vi "Tracker_2.2+.vi"(8 "error in (no error)":errorcluster, 11 "Settings file path":path=path "D:/Users/Dmitriy/CData/CloudStation/Tracker_repository/SubVi's/Tracker_settings.tcf") -> (0 "error out":errorcluster)   [LabVIEW 2018]
uses:
  <vilib>/Utility/miscctls.llb/LVPointTypeDef.ctl
  <vilib>/Utility/config.llb/NI_LVConfig.lvlib
  SubVi's/SW_Globals.vi
  <vilib>/Utility/file.llb/Write Delimited Spreadsheet (string).vi
  <vilib>/Utility/miscctls.llb/LVRangeTypeDef.ctl
  <extravilib>/ChannelInstances/Lossy Stream-a[.,.](str).lvlib
  <vilib>/Instr/_visa.llb/VISA Flush IO Buffer Mask.ctl
  <vilib>/Utility/miscctls.llb/LVBoundsTypeDef.ctl
  <vilib>/Utility/miscctls.llb/LVOffsetAndMultiplierTypeDef.ctl
  <vilib>/platform/TimedLoop/XDataNode/XDataNode.xnode
  <vilib>/Platform/TimedLoop/XDataNode/nitl_modes.ctl
  <vilib>/Platform/TimedLoop/XDataNode/XDNodeRunTimeDep.lvlib
  <vilib>/Platform/TimedLoop/XDataNode/wakeup.ctl
  <vilib>/Platform/TimedLoop/XDataNode/timing_clust.ctl
  <vilib>/Analysis/NI_AALBase.lvlib
  <vilib>/Instr/_visa.llb/VISA Open Access Mode.ctl
  <vilib>/Utility/sysdir.llb/System Directory Type.ctl
  <vilib>/ChannelSupport/Lossy Behavior.ctl
  <extravilib>/ChannelInstances/Stream-a[.](str).lvlib
  <vilib>/Utility/file.llb/Write Delimited Spreadsheet (I64).vi
  <vilib>/Platform/TimedLoop/scheduler/LVUserAPI/_suppVIs/Create_1kHz_TSource.vi
  <vilib>/Utility/file.llb/Read Delimited Spreadsheet (string).vi
  <vilib>/Utility/config.llb/Config Data RefNum.ctl
  <vilib>/Utility/miscctls.llb/LVPoint32TypeDef.ctl
  SubVi's/CTL_Data_flow_control_cluster.ctl
panel:
  out "Timed structure (Streaming) and VISA error(s)":errorcluster
  out "VISA streaming error out":errorcluster
  out "Latest frame":string[](array[string])
  out "Serial port opened":bool
  in  "Open serial port":bool
  out "FP size change error":errorcluster
  out "FPS status":i32=80
  out "Data flow controls":T1
  in  "Streaming":bool
  out "write status":bool
  out "Last send packet size, bytes":u32
  out "PP status":string
  out "DAQ status":string
  out "Stop TTL is fired":bool
  out "Start TTL is fired":bool
  out "IO paramaters loaded from file":bool
  out "IO parameters loaded cluster":T2
  out "Settings load path":path caption="selected path"
  in  "\"Stop at\" enabled":bool
  in  "Serial OUT name":refnum<visa-resource-name>="Serial_Output"
  out "Output to the external terminal":string="00:00:00.000\t0.000000\t0.000000\t0.000000\t0.000000\t00.000000\t0.000000\t0\t0.000\r\n"
  in  "Twisted neck":bool
  in  "Bridge horizontal offset":sgl min=-70 max=70 step=0.1 format="%#.1g"
  in  "Name Prefix":string="SavedTrack"
  in  "Stop record at":dbl=600.0 caption="Stop at" min=0.0 max=43200.0 step=60.0 format="%<%H:%M:%S>t"
  out "Adv. Stim. set":bool
  in  "Save files First Call":bool=TRUE
  in  "Record start First Call":bool=TRUE
  out "Time per sample mean":dbl format="%0.2f"
  out "Time per sample SD":dbl format="%0.2f"
  out "Save iteration duration":i64
  out "standard deviation":dbl format="%0.2f"
  out "mean":dbl format="%0.2f"
  in  "Type of histogram":u8
  out "TTL 4 counter":u32
  out "TTL 3 counter":u32
  out "TTL 2 counter":u32
  out "TTL 1 counter":u32
  out "Full track plotting":u32
  out "Full track preparation":u32
  out "Main queue":refnum<queue>
  in  "Map index (analysis)":i32
  in  "Full trace color":u32(colorbox)=16711680
  out "Current TTL status":u8
  out "TTL inputs":u8[](array[numeric])
  out "TTL outputs":u8[](array[numeric])
  out "Start/Stop in config":u32
  out "Start/Stop out pulses config":u32
  out "Changed IO":bool
  out "Sync capability":u8
  in  "IO parameters string":string
  out "Reset STIM":bool
  out "Reset REG":bool
  out "Init plot":bool=TRUE
  out "Zones preference array (loaded)":dbl[][](array[numeric])
  out "Current zone":dbl[](array[numeric])
  out "Absolute timestamp (rec)":dbl[](array[numeric])
  in  "Colors for Stim. setup":T3(array[cluster])=[{"Not Selected"=1143775, "Not Selected"=1143775}, {"Not Selected"=14517504, "Not Selected"=14517504}, {"Not Selected"=1976113, "Not Selected"=1976113}, {"Not Selected"=2575993, "Not Selected"=2575993}]
  out "Record":bool
  out "Stopped":bool
  out "Reset starting pulse":bool
  out "TTL is long enough":bool
  out "Started":bool
  out "Coords":T4={"Horizontal"=316, "Vertical"=127}
  out "Button":u16=1
  out "Settings file path":path
  out "Track path":path
  out "Index of the last recorded timepoint":i32
  out "ceil(x): smallest int >= x":dbl
  out "Application Directory":path
  out "Path to the settings file":path=path "D:/Users/Dmitriy/CData/CloudStation/Tracker_repository/Tracker_settings.tcf"
  out "Eff. save interval":sgl=7.981
  out "Relative timestamp (rec)":dbl[](array[numeric])
  out "alpha rot. angle":dbl[](array[numeric])
  out "Y coord":dbl[](array[numeric])
  out "X coord":dbl[](array[numeric])
  out "Zones allocation array":i32[](array[numeric])
  out "Zones presence array":bool[](array[boolean])
  in  "Stop Button":bool
  out "Path to the latest saved temp file":path
  out "Temp file ready":bool
  out "Pixels per mm":dbl=1.1663076923076923
  out "Settings file refnum out":T5
  out "Current User":string="Researcher"
  in  "Main tab control":enum32{"Settings", "Recording", "Analysis"}(tab)
  in  "Set advanced stimulus":bool
  in  "Load settings":bool
  out "IO status indicator":T6
  in  "Set IO config":bool
  in  "Jump to Analysis":bool
  in  "Reset stimuli":bool
  in  "Stimulus presets":T7(array[cluster]) {"TTL out" items=["1"=1, "2"=2, "1 + 2"=3]; "Stimulus, s" min=0 max=10000 step=0.1; "Time, s" min=0 max=10000 step=0.1; "Event type" items=["Time spent in zone", "Future options"]}
  in  "Zone-based stimulus setup":T8(radio)=enum."Zone 13"
  out "Ready":bool=TRUE
  in  "Re-check HW connection":bool
  in  "Reset regions":bool
  in  "Start Tracking button":bool
  in  "Starting angle BORDER":i16
  in  "N segments BORDER":u8=5 min=1 max=12
  in  "N segments MIDFIELD":u8=3 max=8
  in  "Starting angle MIDFIELD":i16=30
  in  "Radius, mm MIDFIELD":u16=110
  in  "Radius, mm CENTER":u16=50 min=5 step=1
  out "Board size":string="Large"
  in  "Cage diameter, mm":u16(ring)=333 items=["180 mm"=180, "240 mm"=240, "290 mm"=290, "325 mm"=325, "327 mm"=327, "333 mm"=333]
  out "Segments diagram":picture
  out "HW info":string
  out "Port":string="Large"
  in  "Expand/hide stream panel (Set)":bool
  out "Run times distrib. indicator":bool
  out "IO pulses count":string
  in  "Bridge swap":bool
  in  "Reset barplot":bool
  out "Mouse speed digi":dbl=0.28949046360238656 caption="Mouse speed" format="%05.1f"
  out "Histograms (normalized)":dbl[](graph)=[0.0, 0.0, 0.0, 0.0, 0.0, 0.0, 0.0, 1.0, 0.0, 0.0, 0.0, 0.0, 0.0, 0.0] caption="Zone preference (normalized)"
  in  "Multiplyer of chart RX":u8(slide)=1 min=1 max=10 step=1 scale=1.0..6.0
  in  "Zones presence indicator":T9={"01"=TRUE, "02"=TRUE, "03"=TRUE, "04"=TRUE, "05"=TRUE, "06"=TRUE, "07"=TRUE, "08"=TRUE, "09"=TRUE, "10"=TRUE, "11"=TRUE, "12"=TRUE, "13"=TRUE}
  in  "Zones":bool=TRUE
  in  "Record/Stop":bool
  out "Diagram at recording":picture caption="Mouse track"
  in  "Trace, s":u16(slide)=5 max=30 step=1 scale=0.0..30.0
  in  "Data filtering":u16(ring)=5 items=["None"=0, "Kalman 1/3"=2, "Kalman 1/8"=3, "SG 3/5"=4, "SG 3/11"=5, "SG 3/31"=6]
  out "Record timestamp":dbl format="%<%H:%M:%S%3u>t"
  out "Current Time":timestamp=timestamp(3610093053.229 s since 1904-01-01) format="%<%H:%M:%S %d.%m.%Y>T"
  in  "Exit (recording)":bool
  out "Mouse speed":waveform(dbl)(graph)={"t0"=timestamp(3610093053.229 s since 1904-01-01), "dt"=1.0, "Y"=[0.28949046360238656]}
  in  "Bridge offset":sgl min=-70 max=70 step=0.1 format="%#.1g"
  out "TTL IO 1 (recording)":bool caption="IO 1"
  out "TTL IO 2 (recording)":bool caption="IO 2"
  out "TTL IO 3 (recording)":bool caption="IO 3"
  out "TTL IO 4 (recording)":bool caption="IO 4"
  out "TTL REC":bool
  out "Mouse running, perc. of time":dbl=0.28949046360238656 caption="Run, %" format="%05.2f"
  out "Zones presense indicator":bool=TRUE
  out "Speed distrib. indicator":bool
  out "Run lengts distrib. indicator":bool
  in  "Additional record settings":bool caption="Add. recording settings"
  in  "Expand/hide stream panel (Rec)":bool
  in  "Back to Settings":bool
  out "Data loading progress":dbl(slide) scale=0.0..100.0
  in  "Speed":u16(ring)=3 items=["25"=75, "10"=30, "6"=18, "4"=12, "2"=6, "1"=3, "2/3"=2, "1/3"=1]
  in  "Timeline":dbl(slide) min=0.0 step=1.0 scale=0.0..2351.728 scale format="%<%H:%M:%S>t"
  in  "Multiplyer of chart RX 2":u8(slide)=1 min=1 max=10 step=1 scale=1.0..6.0
  out "Diagram at analysis":picture caption="Mouse track"
  in  "Play/Pause":bool
  out "Recorded at time":timestamp format="%<%H:%M:%S %d.%m.%Y>T"
  out "Recorded timestamp":dbl format="%<%H:%M:%S%3u>t"
  in  "Zones (analysis)":bool=TRUE caption="Zones"
  out "Mouse speed 2":waveform(dbl)(graph) caption="Mouse speed"
  out "Mouse speed digi 2":dbl format="%05.1f"
  out "Zones allocation (normalized) in analysis":dbl[](graph) caption="Zone preference (normalized)"
  out "Recorded by":string
  in  "Trace in analysis, s":u16(slide)=2 caption="Trace, s" max=30 step=1 scale=0.0..30.0
  in  "Open File":bool
  out "Bridge swap (analysis)":bool caption="Swapped"
  in  "Show heatmap (analysis)":bool caption="Heat map"
  in  "Show full track (analysis)":bool caption="Full track"
  out "Bridge Vertical offset (analysis)":sgl caption="Br. offset" min=-60 max=60 step=0.1 format="%#.1g"
  out "TTL IO 2 (analysis)":bool
  out "TTL IO 1 (analysis)":bool
  out "TTL IO 3 (analysis)":bool
  out "TTL IO 4 (analysis)":bool
  in  "Expand/hide stream panel (An)":bool
  # "v.2.1.9.9"
  # "Cage segmentation"
  # "BORDER"
  # "CENTER"
  # "MIDFIELD"
  # "v.2.1.9.9"
  # "v.2.1.9.9"
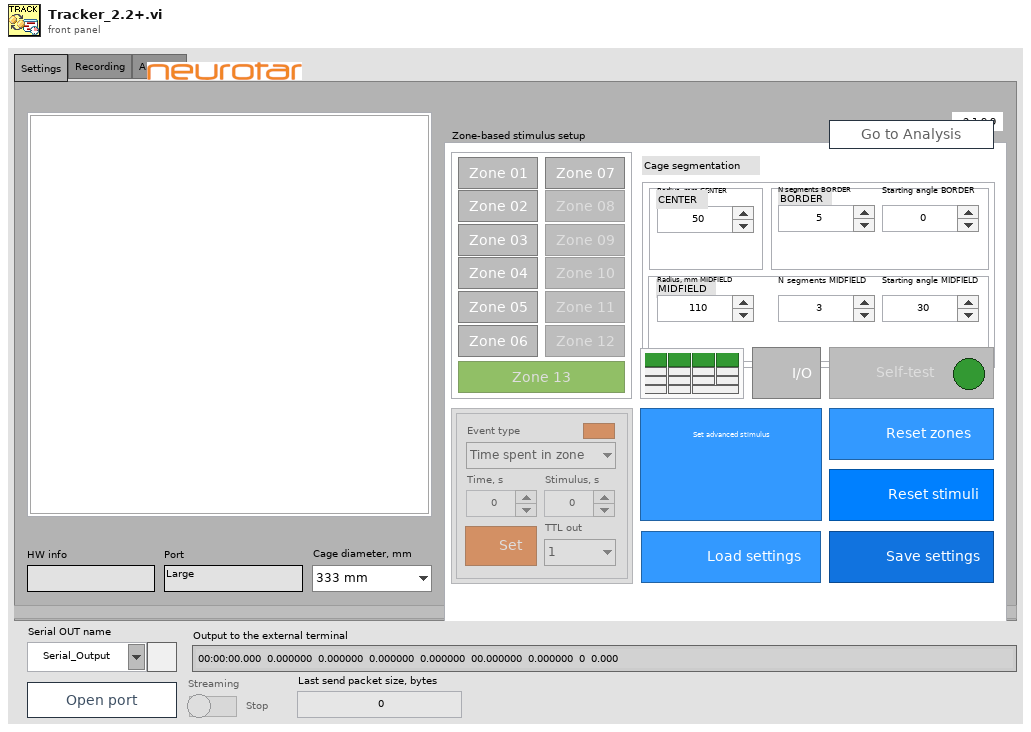
[diagram p1: front panel]
types:
  T1 = typedef "CTL_Data_flow_control_cluster.ctl" = cluster{"Data acquisition status":refnum<notifier>, "Play/Pause status":refnum<notifier>, "Complete stop":refnum<notifier>, "Temp file ready for processing":refnum<notifier>, "Has been recorded":refnum<notifier>, "Recording now":refnum<notifier>, "Path to the latest complete temp file":refnum<notifier>, "(Final) Data file is saved":refnum<notifier>, "Data loaded":refnum<notifier>}
  T2 = cluster{"SYNC configuration":u16, "IO 1 configuration":u16, "IO 2 configuration":u16, "IO 3 configuration":u16, "IO 4 configuration":u16, "Activate ext. RS-232":u16, "IO inversion config.":u16}
  T3 = cluster{"Not Selected":u32, "Not Selected":u32}[]
  T4 = typedef "LVPoint32TypeDef.ctl" = cluster{"Horizontal":i32, "Vertical":i32}
  T5 = typedef "NI_LVConfig.lvlib/Config Data RefNum.ctl" = refnum<k1>
  T6 = cluster{"IO1":bool, "IO2":bool, "IO3":bool, "IO4":bool, "Z1":bool, "Z2":bool, "Z3":bool, "Z4":bool, "St1":bool, "St2":bool, "St3":bool, "St4":bool, "Syn1":bool, "Syn2":bool, "RS-232 ext. activated":bool}
  T7 = cluster{"Event type":u16, "Time, s":sgl, "Stimulus, s":sgl, "Set/Clear":bool, "TTL out":u16, "Stim. has been set":bool}[]
  T8 = enum32{"No Selection", "Zone 01", "Zone 02", "Zone 03", "Zone 04", "Zone 05", "Zone 06", "Zone 07", "Zone 08", "Zone 09", "Zone 10", "Zone 11", "Zone 12", "Zone 13"}
  T9 = cluster{"01":bool, "02":bool, "03":bool, "04":bool, "05":bool, "06":bool, "07":bool, "08":bool, "09":bool, "10":bool, "11":bool, "12":bool, "13":bool}
  T10 = cluster{"SG coefficients 3/5":cluster{"0th order SG coefficients":dbl[], "1st order SG coefficients":dbl[]}, "SG coefficients 3/11":cluster{"0th order SG coefficients":dbl[], "1st order SG coefficients":dbl[]}, "SG coefficients 3/31":cluster{"0th order SG coefficients":dbl[], "1st order SG coefficients":dbl[]}, "SG coefficients 3/51":cluster{"0th order SG coefficients":dbl[], "1st order SG coefficients":dbl[]}}
  T11 = cluster{"Numeric Control":u32, "Numeric Control":u32}[]
  T12 = enum8{"Enabled", "Disabled", "Disabled and Grayed Out"}
  T13 = typedef "XDNodeRunTimeDep.lvlib/timing_clust.ctl" = cluster{"Expected End [f-1]":u64, "Actual End [f-1]":u64, "Finished Late? [f-1]":bool, "Expected End [i-1]":u64, "Actual End [i-1]":u64, "Finished Late? [i-1]":bool, "Expected Start [i]":u64, "Actual Start [i]":u64, "Expected Start [f]":u64, "Actual Start [f]":u64, "Source Name":string, "Structure Name":string, "Period":i64, "Deadline":i64, "Offset":i64, "Start":i64, "Priority":i32, "Timeout":i32, "Mode":T14, "Wakeup Reason":T15, "Error":errorcluster, "Source Type":string, "Secondary Source Type":string, "Global End Time":u64, "Global Start Time":u64, "Frame Duration":u64, "Iteration Duration":u64, "Assigned CPU":i32, "I/O Scan Engine Mode":u32}
  T14 = typedef "XDNodeRunTimeDep.lvlib/nitl_modes.ctl" = enum32{"No Change", "Process missed periods, maintain original phase", "Discard missed periods, maintain original phase", "Process missed periods, ignore original phase", "Discard missed periods, ignore original phase"}
  T15 = typedef "XDNodeRunTimeDep.lvlib/wakeup.ctl" = enum32{"Normal", "Aborted", "Asynchronous wakeup", "Timing source error", "Timed loop error", "Timeout"}
  T16 = cluster{"Read buffer":string, "Timestamp":timestamp}
  T17 = cluster{"Data acquisition status":refnum<notifier>, "Play/Pause status":refnum<notifier>, "Complete stop":refnum<notifier>, "Temp file ready for processing":refnum<notifier>, "Has been recorded":refnum<notifier>, "Recording now":refnum<notifier>, "Path to the latest complete temp file":refnum<notifier>, "Final CSV saved":refnum<notifier>, "Data loaded":refnum<notifier>}
  T18 = typedef "VISA Flush IO Buffer Mask.ctl" = u16
  T19 = typedef "LVBoundsTypeDef.ctl" = cluster{"Width":u32, "Height":u32}
  T20 = cluster{"Amount of border segments":u8, "Border segments starting angle":i16, "Amount of midfield segments":u8, "Midfield segments starting angle":i16, "Midfield segments outer radius, mm":u16, "Amount of central segments":u8, "Center segment outer radius, mm":u16, "Diameter of the cage, mm":u16, "R-gap between segments, mm":u8}
  T21 = typedef "LVRangeTypeDef.ctl" = cluster{"Minimum":dbl, "Maximum":dbl, "Increment":dbl, "Minor Increment":dbl, "Start":dbl}
  T22 = cluster{"Temporary file output path":path, "Density map array output path":path, "Recording settings output path":path, "Density map picture output path":path, "Layout picture output path":path, "Path to the settings file":path, "Path to TDMS file":path, "TDMS file reference":refnum<k34>}
  T23 = cluster{"Zones preference array (loaded)":dbl[][], "TTL inputs":u8[], "TTL outputs":u8[], "Stimulus presets array (loaded)":cluster{"Event type":u16, "Time, s":sgl, "Stimulus, s":sgl, "Set/Clear":bool, "TTL out":u16, "Stim. has been set":bool}[], "Absolute timestamp":dbl[], "Relative timestamp":dbl[], "X coord":dbl[], "Y coord":dbl[], "alpha rot. angle":dbl[], "Current zone":dbl[], "Acquisition settings cluster out":cluster{"Researcher name":string, "N segments MIDFIELD":u8, "N segments BORDER":u8, "Radius, mm CENTER":u16, "Radius, mm MIDFIELD":u16, "Starting angle MIDFIELD":i16, "Starting angle BORDER":i16, "Cage diameter, mm":u16, "Bridge swap":bool, "Bridge V. offset":sgl, "Twisted neck":bool, "Offset H.":sgl, "Name prefix":string, "Stop at":dbl, "\"Stop at\" enabled":bool, "Settings loaded OK":bool}, "Data column names":string[]}
  T24 = cluster{"Absolute timestamp (DBL)":dbl[], "Relative timestamp (DBL)":dbl[], "Zones normalized allocation array":dbl[][], "Coordinates and speed":dbl[][], "Current zone and TTLs":u8[][], "Acquisition settings cluster out":cluster{"Researcher name":string, "N segments MIDFIELD":u8, "N segments BORDER":u8, "Radius, mm CENTER":u16, "Radius, mm MIDFIELD":u16, "Starting angle MIDFIELD":i16, "Starting angle BORDER":i16, "Cage diameter, mm":u16, "Bridge swap":bool, "Bridge V. offset":sgl, "Twisted neck":bool, "Offset H.":sgl, "Name prefix":string, "Stop at":dbl, "\"Stop at\" enabled":bool, "Settings loaded OK":bool}, "Stimulus presets array":cluster{"Event type":u16, "Time, s":sgl, "Stimulus, s":sgl, "Set/Clear":bool, "TTL out":u16, "Stim. has been set":bool}[]}
  T25 = cluster{"Researcher name":string, "N segments MIDFIELD":u8, "N segments BORDER":u8, "Radius, mm CENTER":u16, "Radius, mm MIDFIELD":u16, "Starting angle MIDFIELD":i16, "Starting angle BORDER":i16, "Cage diameter, mm":u16, "Bridge swap":bool, "Bridge V. offset":sgl, "Twisted neck":bool, "Offset H.":sgl, "Name prefix":string, "Stop at":dbl, "\"Stop at\" enabled":bool, "Settings loaded OK":bool}
  T26 = typedef "imagedata.ctl" = cluster{"image type":i32, "image depth":i32, "image":u8[], "mask":u8[], "colors":u32[], "Rectangle":cluster{"left":i16, "top":i16, "right":i16, "bottom":i16}}
  T27 = cluster{"Fonts scale factor":dbl, "Pixels per mm":dbl, "Radius of displayed outer segments, pix":dbl, "Radius of displayed midfield segments, pix":dbl, "Radius of displayed central segment, pix":dbl}
  T28 = cluster{"Width":u16, "Style":enum32{"Solid", "Dash", "Dot", "DashDot", "DashDotDot"}}
  T29 = cluster{"N segments BORDER":u8, "Starting angle BORDER":i16, "N segments MIDFIELD":u8, "Starting angle MIDFIELD":i16, "Radius, mm MIDFIELD":u16, "Amount of central segments":u8, "Radius, mm CENTER":u16}
  T30 = typedef "LVOffsetAndMultiplierTypeDef.ctl" = cluster{"Offset":dbl, "Multiplier":dbl}
  T31 = enum32{"No Selection", "Zone 01", "Zone 02", "Zone 03", "Zone 04", "Zone 05", "Zone 06", "Zone 07", "Zone 08", "Zone 09", "Zone 10", "Zone 11", "Zone 12", "Zone 13", "Zone 14"}
  T32 = enum32{"Page Enabled", "Page Disabled", "Page Disabled & Grayed"}
  T33 = typedef "LVPointTypeDef.ctl" = cluster{"Horizontal":i16, "Vertical":i16}
  T34 = enum32{"invalid app kind", "Development System", "Run Time System", "Student Edition", "Embedded LabVIEW", "Evaluation", "Custom"}
  T35 = cluster{"Researcher name":string, "N segments MIDFIELD":u8, "N segments BORDER":u8, "Radius, mm CENTER":u16, "Radius, mm MIDFIELD":u16, "Starting angle MIDFIELD":i16, "Starting angle BORDER":i16, "Cage diameter, mm":u16, "Bridge swap":bool, "Bridge V. offset":sgl, "Twisted neck":bool, "Offset H.":sgl, "Name prefix":string, "Stop at":dbl, "\"Stop at\" enabled":bool, "Data filtering":u16, "Settings loaded OK":bool}
  T36 = cluster{"Event type":u16, "Dur., s":sgl, "Stim., s":sgl, "Set/Clear":bool, "TTL out N":u16, "Stim. has been set":bool}[]
  T37 = cluster{"0th order SG coefficients":dbl[], "1st order SG coefficients":dbl[]}
  T38 = typedef "Lossy Behavior.ctl" = enum16{"drop oldest element", "skip this write"}
  T39 = cluster{"Offset V.":sgl, "Offset H.":sgl, "Bridge swap":bool, "Turn magnets 90 deg.":bool, "Twisted neck":bool}
  T40 = typedef "Stream-a[.](str).lvlib/)Channel.ctl" = refnum<queue>
  T41 = typedef "Lossy Stream-a[.,.](str).lvlib/)Channel.ctl" = refnum<queue>
  T42 = cluster{"Read buffer":string, "Timestamp":timestamp}[]
  T43 = typedef "LVRectTypeDef.ctl" = cluster{"Left":i16, "Top":i16, "Right":i16, "Bottom":i16}
  T44 = typedef "VISA Open Access Mode.ctl" = u32
  T45 = cluster{"Event type":u16, "Cond., s":sgl, "Stim., s":sgl, "Set/Clear":bool, "TTL out N":u16, "Stim. has been set":bool}
  T46 = cluster{"Offset V.":sgl, "Offset H.":sgl, "Bridge swap":bool, "Twisted neck":bool, "Name prefix":string, "Stop at":dbl, "\"Stop at\" enabled":bool}
  T47 = cluster{"N segments BORDER":u8, "Starting angle BORDER":i16, "N segments MIDFIELD":u8, "Starting angle MIDFIELD":i16, "Radius, mm MIDFIELD":u16, "Amount of central segments":u8, "Radius, mm CENTER":u16, "Bridge swap":bool, "Bridge V. offset":sgl, "Twisted neck":bool, "Offset H.":sgl, "Zones configuration":string[], "IO parameters string":string, "Cage diameter, mm":u16, "Name prefix":string, "Stop at":dbl, "\"Stop at\" enabled":bool, "Data filtering":u16}
  T48 = cluster{"SYNC configuration":bool, "IO 1 configuration":bool, "IO 2 configuration":bool, "IO 3 configuration":bool, "IO 4 configuration":bool, "Activate ext. RS-232":bool, "IO inversion config.":bool}
  T49 = cluster{"Event type":u16, "Cond., s":sgl, "Stim., s":sgl, "Set/Clear":bool, "TTL out N":u16, "Stim. has been set":bool}[]
  T50 = cluster{"Event type":u16, "Time, s":sgl, "Stimulus, s":sgl, "Set/Clear":bool, "TTL out":u16, "Stim. has been set":bool}
  T51 = typedef "System Directory Type.ctl" = i32
  T52 = cluster{"N segments BORDER":u8, "Starting angle BORDER":i16, "N segments MIDFIELD":u8, "Starting angle MIDFIELD":i16, "Radius, mm MIDFIELD":u16, u8, "Radius, mm CENTER":u16, "Cage diameter, mm":u16, i32}
  T53 = cluster{"N segments BORDER":u8, "Starting angle BORDER":i16, "N segments MIDFIELD":u8, "Starting angle MIDFIELD":i16, "Radius, mm MIDFIELD":u16, "N segments CENTER":u8, "Radius, mm CENTER":u16, "Cage diameter, mm":u16, "R-gap":i32}
  T54 = cluster{"Zone[1]":bool, "Zone[2]":bool, "Zone[3]":bool, "Zone[4]":bool, "Zone[5]":bool, "Zone[6]":bool, "Zone[7]":bool, "Zone[8]":bool, "Zone[9]":bool, "Zone[10]":bool, "Zone[11]":bool, "Zone[12]":bool, "Zone[13]":bool}
  T55 = typedef "LVStringsAndValuesArrayTypeDef_U16.ctl" = cluster{"String":string, "Value":u16}[]
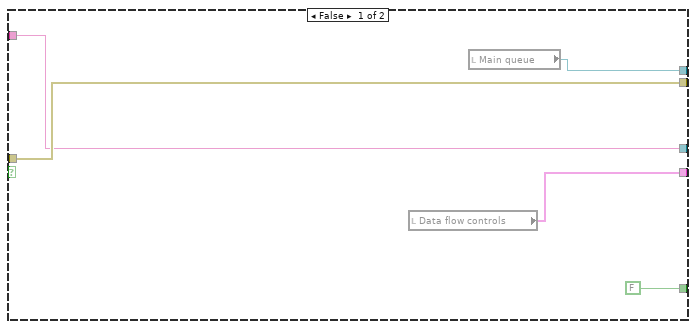
[diagram p2: hidden frame]
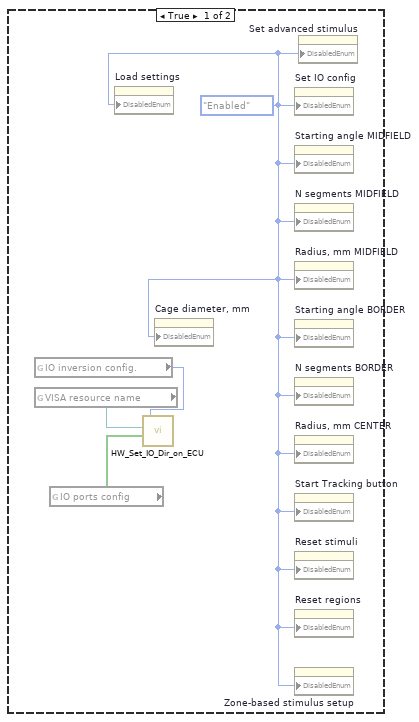
[diagram p3: hidden frame]
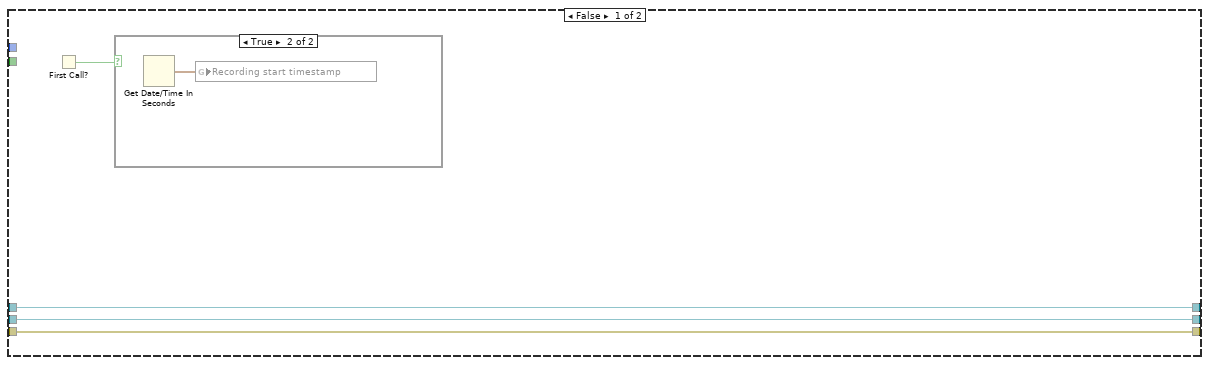
[diagram p10: hidden frame]
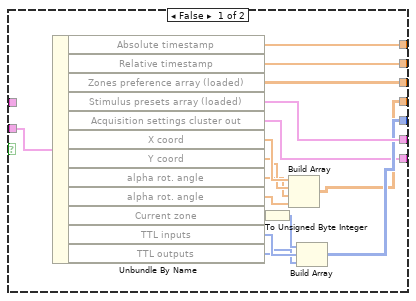
[diagram p20: hidden frame]
diagram:
  w6 = u16 3 items=["3/5", "3/11", "3/31", "3/51"] ("Select filter length")
  w8 = u16 2 items=["3/5", "3/11", "3/31", "3/51"] ("Select filter length")
  w12 = u16 1 items=["3/5", "3/11", "3/31", "3/51"] ("Select filter length")
  w16 = u16 0 items=["3/5", "3/11", "3/31", "3/51"] ("Select filter length")
  n1 = disable-structure shown="Disabled" {
    disable-tunnel: w26 -> [w43 _]
    disable-tunnel: [w42 _] -> w23
    disable-tunnel: [w31 _] -> w20
    disable-tunnel: [w30 _] -> w18
    disable-tunnel: w3 -> [w28 _]
    disable-tunnel: [w27 _] -> w2
    frame Disabled {
      n2 = disable-structure shown="Default" {
        disable-tunnel: [w109] -> w32
        frame Enabled {
          w108 = T12."Disabled and Grayed Out" ("Disabled")
          n3 = property on="Cage diameter, mm" class="Ring (strict)"("DisabledEnum"=w108) -> ()  [unwired: 2 in, 2 out]
          n4 = property on="Load settings" class="Bool (strict)"("DisabledEnum"=w108) -> ()  [unwired: 2 in, 2 out]
          n5 = property on="Set IO config" class="Bool"("DisabledEnum"=w108) -> ()  [unwired: 2 in, 2 out]
          n6 = property on="Starting angle MIDFIELD" class="DigNum (strict)"("DisabledEnum"=w108) -> ()  [unwired: 2 in, 2 out]
          n7 = property on="N segments MIDFIELD" class="DigNum (strict)"("DisabledEnum"=w108) -> ()  [unwired: 2 in, 2 out]
          n8 = property on="Radius, mm MIDFIELD" class="DigNum (strict)"("DisabledEnum"=w108) -> ()  [unwired: 2 in, 2 out]
          n9 = property on="Starting angle BORDER" class="DigNum (strict)"("DisabledEnum"=w108) -> ()  [unwired: 2 in, 2 out]
          n10 = property on="N segments BORDER" class="DigNum (strict)"("DisabledEnum"=w108) -> ()  [unwired: 2 in, 2 out]
          n11 = property on="Radius, mm CENTER" class="DigNum (strict)"("DisabledEnum"=w108) -> ()  [unwired: 2 in, 2 out]
          n12 = property on="Start Tracking button" class="Bool"("DisabledEnum"=w108) -> ()  [unwired: 2 in, 2 out]
          n13 = property on="Reset stimuli" class="Bool (strict)"("DisabledEnum"=w108) -> ()  [unwired: 2 in, 2 out]
          n14 = property on="Reset regions" class="Bool (strict)"("DisabledEnum"=w108) -> (error out=w109:errorcluster)  [unwired: 2 in, 1 out]
          n15 = property on="Zone-based stimulus setup" class="RadioBtnsControl (strict)"("DisabledEnum"=w108) -> ()  [unwired: 2 in, 2 out]
          n16 = property on="Set advanced stimulus" class="Bool (strict)"("DisabledEnum"=w108) -> ()  [unwired: 2 in, 2 out]
        }
      }
      n17 = property on="Re-check HW connection" class="Bool"(error in=w32, "DisabledEnum"=T12."Disabled and Grayed Out" ("Disabled")) -> (error out=w40:errorcluster)  [unwired: 1 in, 1 out]
      n18 = property on="Ready" class="Bool (strict)"(error in=w40, "Value"=FALSE ("Ready"), "Colors [4]"=T11 [{"Numeric Control"=16749459, "Numeric Control"=16749459}, {"Numeric Control"=1988894, "Numeric Control"=3381555}, {"Numeric Control"=4934475, "Numeric Control"=7895160}, {"Numeric Control"=994319, "Numeric Control"=1657881}]) -> (error out=w29:errorcluster)  [unwired: 1 in, 1 out]
      n19 = node-c288(w28, i64 1201 ("Period"), 50 ("Priority")) -> (w45:T13)
      n20 = timed-loop {
        tunnel: w43 -> [w65]
        tunnel: [w48] -> w33
        tunnel: [w64] -> w31
        tunnel: [w49] -> w42
        tunnel: [w63] -> w27
        tunnel: w29 -> [w59]
        tunnel: [w52] -> w36
        timing: w45 -> [_]
        timing-out: [_] -> w44
        stop <- w47 stop-if-true
        n21 = node-c288() -> ()  [unwired: 1 in, 1 out]
        n22 = property on="Re-check HW connection" class="Bool"(error in=w59, "DisabledEnum"=T12."Enabled" ("Disabled")) -> (error out=w58:errorcluster)  [unwired: 1 in, 1 out]
        n23 = First Call?() -> (First Call?: T/F=w50:bool)
        n24 = property on="Ready" class="Bool (strict)"(error in=w58) -> (error out=w62:errorcluster, "Value"=w61:bool)  [unwired: 1 in, 1 out]
        n25 = Or(x=w50, y="Re-check HW connection") -> (x .or. y?=w51:bool)
        n26 = Not(x=w61) -> (.not. x?=w57:bool)
        n27 = And(x=w57, y=w51) -> (x .and. y?=w56:bool)
        n28 = case shown="True" w56 {
          tunnel: w65 -> [w71 w101]
          tunnel: [w69 w100] -> w64
          tunnel: [w71 w99] -> w49
          tunnel: [w68 w98] -> w63
          tunnel: [w72 w73] -> w53
          tunnel: [FALSE ("Instrument OK?") w88] -> w48
          tunnel: w62 -> [w72 w76]
          frame False {
            n29 = local read "Data flow controls"() -> (w68:T1)
            n30 = local read "Main queue"() -> (w69:refnum<queue>)
          }
          frame True {
            w97 = T16 {"Read buffer"="", "Timestamp"=timestamp(3605695211.9516535 s since 1904-01-01)}  # Data frame example
            n31 = call <vilib>:"Set Busy.vi"("error in (no error)"=w76) -> ("error out"=w75:errorcluster)  [unwired: 9 in, 1 out]
            n32 = property on="Ready" class="Bool (strict)"(error in=w75, "Colors [4]"=T11 [{"Numeric Control"=16749459, "Numeric Control"=16176658}, {"Numeric Control"=1988894, "Numeric Control"=3381555}, {"Numeric Control"=4934475, "Numeric Control"=7895160}, {"Numeric Control"=994319, "Numeric Control"=1657881}]) -> (error out=w86:errorcluster)  [unwired: 1 in, 1 out]
            n33 = Obtain Queue(name (unnamed)="Data flow", element data type=w97, error in (no error)=w86) -> (queue out=w100:refnum<queue>, error out=w95:errorcluster)  [unwired: 2 in, 1 out]
            "Main queue" <- w100
            n34 = call "HW_Setup.vi"("error in"=w95, "Traget FPS"=80, "VISA resource name in"=w101) -> ("FPS status"=→"FPS status":i32, "Instrument OK?"=w88:bool, "Data flow controls"=w98:T1, "VISA resource name out"=w99:refnum<visa-resource-name>, "Version information"=w85:string, "Sensor board size"=w78:string, "error out"=w74:errorcluster)  [unwired: 1 in, 1 out]
            "Ready" <- w88
            "Board size" <- w78
            "Data flow controls" <- w98
            n35 = String Length(string=w85) -> (length=w92:i32)
            n36 = Equal?(x=w85, y="1.1.4") -> (x = y?=w82:bool)
            n37 = Greater Than 0?(x=w92) -> (x > 0?=w91:bool)
            n38 = Concatenate Strings(w78, ", FW: " ("string"), w85) -> (w90:string)
            n39 = Select(t=u8 0, s=w82, f=u8 1) -> (s? t:f=→"Sync capability":u8)
            n40 = Select(t=w90, s=w91, f="Not connected") -> (s? t:f=→"HW info":string)
            n41 = call <vilib>:"Unset Busy.vi"("error in (no error)"=w74) -> ("error out"=w73:errorcluster)  [unwired: 10 in]
          }
        }
        n42 = property on="Jump to Analysis" class="Bool (strict)"() -> ("Value"=w46:bool)  [unwired: 2 in, 2 out]
        n43 = Or(x=w48, y=w46) -> (x .or. y?=w47:bool)
        n44 = global write "SW_Globals.vi" "VISA resource name"(w49) -> ()
        n45 = property on="Ready" class="Bool (strict)"(error in=w53, "Colors [4]"=T11 [{"Numeric Control"=16749459, "Numeric Control"=16749459}, {"Numeric Control"=1988894, "Numeric Control"=3381555}, {"Numeric Control"=4934475, "Numeric Control"=7895160}, {"Numeric Control"=994319, "Numeric Control"=1657881}]) -> (error out=w52:errorcluster)  [unwired: 1 in, 1 out]
        n46 = node-c288() -> ()  [unwired: 1 in, 1 out]
      }
      n47 = node-c288(w44) -> ()  [unwired: 1 out]
      n48 = property on="Re-check HW connection" class="Bool"(error in=w36, "DisabledEnum"=T12."Disabled and Grayed Out" ("Disabled")) -> (error out=w30:errorcluster)  [unwired: 1 in, 1 out]
      n49 = case shown="False" w33 {
        frame True {
          w110 = T12."Enabled" ("Disabled")
          n50 = global read "SW_Globals.vi" "IO inversion config."() -> (w111:u16)
          n51 = global read "SW_Globals.vi" "VISA resource name"() -> (w113:refnum<visa-resource-name>)
          n52 = global read "SW_Globals.vi" "IO ports config"() -> (w112:bool[])
          n53 = property on="Load settings" class="Bool (strict)"("DisabledEnum"=w110) -> ()  [unwired: 2 in, 2 out]
          n54 = call "HW_Set_IO_Dir_on_ECU.vi"("IO ports config"=w112, "VISA resource name"=w113, "IO inversion config."=w111) -> ()  [unwired: 1 in, 2 out]
          n55 = property on="Cage diameter, mm" class="Ring (strict)"("DisabledEnum"=w110) -> ()  [unwired: 2 in, 2 out]
          n56 = property on="Set IO config" class="Bool"("DisabledEnum"=w110) -> ()  [unwired: 2 in, 2 out]
          n57 = property on="Starting angle MIDFIELD" class="DigNum (strict)"("DisabledEnum"=w110) -> ()  [unwired: 2 in, 2 out]
          n58 = property on="N segments MIDFIELD" class="DigNum (strict)"("DisabledEnum"=w110) -> ()  [unwired: 2 in, 2 out]
          n59 = property on="Radius, mm MIDFIELD" class="DigNum (strict)"("DisabledEnum"=w110) -> ()  [unwired: 2 in, 2 out]
          n60 = property on="Starting angle BORDER" class="DigNum (strict)"("DisabledEnum"=w110) -> ()  [unwired: 2 in, 2 out]
          n61 = property on="N segments BORDER" class="DigNum (strict)"("DisabledEnum"=w110) -> ()  [unwired: 2 in, 2 out]
          n62 = property on="Radius, mm CENTER" class="DigNum (strict)"("DisabledEnum"=w110) -> ()  [unwired: 2 in, 2 out]
          n63 = property on="Start Tracking button" class="Bool"("DisabledEnum"=w110) -> ()  [unwired: 2 in, 2 out]
          n64 = property on="Reset stimuli" class="Bool (strict)"("DisabledEnum"=w110) -> ()  [unwired: 2 in, 2 out]
          n65 = property on="Reset regions" class="Bool (strict)"("DisabledEnum"=w110) -> ()  [unwired: 2 in, 2 out]
          n66 = property on="Zone-based stimulus setup" class="RadioBtnsControl (strict)"("DisabledEnum"=w110) -> ()  [unwired: 2 in, 2 out]
          n67 = property on="Set advanced stimulus" class="Bool (strict)"("DisabledEnum"=w110) -> ()  [unwired: 2 in, 2 out]
        }
        frame False {
          w114 = T12."Disabled and Grayed Out" ("Disabled")
          n68 = disable-structure shown="Disabled" {
            disable-tunnel: w114 -> [w115 _]
            frame Disabled {
              n69 = property on="Load settings" class="Bool (strict)"("DisabledEnum"=w115) -> ()  [unwired: 2 in, 2 out]
            }
            frame Enabled {
            }
          }
          n70 = property on="Set advanced stimulus" class="Bool (strict)"("DisabledEnum"=w114) -> ()  [unwired: 2 in, 2 out]
          n71 = property on="Cage diameter, mm" class="Ring (strict)"("DisabledEnum"=w114) -> ()  [unwired: 2 in, 2 out]
          n72 = property on="Set IO config" class="Bool"("DisabledEnum"=w114) -> ()  [unwired: 2 in, 2 out]
          n73 = property on="Starting angle MIDFIELD" class="DigNum (strict)"("DisabledEnum"=w114) -> ()  [unwired: 2 in, 2 out]
          n74 = property on="N segments MIDFIELD" class="DigNum (strict)"("DisabledEnum"=w114) -> ()  [unwired: 2 in, 2 out]
          n75 = property on="Radius, mm MIDFIELD" class="DigNum (strict)"("DisabledEnum"=w114) -> ()  [unwired: 2 in, 2 out]
          n76 = property on="Starting angle BORDER" class="DigNum (strict)"("DisabledEnum"=w114) -> ()  [unwired: 2 in, 2 out]
          n77 = property on="N segments BORDER" class="DigNum (strict)"("DisabledEnum"=w114) -> ()  [unwired: 2 in, 2 out]
          n78 = property on="Radius, mm CENTER" class="DigNum (strict)"("DisabledEnum"=w114) -> ()  [unwired: 2 in, 2 out]
          n79 = property on="Start Tracking button" class="Bool"("DisabledEnum"=w114) -> ()  [unwired: 2 in, 2 out]
          n80 = property on="Reset stimuli" class="Bool (strict)"("DisabledEnum"=w114) -> ()  [unwired: 2 in, 2 out]
          n81 = property on="Reset regions" class="Bool (strict)"("DisabledEnum"=w114) -> ()  [unwired: 2 in, 2 out]
          n82 = property on="Zone-based stimulus setup" class="RadioBtnsControl (strict)"("DisabledEnum"=w114) -> ()  [unwired: 2 in, 2 out]
          n83 = property on="Set advanced stimulus" class="Bool (strict)"("DisabledEnum"=w114) -> ()  [unwired: 2 in, 2 out]
        }
      }
    }
    frame Enabled {
    }
  }
  n84 = disable-structure shown="Disabled" {
    disable-tunnel: w23 -> [w122 _]
    disable-tunnel: w20 -> [w119 _]
    disable-tunnel: w18 -> [w118 _]
    disable-tunnel: w3 -> [w117 _]
    disable-tunnel: w2 -> [w116 _]
    frame Disabled {
      n85 = node-c288(w117, i64 1 ("Period"), 65000 ("Priority")) -> (w124:T13)
      n86 = timed-loop "In this loop raw data from the device is obtained and TTLs are fired" {
        tunnel: w122 -> [w147]
        tunnel: w118 -> [w146]
        tunnel: w116 -> [w126]
        tunnel: w119 -> [w151]
        timing: w124 -> [_]
        timing-out: [_] -> w123
        stop <- w128 stop-if-true
        # "In this loop raw data from the device is obtained and TTLs are fired"
        n87 = node-c288() -> (w145:i64)  [unwired: 1 in]
        n88 = Unbundle By Name(w126) -> ("Complete stop"=w135:refnum<notifier>, "Recording now"=w134:refnum<notifier>, "Has been recorded"=w133:refnum<notifier>)
        n89 = disable-structure shown="Disabled" {
          disable-tunnel: w145 -> [w183 _]
          frame Disabled {
            n90 = Build Array(w183) -> (w181:i64[])
            n91 = call "FL_Last_N_Samples_1D.vi"("BufferLengthSamples"=u32 500, "Input Array"=w181) -> ("Output Array"=w182:dbl[])
            n92 = call <vilib>:"Std Deviation and Variance.vi"("X"=w182) -> ("mean"=→"mean":dbl, "standard deviation"=→"standard deviation":dbl)  [unwired: 1 in, 1 out]
          }
          frame Enabled {
          }
        }
        n93 = property on="Start/Stop out pulses config" class="DigNum (strict)"() -> ("Value"=w148:u32)  [unwired: 2 in, 2 out]
        n94 = Get Notifier Status(notifier=w133) -> (current notification=w132:bool)  [unwired: 1 in, 4 out]
        n95 = Get Notifier Status(notifier=w135) -> (current notification=w128:bool)  [unwired: 1 in, 4 out]
        n96 = Get Notifier Status(notifier=w134) -> (current notification=w130:bool)  [unwired: 1 in, 4 out]
        n97 = Not(x=w130) -> (.not. x?=w129:bool)
        n98 = Greater Than 0?(x=w148) -> (x > 0?=w149:bool)
        n99 = And(x=w129, y=w132) -> (x .and. y?=w131:bool)
        n100 = case "Inside this case structure TTL can be fired at the start of the recording" shown="True" w130 {
          tunnel: w149 -> [_ w197]
          tunnel: w146 -> [w186 w196]
          tunnel: [w186 w195] -> w152
          tunnel: w147 -> [w187 w194]
          tunnel: [w187 w193] -> w154
          tunnel: [w185 w192] -> w153
          tunnel: w151 -> [w185 w191]
          tunnel: w148 -> [_ w190]
          frame False {
            n101 = First Call?() -> (First Call?: T/F=w184:bool)
            n102 = case shown="True" w184 {
              frame False {
              }
              frame True {
                n103 = Get Date/Time In Seconds() -> (seconds since 1Jan1904=w188:timestamp)
                n104 = global write "SW_Globals.vi" "Recording start timestamp"(w188) -> ()
              }
            }
          }
          frame True {
            n105 = property on="Start TTL is fired" class="Bool (strict)"() -> ("Value"=w189:bool)  [unwired: 2 in, 2 out]
            n106 = case shown="False" w189 {
              tunnel: w197 -> [w214 _]
              tunnel: w196 -> [w213 w256]
              tunnel: [w198 w256] -> w195
              tunnel: w194 -> [w212 w255]
              tunnel: [w211 w255] -> w193
              tunnel: [w209 w254] -> w192
              tunnel: w191 -> [w210 w254]
              tunnel: w190 -> [w201 _]
              tunnel: w190 -> [w200 _]
              frame False {
                n107 = flat-sequence {
                  tunnel: w210 -> [w227]
                  tunnel: w212 -> [w228]
                  tunnel: w213 -> [w225]
                  tunnel: w214 -> [w226]
                  tunnel: [w226] -> w208
                  tunnel: [w225] -> w207
                  tunnel: [w228] -> w206
                  tunnel: [w227] -> w205
                  tunnel: w200 -> [w215]
                  tunnel: [w233] -> w204
                  tunnel: [w238] -> w203
                  tunnel: [w237] -> w202
                  tunnel: w208 -> [w230]
                  tunnel: w207 -> [w236]
                  tunnel: w206 -> [w235]
                  tunnel: w205 -> [w239]
                  tunnel: w201 -> [w229]
                  tunnel: [w250] -> w198
                  tunnel: [w252] -> w209
                  tunnel: [w253] -> w211
                  tunnel: w202 -> [w250]
                  tunnel: w203 -> [w252]
                  tunnel: w204 -> [w253]
                  frame #0 {
                    n108 = Number To Boolean Array(number=w215) -> (Boolean array=w219:bool[])
                    n109 = Index Array(array=w219, index=3) -> (element=w221:bool)
                    n110 = Index Array(array=w219, index=2) -> (element=w222:bool)
                    n111 = Index Array(array=w219, index=1) -> (element=w223:bool)
                    n112 = Index Array(array=w219, index=0) -> (element=w224:bool)
                    n113 = property on="TTL IO 4 (recording)" class="Bool (strict)"("Value"=w221) -> ()  [unwired: 2 in, 2 out]
                    n114 = property on="TTL IO 3 (recording)" class="Bool (strict)"("Value"=w222) -> ()  [unwired: 2 in, 2 out]
                    n115 = property on="TTL IO 2 (recording)" class="Bool (strict)"("Value"=w223) -> ()  [unwired: 2 in, 2 out]
                    n116 = property on="TTL IO 1 (recording)" class="Bool (strict)"("Value"=w224) -> ()  [unwired: 2 in, 2 out]
                  }
                  frame #1 {
                    n117 = call "SW_Fire_TTL_at_start_universal.vi"("TTL port(s) config to fire"=w229, "TTL pulse length, ms"=100.0, "error in (no error)"=w236, "Serial Port In"=w235, "Close VISA (T)"=FALSE, "Start/stop signaling (F)"=w230) -> ("error out"=w234:errorcluster, "Serial Port Out"=w233:refnum<visa-resource-name>)  [unwired: 3 in, 1 out]
                    n118 = Flush Queue(queue=w239, error in (no error)=w234) -> (queue out=w238:refnum<queue>, error out=w237:errorcluster)  [unwired: 1 out]
                  }
                  frame #2 {
                    n119 = Get Date/Time In Seconds() -> (seconds since 1Jan1904=w251:timestamp)
                    n120 = Number To Boolean Array(number=u32 0) -> (Boolean array=w246:bool[])
                    n121 = global write "SW_Globals.vi" "Recording start timestamp"(w251) -> ()
                    n122 = Index Array(array=w246, index=2) -> (element=w243:bool)
                    n123 = Index Array(array=w246, index=1) -> (element=w242:bool)
                    n124 = Index Array(array=w246, index=0) -> (element=w241:bool)
                    n125 = Index Array(array=w246, index=3) -> (element=w244:bool)
                    n126 = property on="TTL IO 3 (recording)" class="Bool (strict)"("Value"=w243) -> ()  [unwired: 2 in, 2 out]
                    n127 = property on="TTL IO 2 (recording)" class="Bool (strict)"("Value"=w242) -> ()  [unwired: 2 in, 2 out]
                    n128 = property on="TTL IO 1 (recording)" class="Bool (strict)"("Value"=w241) -> ()  [unwired: 2 in, 2 out]
                    n129 = property on="TTL IO 4 (recording)" class="Bool (strict)"("Value"=w244) -> ()  [unwired: 2 in, 2 out]
                  }
                }
                n130 = property on="Start TTL is fired" class="Bool (strict)"(error in=w198, "Value"=TRUE ("Start TTL is fired")) -> ()  [unwired: 1 in, 2 out]
              }
              frame True {
              }
            }
          }
        }
        n131 = Or(x=w131, y=w128) -> (x .or. y?=w155:bool)
        n132 = disable-structure shown="Disabled" {
          disable-tunnel: w137 -> [w177 _]
          disable-tunnel: w136 -> [w176 _]
          frame Disabled {
            n133 = Subtract(x=w177, y=w176) -> (x-y=w171:dbl)
            n134 = Multiply(x=1000.0, y=w171) -> (x*y=w169:dbl)
            n135 = Build Array(w169) -> (w170:dbl[])
            n136 = call "FL_Last_N_Samples_1D.vi"("BufferLengthSamples"=u32 1000, "Input Array"=w170) -> ("Output Array"=w172:dbl[])
            n137 = call <vilib>:"Std Deviation and Variance.vi"("X"=w172) -> ("mean"=→"Time per sample mean":dbl, "standard deviation"=→"Time per sample SD":dbl)  [unwired: 1 in, 1 out]
          }
          frame Enabled {
          }
        }
        n138 = disable-structure shown="Disabled" {
          disable-tunnel: w126 -> [w164 _]
          frame Disabled {
            n139 = Unbundle By Name(w164) -> ("Data acquisition status"=w163:refnum<notifier>, "Play/Pause status"=w161:refnum<notifier>)
            n140 = Get Notifier Status(notifier=w163) -> (current notification=→"DAQ status":string)  [unwired: 1 in, 4 out]
            n141 = Get Notifier Status(notifier=w161) -> (current notification=→"PP status":string)  [unwired: 1 in, 4 out]
          }
          frame Enabled {
          }
        }
        n142 = flat-sequence {
          tunnel: w152 -> [w258]
          tunnel: w153 -> [w259]
          tunnel: w154 -> [w260]
          tunnel: w126 -> [w261]
          tunnel: [w261] -> w144
          tunnel: [w260] -> w143
          tunnel: [w259] -> w142
          tunnel: [w258] -> w141
          tunnel: [w257] -> w136
          tunnel: w144 -> [w267]
          tunnel: w143 -> [w264]
          tunnel: w142 -> [w263]
          tunnel: w141 -> [w262]
          tunnel: [w268] -> w140
          tunnel: [w266] -> w139
          tunnel: [w265] -> w138
          tunnel: [w270] -> w158
          tunnel: [w271] -> w159
          tunnel: [w272] -> _
          tunnel: w140 -> [w272]
          tunnel: w139 -> [w271]
          tunnel: w138 -> [w270]
          tunnel: [w269] -> w137
          frame #0 {
            n143 = call <vilib>:"High Resolution Relative Seconds.vi"() -> ("relative seconds"=w257:dbl)
          }
          frame #1 {
            n144 = call "HW_Stream_raw_data_enq.vi"("error in"=w262, "Queue in"=w263, "Data flow controls in"=w267, "VISA resource name in"=w264) -> ("error out"=w265:errorcluster, "Data flow controls out"=w268:T17, "VISA resource name out"=w266:refnum<visa-resource-name>)  [unwired: 4 in, 1 out]
          }
          frame #2 {
            n145 = call <vilib>:"High Resolution Relative Seconds.vi"() -> ("relative seconds"=w269:dbl)
          }
        }
        n146 = case "Inside this case structure TTL can be fired at the end of the recording" shown="True" w155 {
          selector: w155 -> [w297 w303]
          tunnel: w159 -> [w298 w306]
          tunnel: [w299 w308] -> w157
          tunnel: w158 -> [w299 w307]
          tunnel: [w298 w305] -> w156
          tunnel: w149 -> [_ w304]
          tunnel: [w297 w303] -> w150
          tunnel: w148 -> [_ w302]
          tunnel: w148 -> [_ w301]
          frame False {
          }
          frame True {
            n147 = property on="Stop TTL is fired" class="Bool (strict)"() -> ("Value"=w300:bool)  [unwired: 2 in, 2 out]
            n148 = case shown="False" w300 {
              tunnel: [w310 w356] -> w308
              tunnel: w307 -> [w321 w356]
              tunnel: w306 -> [w320 w355]
              tunnel: [w319 w355] -> w305
              tunnel: w304 -> [w318 _]
              tunnel: w302 -> [w311 _]
              tunnel: w301 -> [w312 _]
              frame False {
                n149 = flat-sequence {
                  tunnel: w318 -> [w333]
                  tunnel: w320 -> [w334]
                  tunnel: w321 -> [w332]
                  tunnel: [w332] -> w315
                  tunnel: [w334] -> w314
                  tunnel: [w333] -> w313
                  tunnel: w312 -> [w322]
                  tunnel: [w342] -> w317
                  tunnel: [w341] -> w316
                  tunnel: w315 -> [w339]
                  tunnel: w314 -> [w336]
                  tunnel: w313 -> [w337]
                  tunnel: w311 -> [w335]
                  tunnel: [w354] -> w319
                  tunnel: [w353] -> w310
                  tunnel: w317 -> [w353]
                  tunnel: w316 -> [w354]
                  frame #0 {
                    n150 = Number To Boolean Array(number=w322) -> (Boolean array=w328:bool[])
                    n151 = Index Array(array=w328, index=3) -> (element=w326:bool)
                    n152 = Index Array(array=w328, index=2) -> (element=w325:bool)
                    n153 = Index Array(array=w328, index=1) -> (element=w324:bool)
                    n154 = Index Array(array=w328, index=0) -> (element=w323:bool)
                    n155 = property on="TTL IO 4 (recording)" class="Bool (strict)"("Value"=w326) -> ()  [unwired: 2 in, 2 out]
                    n156 = property on="TTL IO 3 (recording)" class="Bool (strict)"("Value"=w325) -> ()  [unwired: 2 in, 2 out]
                    n157 = property on="TTL IO 2 (recording)" class="Bool (strict)"("Value"=w324) -> ()  [unwired: 2 in, 2 out]
                    n158 = property on="TTL IO 1 (recording)" class="Bool (strict)"("Value"=w323) -> ()  [unwired: 2 in, 2 out]
                  }
                  frame #1 {
                    n159 = call "SW_Fire_TTL_at_stop_universal.vi"("TTL port(s) config to fire"=w335, "TTL pulse length, ms"=200.0, "error in (no error)"=w339, "Serial Port In"=w336, "Close VISA (T)"=FALSE, "Start/stop signaling (F)"=w337) -> ("error out"=w342:errorcluster, "Serial Port Out"=w341:refnum<visa-resource-name>)  [unwired: 3 in, 1 out]
                  }
                  frame #2 {
                    n160 = Number To Boolean Array(number=u32 0) -> (Boolean array=w346:bool[])
                    n161 = Index Array(array=w346, index=2) -> (element=w349:bool)
                    n162 = Index Array(array=w346, index=1) -> (element=w350:bool)
                    n163 = Index Array(array=w346, index=0) -> (element=w351:bool)
                    n164 = Index Array(array=w346, index=3) -> (element=w348:bool)
                    n165 = property on="TTL IO 3 (recording)" class="Bool (strict)"("Value"=w349) -> ()  [unwired: 2 in, 2 out]
                    n166 = property on="TTL IO 2 (recording)" class="Bool (strict)"("Value"=w350) -> ()  [unwired: 2 in, 2 out]
                    n167 = property on="TTL IO 1 (recording)" class="Bool (strict)"("Value"=w351) -> ()  [unwired: 2 in, 2 out]
                    n168 = property on="TTL IO 4 (recording)" class="Bool (strict)"("Value"=w348) -> ()  [unwired: 2 in, 2 out]
                  }
                }
                n169 = property on="Stop TTL is fired" class="Bool (strict)"(error in=w310, "Value"=TRUE ("Start/Stop TTL is fired")) -> ()  [unwired: 1 in, 2 out]
              }
              frame True {
              }
            }
          }
        }
        n170 = case shown="True" w150 {
          tunnel: w156 -> [w279 w282]
          tunnel: w157 -> [w278 w283]
          tunnel: [w279 w280] -> w127
          tunnel: [w278 w281] -> w125
          frame False {
          }
          frame True {
            n171 = First Call?() -> (First Call?: T/F=w284:bool)
            n172 = case shown="True" w284 {
              tunnel: w283 -> [w285 w293]
              tunnel: w282 -> [w286 w292]
              tunnel: [w286 w288] -> w280
              tunnel: [w285 w290] -> w281
              frame False {
              }
              frame True {
                w287 = T18 16 items=["Flush Receive Buffer"=16, "Write Transmit Buffer to Device"=32, "Flush Receive Buffer (No I/O)"=64, "Flush Transmit Buffer"=128] ("Mask")
                n173 = Concatenate Strings("SYNC=0" ("string"), "\r") -> (w296:string)
                n174 = VISA Write(VISA resource name=w292, write buffer=w296, error in (no error)=w293) -> (VISA resource name out=w289:refnum<visa-resource-name>, error out=w291:errorcluster)  [unwired: 1 out]
                n175 = VISA Flush I/O Buffer(VISA resource name=w289, mask (16)=w287, error in (no error)=w291) -> (VISA resource name out=w288:refnum<visa-resource-name>, error out=w290:errorcluster)
              }
            }
          }
        }
        n176 = case shown="True" w128 {
          tunnel: w126 -> [_ w167]
          tunnel: w125 -> [_ w166]
          tunnel: w127 -> [_ w165]
          frame False {
          }
          frame True {
            n177 = call "HW_Stop_acq_and_close_VISA.vi"("error in"=w166, "Data flow controls in"=w167, "VISA resource name in"=w165) -> ()  [unwired: 2 out]
          }
        }
        n178 = node-c288(w125) -> ()  [unwired: 1 out]
      }
      n179 = node-c288(w123) -> ()  [unwired: 1 out]
    }
    frame Enabled {
    }
  }
  n180 = disable-structure shown="Disabled" {
    disable-tunnel: w3 -> [w364 _]
    disable-tunnel: w2 -> [w363 _]
    frame Disabled {
      n181 = node-c288(w364, i64 139 ("Period"), 100 ("Priority")) -> (w368:T13)  [unwired: 1 in]
      n182 = timed-loop "This loop is used only for data loading purposes (that is why it is made relatively slow)" {
        tunnel: w363 -> [w373]
        timing: w368 -> [_]
        timing-out: [_] -> w367
        stop <- w370 stop-if-true
        n183 = node-c288() -> ()  [unwired: 1 in, 1 out]
        n184 = Unbundle By Name(w373) -> ("Has been recorded"=w372:refnum<notifier>, "(Final) Data file is saved"=w379:refnum<notifier>, "Data loaded"=w378:refnum<notifier>, "Complete stop"=w371:refnum<notifier>)
        n185 = Get Notifier Status(notifier=w372) -> (current notification=w375:bool)  [unwired: 1 in, 4 out]
        n186 = Get Notifier Status(notifier=w379) -> (current notification=w377:bool)  [unwired: 1 in, 4 out]
        n187 = Get Notifier Status(notifier=w378) -> (current notification=w374:bool)  [unwired: 1 in, 4 out]
        n188 = Get Notifier Status(notifier=w371) -> (current notification=w370:bool)  [unwired: 1 in, 4 out]
        n189 = Not(x=w374) -> (.not. x?=w376:bool)
        n190 = Compound Arithmetic op=AND(w375, w377, w376) -> (w369:bool)
        n191 = case shown="True" w369 {
          tunnel: w373 -> [_ w507]
          frame False {
          }
          frame True {
            w422 = FALSE
            w428 = T12."Disabled and Grayed Out" ("Disabled")
            w451 = 7
            # "Y coord"
            # "X coord"
            # "Background color"
            # "Histogram"
            # "Diagram with zones"
            # "Diagram no zones"
            n192 = call <vilib>:"Set Busy.vi"() -> ("error out"=w382:errorcluster)  [unwired: 10 in, 1 out]
            n193 = property on="Show heatmap (analysis)" class="Bool (strict)"(error in=w382, "DisabledEnum"=w428, "Val(Sgnl)"=w422) -> (error out=w427:errorcluster)  [unwired: 1 in, 1 out]
            n194 = property on="Show full track (analysis)" class="Bool (strict)"("DisabledEnum"=w428, "Val(Sgnl)"=w422) -> (error out=w426:errorcluster)  [unwired: 2 in, 1 out]
            n195 = property on="Zones (analysis)" class="Bool (strict)"("DisabledEnum"=w428, "Val(Sgnl)"=w422) -> (error out=w425:errorcluster)  [unwired: 2 in, 1 out]
            n196 = property on="Play/Pause" class="Bool (strict)"("DisabledEnum"=w428) -> (error out=w424:errorcluster)  [unwired: 2 in, 1 out]
            n197 = Merge Errors(w427, w426, w425, w424) -> (w423:errorcluster)
            n198 = global read "SW_Globals.vi" "Cluster of paths"() -> (w387:T22)
            n199 = property on="Data loading progress" class="Slide (strict)"(error in=w423, "DisabledEnum"=T12."Disabled" ("Disabled"), "Value"=0.0 ("Data loading progress")) -> (error out=w505:errorcluster)  [unwired: 1 in, 1 out]
            n200 = Unbundle By Name(w387) -> ("Path to TDMS file"=w402:path)
            n201 = control-ref of="Data loading progress"() -> (w508:refnum<vi>)
            n202 = property on="Play/Pause" class="Bool (strict)"(error in=w505, "DisabledEnum"=T12."Disabled and Grayed Out" ("Disabled")) -> (error out=w503:errorcluster)  [unwired: 1 in, 1 out]
            n203 = call <vilib>:"Get File Extension.vi"("file"=w402) -> ("lowercase file extension"=w401:string)  [unwired: 6 in, 4 out]
            n204 = Equal?(x=w401, y="tdms") -> (x = y?=w398:bool)
            n205 = case shown="True" w398 {
              tunnel: w508 -> [w543 w551]
              tunnel: w507 -> [w545 w550]
              tunnel: w503 -> [w542 w549]
              tunnel: [w541 w548] -> w465
              tunnel: [_ w547] -> w420
              tunnel: w387 -> [w544 w546]
              tunnel: [w540 _] -> w397
              frame False {
                # "Load CSV"
                n206 = call "SW_Load_data_for_Analysis.vi"("Data flow controls"=w545, "Cluster of paths input"=w544, "Progress bar reference"=w543, "error in (no error)"=w542) -> ("Loaded data"=w540:T23, "error out"=w541:errorcluster)  [unwired: 3 in, 11 out]
              }
              frame True {
                # "Load TDMS"
                n207 = call "SW_Load_data_for_Analysis_from_TDMS.vi"("error in (no error)"=w549, "Progress bar reference"=w551, "Cluster of paths input"=w546, "Data flow controls"=w550) -> ("error out"=w548:errorcluster, "Loaded data"=w547:T24)  [unwired: 3 in, 3 out]
              }
            }
            n208 = case shown="True" w398 {
              tunnel: w420 -> [_ w539]
              tunnel: [w516 w538] -> w396
              tunnel: [w531 w537] -> w419
              tunnel: [w530 w536] -> w418
              tunnel: [w529 w535] -> w417
              tunnel: [w518 w534] -> w413
              tunnel: [w528 w533] -> w410
              tunnel: [w517 w532] -> w404
              tunnel: w397 -> [w527 _]
              frame False {
                n209 = Unbundle By Name(w527) -> ("Absolute timestamp"=w530:dbl[], "Relative timestamp"=w529:dbl[], "Zones preference array (loaded)"=w528:dbl[][], "Stimulus presets array (loaded)"=w531:T7, "Acquisition settings cluster out"=w516:T25, "X coord"=w526:dbl[], "Y coord"=w525:dbl[], "alpha rot. angle"=w524:dbl[], "alpha rot. angle"=w523:dbl[], "Current zone"=w520:dbl[], "TTL inputs"=w522:u8[], "TTL outputs"=w521:u8[])
                n210 = To Unsigned Byte Integer(number=w520) -> (unsigned 8bit integer=w519:u8[])
                n211 = Build Array(w526, w525, w524, w523) -> (w517:dbl[][])
                n212 = Build Array(w519, w522, w521) -> (w518:u8[][])
              }
              frame True {
                n213 = Unbundle By Name(w539) -> ("Absolute timestamp (DBL)"=w536:dbl[], "Relative timestamp (DBL)"=w535:dbl[], "Zones normalized allocation array"=w533:dbl[][], "Coordinates and speed"=w532:dbl[][], "Current zone and TTLs"=w534:u8[][], "Stimulus presets array"=w537:T7, "Acquisition settings cluster out"=w538:T25)
              }
            }
            "Relative timestamp (rec)" <- w417
            "Absolute timestamp (rec)" <- w418
            "Zones preference array (loaded)" <- w410
            n214 = Index Array "TTL Inputs"(array=w413, index (row)=1) -> (element=→"TTL inputs":u8[])  [unwired: 1 in]
            n215 = Index Array "TTL Outputs"(array=w413, index (row)=2) -> (element=→"TTL outputs":u8[])  [unwired: 1 in]
            n216 = Index Array "X coord"(array=w404, index (row)=0) -> (element=w408:dbl[])  [unwired: 1 in]
            "X coord" <- w408
            n217 = Index Array "Current zone"(array=w413, index (row)=0) -> (element=→"Current zone":u8[])  [unwired: 1 in]
            n218 = Index Array "Y coord"(array=w404, index (row)=1) -> (element=w406:dbl[])  [unwired: 1 in]
            "Y coord" <- w406
            n219 = Unbundle By Name(w396) -> ("Twisted neck"=w395:bool, "Offset H."=w394:sgl, "Name prefix"=w393:string, "Stop at"=w392:dbl, "\"Stop at\" enabled"=w391:bool)
            n220 = property on="Data loading progress" class="Slide (strict)"(error in=w465, "DisabledEnum"=T12."Disabled and Grayed Out" ("Disabled")) -> (error out=w432:errorcluster)  [unwired: 1 in, 1 out]
            n221 = Index Array "alpha"(array=w404, index (row)=2) -> (element=→"alpha rot. angle":dbl[])  [unwired: 1 in]
            n222 = property on="Twisted neck" class="Bool (strict)"("Value"=w395) -> ()  [unwired: 2 in, 2 out]
            n223 = property on="\"Stop at\" enabled" class="Bool (strict)"("Value"=w391) -> ()  [unwired: 2 in, 2 out]
            n224 = property on="Bridge horizontal offset" class="DigNum (strict)"("Value"=w394) -> ()  [unwired: 2 in, 2 out]
            n225 = property on="Name Prefix" class="Str"("Value"=w393) -> ()  [unwired: 2 in, 2 out]
            n226 = property on="Stop record at" class="DigNum (strict)"("Value"=w392) -> ()  [unwired: 2 in, 2 out]
            n227 = for {
              tunnel: w419 -> [w637] mode=indexing
              tunnel: [w635] -> w389 mode=indexing if=w634
              i -> [w636]
              n228 = Unbundle By Name(w637) -> ("Stim. has been set"=w634:bool)
              n229 = To Unsigned Byte Integer(number=w636) -> (unsigned 8bit integer=w635:u8)
            }
            n230 = Unbundle By Name(w396) -> ("Bridge V. offset"=w421:sgl, "Bridge swap"=→"Bridge swap (analysis)":bool, "Cage diameter, mm"=w473:u16, "N segments BORDER"=w472:u8, "Starting angle BORDER"=w471:i16, "N segments MIDFIELD"=w470:u8, "Starting angle MIDFIELD"=w469:i16, "Radius, mm MIDFIELD"=w468:u16, "Radius, mm CENTER"=w467:u16, "Researcher name"=w493:string)
            "Bridge Vertical offset (analysis)" <- w421
            n231 = Array Max & Min(array=w417) -> (max value=w500:dbl, max index (indices)=→"Index of the last recorded timepoint":i32, min value=w499:dbl)  [unwired: 1 out]
            n232 = property on="Bridge offset" class="DigNum (strict)"("Value"=w421) -> ()  [unwired: 2 in, 2 out]
            n233 = Concatenate Strings("Recorded by " ("string"), w493) -> (→"Recorded by":string)
            n234 = Compound Arithmetic op=unknown(w472, w470, u32 1 ("value")) -> (w481:u32)
            n235 = Round To Nearest(number=w499) -> (nearest integer value=w497:dbl)
            n236 = Bundle By Name(cluster=T20 {"Amount of border segments"=8, "Border segments starting angle"=0, "Amount of midfield segments"=4, "Midfield segments starting angle"=0, "Midfield segments outer radius, mm"=60, "Amount of central segments"=1, "Center segment outer radius, mm"=30, "Diameter of the cage, mm"=180, "R-gap between segments, mm"=10} ("Input cluster of parameters"), "Diameter of the cage, mm"=w473, "Amount of border segments"=w472, "Border segments starting angle"=w471, "Amount of midfield segments"=w470, "Midfield segments starting angle"=w469, "Midfield segments outer radius, mm"=w468, "Center segment outer radius, mm"=w467) -> (w390:T20)
            n237 = global write "SW_Globals.vi" "Active segments amount"(w481) -> ()
            n238 = property on="Timeline" class="Slide (strict)"(error in=w432, "Scale.Maximum"=w500, "Scale.Minimum"=w497, "Value"=w497, "DisabledEnum"=T12."Disabled and Grayed Out" ("Disabled")) -> (error out=w494:errorcluster)  [unwired: 1 in, 1 out]
            n239 = Unbundle By Name(w387) -> ("Layout picture output path"=w386:path)
            n240 = Increment(x=w481) -> (x+1=w480:u32)
            n241 = property on="Diagram at analysis" class="Pict"(error in=w494) -> (error out=w388:errorcluster, "Bounds"=w475:T19)  [unwired: 1 in, 1 out]
            n242 = flat-sequence "Full track preparation (array of clusters)" {
              tunnel: [w594] -> w439
              tunnel: w429 -> [w604]
              tunnel: w430 -> [w603]
              tunnel: w406 -> [w602]
              tunnel: w408 -> [w600]
              tunnel: [w598] -> w445
              tunnel: [w601] -> w444
              tunnel: w439 -> [w601]
              tunnel: [w633] -> w446
              tunnel: w445 -> [w633]
              tunnel: w444 -> [w632]
              tunnel: [w632] -> w442
              tunnel: [w631] -> w443
              frame #0 {
                n243 = Tick Count (ms)() -> (millisecond timer value=w594:u32)
              }
              frame #1 {
                n244 = Array Size(array=w600) -> (size(s)=w599:i32)
                n245 = for {
                  N: w599 -> [w606]
                  tunnel: w600 -> [w622]
                  tunnel: w602 -> [w621]
                  tunnel: [w616] -> w596 mode=indexing
                  tunnel: w603 -> [w619]
                  tunnel: w604 -> [w615]
                  i -> [w607]
                  n246 = Increment(x=w607) -> (x+1=w608:i32)
                  n247 = Equal?(x=w607, y=w608) -> (x = y?=w609:bool)
                  n248 = Quotient & Remainder(x=w607, y=1200) -> (x-y*floor(x/y)=w611:i32)  [unwired: 1 out]
                  n249 = Equal To 0?(x=w611) -> (x = 0?=w610:bool)
                  n250 = Or(x=w609, y=w610) -> (x .or. y?=w605:bool)
                  n251 = Index Array(array=w622, index=w607) -> (element=w613:dbl)
                  n252 = Index Array(array=w621, index=w607) -> (element=w614:dbl)
                  n253 = case shown="True" w605 {
                    tunnel: w607 -> [_ w627]
                    tunnel: w606 -> [_ w626]
                    frame False {
                    }
                    frame True {
                      n254 = Increment(x=w627) -> (x+1=w628:i32)
                      n255 = Divide(x=w628, y=w626) -> (x/y=w630:dbl)
                      n256 = Multiply(x=w630, y=20.0) -> (x*y=w625:dbl)
                      n257 = Add(x=40.0, y=w625) -> (x+y=w623:dbl)
                      n258 = local write "Data loading progress"(w623) -> ()
                    }
                  }
                  n259 = Multiply(x=w619, y=w613) -> (x*y=w618:dbl)
                  n260 = Multiply(x=w619, y=w614) -> (x*y=w617:dbl)
                  n261 = Bundle(w618, w617) -> (w620:cluster{dbl, dbl})  [unwired: 1 in]
                  n262 = Add(x=w620, y=w615) -> (x+y=w616:cluster{dbl, dbl})
                }
                n263 = Delete From Array(array=w596, length=1, index=0) -> (array with subset deleted=w598:cluster{dbl, dbl}[])  [unwired: 1 out]
              }
              frame #2 {
                n264 = Tick Count (ms)() -> (millisecond timer value=w631:u32)
              }
            }
            n265 = call <vilib>:"Check if File or Folder Exists.vi"("path"=w386) -> ("file or folder exists?"=w385:bool)  [unwired: 8 in, 2 out]
            n266 = global write "SW_Globals.vi" "Regions to track"(w389) -> ()
            n267 = Bundle By Name(cluster=T21 {"Minimum"=0.0, "Maximum"=14.0, "Increment"=1.0, "Minor Increment"=1.0, "Start"=0.0} ("X Scale.Range"), "Maximum"=w480) -> (w479:T21)
            n268 = property on="Diagram at analysis" class="Pict"() -> ("Bounds"=w460:T19)  [unwired: 2 in, 2 out]
            n269 = case shown="False" w385 {
              tunnel: w390 -> [w515 _]
              tunnel: w389 -> [w513 _]
              tunnel: w388 -> [w512 _]
              tunnel: w386 -> [w509 _]
              frame False {
                n270 = call "SW_Generate_Segmented_Plot_v3.vi"("Draw Area Size"=cluster{"Width":dbl, "Height":dbl} {"Width"=1200.0, "Height"=1200.0}, "Regions to mark set"=w513, "Input cluster of parameters"=w515, "Error In"=w512) -> ("Zones layout output"=w511:picture)  [unwired: 6 in, 5 out]
                n271 = call <vilib>:"Picture to Pixmap.vi"("picture"=w511) -> ("image data"=w510:T26)  [unwired: 9 in, 1 out]
                n272 = call <vilib>:"Write PNG File.vi"("image data"=w510, "path to PNG file"=w509) -> ()  [unwired: 8 in, 2 out]
              }
              frame True {
              }
            }
            n273 = control-ref of="Zones allocation array"() -> (w487:refnum<vi>)
            n274 = property on="Zones allocation (normalized) in analysis" class="WFGraph (strict)"("XScale.Range"=w479) -> ()  [unwired: 2 in, 2 out]
            n275 = call "SW_Generate_Segmented_Plot_v3.vi"("Draw Area Size"=w475, "Regions to mark set"=w389, "Input cluster of parameters"=w390, "Error In"=w388) -> ("Zones layout output"=w450:picture, "No zones image"=w448:picture, "Array of the pixel to color correspondences"=w477:u32[][], "Array of the segment to color correspondences"=w478:u32[][], "Cluster of image geometrical and scaling parameters"=w476:T27, "Error Out"=w466:errorcluster)  [unwired: 6 in]
            n276 = control-ref of="Diagram at analysis"() -> (w431:refnum<vi>)
            n277 = global write "SW_Globals.vi" "Diagram"(w450) -> ()
            n278 = global write "SW_Globals.vi" "Diagram no zones"(w448) -> ()
            n279 = Unbundle By Name(w476) -> ("Pixels per mm"=w430:dbl)
            n280 = global write "SW_Globals.vi" "Array of the pixel to color correspondences"(w477) -> ()
            n281 = global write "SW_Globals.vi" "Array of the segment to color correspondences"(w478) -> ()
            n282 = property class="Arr (strict)"(reference=w487, error in=w466) -> (reference out=w485:refnum<vi>, error out=w484:errorcluster, "Value"=w488:i32[])
            n283 = Quotient & Remainder(x=w460, y=T19 {"Width"=2, "Height"=2}) -> (floor(x/y)=w429:T19)  [unwired: 1 out]
            n284 = call <vilib>:"Picture to Pixmap.vi"("picture"=w448) -> ("image data"=w449:T26)  [unwired: 9 in, 1 out]
            n285 = call <vilib>:"Picture to Pixmap.vi"("picture"=w450) -> ("image data"=w464:T26)  [unwired: 9 in, 1 out]
            n286 = local write "Pixels per mm"(w430) -> ()
            n287 = call <vilib>:"Unflatten Pixmap.vi"("image data"=w449) -> ("24-bit pixmap"=w447:u32[][])  [unwired: 4 in, 6 out]
            n288 = call <vilib>:"Unflatten Pixmap.vi"("image data"=w464) -> ("24-bit pixmap"=w463:u32[][])  [unwired: 4 in, 6 out]
            n289 = Array Size(array=w488) -> (size(s)=w490:i32)
            n290 = call "SW_Gen_2D_Histogram.vi"("Picture reference in"=w431, "Pixels per mm"=w430, "Y coord array"=w406, "X coord array"=w408, "Bounds"=w429) -> ("8-bit density map"=w383:u8[][], "24-bit pixmap"=w384:u32[][])  [unwired: 4 in, 1 out]
            n291 = Array Size(array=w384) -> (size(s)=w459:i32[])
            n292 = Initialize Array(0 ("element"), w490) -> (w486:i32[])
            n293 = property class="Arr (strict)"(reference=w485, error in=w484, "Value"=w486) -> ()  [unwired: 2 out]
            n294 = Index Array(array=w459, index=0) -> (element=w455:i32)
            n295 = Index Array(array=w459, index=1) -> (element=w453:i32)
            n296 = Subtract(x=w455, y=w451) -> (x-y=w454:i32)
            n297 = Subtract(x=w453, y=w451) -> (x-y=w452:i32)
            n298 = Index Array(array=w384, index (row)=w454, index (col)=w452) -> (element=w456:u32)
            n299 = Subtract(x=w443, y=w442) -> (x-y=→"Full track preparation":u32)
            n300 = flat-sequence {
              tunnel: w446 -> [w553]
              tunnel: w448 -> [w554]
              tunnel: w450 -> [w555]
              tunnel: [w555] -> w438
              tunnel: [w554] -> w437
              tunnel: [w553] -> w436
              tunnel: [w552] -> w434
              tunnel: w462 -> [w584]
              tunnel: w440 -> [w569]
              tunnel: w438 -> [w579]
              tunnel: w437 -> [w578]
              tunnel: w436 -> [w566]
              tunnel: w383 -> [w558]
              tunnel: [w593] -> w435
              frame #0 {
                n301 = Tick Count (ms)() -> (millisecond timer value=w552:u32)
              }
              frame #1 {
                w567 = T28 {"Width"=2, "Style"=enum."Solid"} ("pen")
                n302 = global read "SW_Globals.vi" "Cluster of paths"() -> (w563:T22)
                n303 = call <vilib>:"Flatten Pixmap.vi"("24-bit pixmap"=w569) -> ("image data"=w557:T26)  [unwired: 10 in]
                n304 = call <vilib>:"Flatten Pixmap.vi"("24-bit pixmap"=w584) -> ("image data"=w556:T26)  [unwired: 10 in]
                n305 = call <vilib>:"Draw Flattened Pixmap.vi"("image data"=w557) -> ("new picture"=w564:picture)  [unwired: 8 in]
                n306 = call <vilib>:"Draw Flattened Pixmap.vi"("image data"=w556) -> ("new picture"=w571:picture)  [unwired: 8 in]
                n307 = Unbundle By Name(w563) -> ("Density map array output path"=w559:path, "Density map picture output path"=w561:path)
                n308 = call <vilib>:"Check if File or Folder Exists.vi"("path"=w561) -> ("file or folder exists?"=w562:bool)  [unwired: 8 in, 2 out]
                n309 = call <vilib>:"Check if File or Folder Exists.vi"("path"=w559) -> ("file or folder exists?"=w560:bool)  [unwired: 8 in, 2 out]
                n310 = call "SW_Make_Track_overlay.vi"("Pen properties"=w567, "Full track array"=w566, "Full trace color"="Full trace color", "Picture in"=w579) -> ("Picture out"=w581:picture)  [unwired: 3 in]
                n311 = call "SW_Make_Track_overlay.vi"("Pen properties"=w567, "Full track array"=w566, "Full trace color"="Full trace color", "Picture in"=w564) -> ("Picture out"=w565:picture)  [unwired: 3 in]
                n312 = call "SW_Make_Track_overlay.vi"("Pen properties"=w567, "Full track array"=w566, "Full trace color"="Full trace color", "Picture in"=w571) -> ("Picture out"=w570:picture)  [unwired: 3 in]
                n313 = call "SW_Make_Track_overlay.vi"("Pen properties"=w567, "Full track array"=w566, "Full trace color"="Full trace color", "Picture in"=w578) -> ("Picture out"=w582:picture)  [unwired: 3 in]
                n314 = global write "SW_Globals.vi" "Density map with zones"(w571) -> ()
                n315 = global write "SW_Globals.vi" "Density map no zones"(w564) -> ()
                n316 = call <vilib>:"Picture to Pixmap.vi"("picture"=w581) -> ("image data"=w580:T26)  [unwired: 9 in, 1 out]
                n317 = call <vilib>:"Picture to Pixmap.vi"("picture"=w565) -> ("image data"=w575:T26)  [unwired: 9 in, 1 out]
                n318 = call <vilib>:"Picture to Pixmap.vi"("picture"=w570) -> ("image data"=w574:T26)  [unwired: 9 in, 1 out]
                n319 = call <vilib>:"Picture to Pixmap.vi"("picture"=w582) -> ("image data"=w583:T26)  [unwired: 9 in, 1 out]
                n320 = call <vilib>:"Draw Flattened Pixmap.vi"("image data"=w580) -> ("new picture"=w577:picture)  [unwired: 8 in]
                n321 = call <vilib>:"Draw Flattened Pixmap.vi"("image data"=w575) -> ("new picture"=w573:picture)  [unwired: 8 in]
                n322 = call <vilib>:"Draw Flattened Pixmap.vi"("image data"=w574) -> ("new picture"=w572:picture)  [unwired: 8 in]
                n323 = call <vilib>:"Draw Flattened Pixmap.vi"("image data"=w583) -> ("new picture"=w576:picture)  [unwired: 8 in]
                n324 = global write "SW_Globals.vi" "Full track with zones"(w577) -> ()
                n325 = global write "SW_Globals.vi" "Density map with no zones and with full track"(w573) -> ()
                n326 = global write "SW_Globals.vi" "Density map with zones and full track"(w572) -> ()
                n327 = global write "SW_Globals.vi" "Full track with no zones"(w576) -> ()
                n328 = case shown="False" w562 {
                  tunnel: w561 -> [w588 _]
                  tunnel: w556 -> [w587 _]
                  frame False {
                    n329 = call <vilib>:"Write PNG File.vi"("image data"=w587, "path to PNG file"=w588) -> ()  [unwired: 8 in, 2 out]
                  }
                  frame True {
                  }
                }
                n330 = case shown="False" w560 {
                  tunnel: w559 -> [w586 _]
                  tunnel: w558 -> [w585 _]
                  frame False {
                    n331 = call-poly <vilib>:"Write Delimited Spreadsheet.vi"("file path (dialog if empty)"=w586, "2D data"=w585) -> ()  [unwired: 12 in, 2 out]
                  }
                  frame True {
                  }
                }
              }
              frame #2 {
                w592 = T12."Enabled" ("Disabled")
                n332 = local write "Data loading progress"(100.0 ("Data loading progress")) -> ()
                n333 = property on="Zones (analysis)" class="Bool (strict)"("DisabledEnum"=w592) -> ()  [unwired: 2 in, 2 out]
                n334 = property on="Play/Pause" class="Bool (strict)"("DisabledEnum"=w592) -> ()  [unwired: 2 in, 2 out]
                n335 = property on="Show heatmap (analysis)" class="Bool (strict)"("DisabledEnum"=w592) -> ()  [unwired: 2 in, 2 out]
                n336 = property on="Show full track (analysis)" class="Bool (strict)"("DisabledEnum"=w592, "Val(Sgnl)"=TRUE ("Value (Signaling)")) -> (error out=w589:errorcluster)  [unwired: 2 in, 1 out]
                n337 = Tick Count (ms)() -> (millisecond timer value=w593:u32)
                n338 = call <vilib>:"Unset Busy.vi"("error in (no error)"=w589) -> ()  [unwired: 10 in, 1 out]
              }
            }
            n339 = call "SW_Create_density_overlay.vi"("Background color"=w456, "Density histogram"=w384, "Diagram with zones"=w463, "Diagram no zones"=w447) -> ("Density map with zones"=w462:u32[][], "Density map no zones"=w440:u32[][])
            n340 = Subtract(x=w435, y=w434) -> (x-y=→"Full track plotting":u32)
          }
        }
        n341 = node-c288() -> ()  [unwired: 1 in, 1 out]
      }
      n342 = node-c288(w367) -> ()  [unwired: 1 out]
    }
    frame Enabled {
    }
  }
  n343 = disable-structure shown="Disabled" {
    disable-tunnel: _ -> [w645 _]
    disable-tunnel: _ -> [w644 _]
    frame Disabled {
      n344 = node-c288(w644, i64 499 ("Period"), 800 ("Priority")) -> (w650:T13)
      n345 = timed-loop "Loop where temporary files are transferred to permanent location and data saved" {
        tunnel: w645 -> [w677]
        tunnel: [w662] -> w648
        timing: w650 -> [_]
        timing-out: [_] -> w649
        stop <- w663 stop-if-true
        n346 = node-c288() -> (→"Save iteration duration":i64)  [unwired: 1 in]
        n347 = flat-sequence {
          tunnel: w677 -> [w938]
          tunnel: [w938] -> w676
          tunnel: w676 -> [w939]
          tunnel: [w941] -> w674
          tunnel: [w940] -> w673
          tunnel: [w939] -> w675
          frame #0 {
            n348 = Wait (ms)(milliseconds to wait=u32 521) -> ()  [unwired: 1 out]
          }
          frame #1 {
            n349 = Unbundle By Name(w939) -> ("Path to the latest complete temp file"=w941, "Temp file ready for processing"=w940)
          }
        }
        n350 = Get Notifier Status(notifier=w673) -> (error out=w672:errorcluster)  [unwired: 1 in, 4 out]
        n351 = Get Notifier Status(notifier=w674, error in (no error)=w672) -> (current notification=w668:path)  [unwired: 4 out]
        n352 = feedback-in #1(w668) -> ()
        n353 = feedback #1(path "") -> (w670:path)
        n354 = local read "Starting angle MIDFIELD"() -> (w658:i16)
        n355 = local read "Starting angle BORDER"() -> (w660:i16)
        n356 = local read "N segments MIDFIELD"() -> (w659:u8)
        n357 = local read "Radius, mm MIDFIELD"() -> (w657:u16)
        n358 = local read "N segments BORDER"() -> (w661:u8)
        n359 = local read "Radius, mm CENTER"() -> (w655:u16)
        n360 = Not Equal?(x=w670, y=w668) -> (x != y?=w669:bool)
        n361 = Not Equal?(x=path "", y=w668) -> (x != y?=w667:bool)
        n362 = Bundle By Name(cluster=T29 {"N segments BORDER"=0, "Starting angle BORDER"=0, "N segments MIDFIELD"=0, "Starting angle MIDFIELD"=0, "Radius, mm MIDFIELD"=0, "Amount of central segments"=0, "Radius, mm CENTER"=0} ("output cluster 2"), "N segments BORDER"=w661, "Starting angle BORDER"=w660, "N segments MIDFIELD"=w659, "Starting angle MIDFIELD"=w658, "Radius, mm MIDFIELD"=w657, "Amount of central segments"=u8 1, "Radius, mm CENTER"=w655) -> (w654:T29)
        n363 = And(x=w667, y=w669) -> (x .and. y?=w664:bool)
        n364 = local read "Cage diameter, mm"() -> (w653:u16)
        n365 = global read "SW_Globals.vi" "Cluster of paths"() -> (w678:T22)
        n366 = case shown="True" w664 {
          tunnel: w678 -> [_ w702]
          tunnel: w675 -> [_ w701]
          tunnel: errorcluster {"status"=FALSE, "code"=0, "source"=""} ("error constant") -> [w683 w700]
          tunnel: w664 -> [_ w699]
          tunnel: w668 -> [_ w698]
          tunnel: [FALSE w689] -> w663
          tunnel: [w683 w690] -> w662
          tunnel: w654 -> [_ w693]
          tunnel: w653 -> [_ w692]
          frame False {
          }
          frame True {
            n367 = flat-sequence {
              tunnel: w698 -> [w772]
              tunnel: w699 -> [w771]
              tunnel: w702 -> [w757]
              tunnel: w700 -> [w770]
              tunnel: [w769] -> w706
              tunnel: w701 -> [w768]
              tunnel: [w768] -> w705
              tunnel: [w757] -> w696
              tunnel: w693 -> [w756]
              tunnel: w692 -> [w755]
              tunnel: w706 -> [w912]
              tunnel: [w912] -> w704
              tunnel: [w911] -> w703
              tunnel: w705 -> [w911]
              tunnel: w696 -> [w910]
              tunnel: [w910] -> w695
              tunnel: w704 -> [w920]
              tunnel: w703 -> [w919]
              tunnel: w695 -> [w916]
              tunnel: [w921] -> w687
              tunnel: [w924] -> w686
              tunnel: [w919] -> w685
              tunnel: [w916] -> w684
              tunnel: [w934] -> w694
              tunnel: [w935] -> w688
              tunnel: [w932] -> w691
              tunnel: [w936] -> w697
              tunnel: w687 -> [w936]
              tunnel: w686 -> [w932]
              tunnel: w685 -> [w935]
              tunnel: w684 -> [w934]
              frame #0 {
                n368 = Unbundle By Name(w757) -> ("Density map array output path"=w762:path, "Layout picture output path"=w765:path, "Recording settings output path"=w764:path, "Density map picture output path"=w763:path, "Path to the settings file"=w754:path)
                n369 = case shown="True" "Save files First Call" {
                  selector: "Save files First Call" -> [w773 w786]
                  tunnel: [w776 w889] -> w761
                  tunnel: w772 -> [w776 w889]
                  tunnel: w762 -> [w774 w876]
                  tunnel: w765 -> [_ w874]
                  tunnel: w764 -> [_ w872]
                  tunnel: w763 -> [_ w844]
                  tunnel: w770 -> [w775 w841]
                  tunnel: [w775 w840] -> w760
                  tunnel: [w774 w781] -> w758
                  tunnel: w756 -> [_ w803]
                  tunnel: w755 -> [_ w801]
                  tunnel: w754 -> [_ w821]
                  tunnel: [w773 w786] -> w753
                  frame False {
                  }
                  frame True {
                    w820 = "Vertical offset" ("key")
                    w813 = "Mouse snout orientation swap?" ("key")
                    w787 = "Recording settings" ("key")
                    n370 = Unbundle By Name(w803) -> ("N segments BORDER"=w802:u8, "Starting angle BORDER"=w800:i16, "N segments MIDFIELD"=w799:u8, "Starting angle MIDFIELD"=w798:i16, "Radius, mm MIDFIELD"=w797:u16, "Radius, mm CENTER"=w795:u16)
                    n371 = property on="Save files First Call" class="Bool (strict)"("Value"=FALSE ("Save files First Call")) -> ()  [unwired: 2 in, 2 out]
                    n372 = Bundle By Name(cluster=T20 {"Amount of border segments"=8, "Border segments starting angle"=0, "Amount of midfield segments"=4, "Midfield segments starting angle"=0, "Midfield segments outer radius, mm"=60, "Amount of central segments"=1, "Center segment outer radius, mm"=30, "Diameter of the cage, mm"=180, "R-gap between segments, mm"=10} ("Input cluster of parameters"), "Diameter of the cage, mm"=w801, "Amount of border segments"=w802, "Border segments starting angle"=w800, "Amount of midfield segments"=w799, "Midfield segments starting angle"=w798, "Midfield segments outer radius, mm"=w797, "Center segment outer radius, mm"=w795) -> (w796:T20)
                    n373 = global read "SW_Globals.vi" "Regions to track"() -> (w806:u8[])
                    n374 = Build Array("X1_raw", "Y1_raw", "X2_raw", "Y2_raw", "Absolute_timestamp", "Relative_timestamp", "R", "phi", "alpha", "X", "Y", "w", "Current_zone", "Zones_preference", "TTL_inputs", "TTL_outputs", "Speed_mm_per_s", "Frame_OK") -> (w777:string[])
                    n375 = call-poly <vilib>:"Write Delimited Spreadsheet.vi"("file path (dialog if empty)"=w876, "1D data"=w777, "append to file? (new file:F)"=FALSE, "error in (no error)"=w841) -> ("new file path (Not A Path if cancelled)"=w782:path, "error out"=w779:errorcluster)  [unwired: 10 in]
                    n376 = Set Permissions(7:i16 384 ("permissions"), 8:w779, 11:w782) -> (0:w778:errorcluster, 3:w781:path)  [unwired: 2 in]
                    n377 = call "SW_Generate_Segmented_Plot_v3.vi"("Draw Area Size"=cluster{"Width":dbl, "Height":dbl} {"Width"=1200.0, "Height"=1200.0}, "Regions to mark set"=w806, "Input cluster of parameters"=w796, "Error In"=w778) -> ("Zones layout output"=w807:picture, "Error Out"=w808:errorcluster)  [unwired: 6 in, 4 out]
                    n378 = call <vilib>:"Picture to Pixmap.vi"("picture"=w807) -> ("image data"=w873:T26)  [unwired: 9 in, 1 out]
                    n379 = local read "Current User"() -> (w847:string)
                    n380 = call <vilib>:"Write PNG File.vi"("error in (no error)"=w808, "image data"=w873, "path to PNG file"=w874) -> ("error out"=w854:errorcluster)  [unwired: 7 in, 1 out]
                    n381 = call <vilib>:"Open Config Data.vi"("error in (no error)"=w854, "configuration file path"=w872) -> ("refnum"=w852:T5)  [unwired: 7 in, 2 out]
                    n382 = Strip Path(path=w844) -> (name=w843:string)  [unwired: 1 out]
                    n383 = call <vilib>:"Write Key (String).vi"("section"=w787, "value"=w847, "key"="Researcher", "refnum"=w852) -> ("error out"=w849:errorcluster, "refnum out"=w851:T5)  [unwired: 5 in, 1 out]
                    n384 = Unbundle By Name(w803) -> ("N segments MIDFIELD"=w839:u8, "N segments BORDER"=w838:u8, "Radius, mm CENTER"=w837:u16, "Radius, mm MIDFIELD"=w836:u16, "Starting angle MIDFIELD"=w835:i16, "Starting angle BORDER"=w834:i16)
                    n385 = call <vilib>:"Write Key (String).vi"("section"=w787, "error in (no error)"=w849, "value"=w843, "key"="Track name", "refnum"=w851) -> ("error out"=w848:errorcluster, "refnum out"=w850:T5)  [unwired: 4 in, 1 out]
                    n386 = call <vilib>:"Write Key (I32).vi"("section"=w787, "error in (no error)"=w848, "value"=w839, "key"="Amount of midfield segments", "refnum"=w850) -> ("error out"=w870:errorcluster, "refnum out"=w869:T5)  [unwired: 4 in, 1 out]
                    n387 = call <vilib>:"Write Key (I32).vi"("section"=w787, "error in (no error)"=w870, "value"=w838, "key"="Amount of border segments", "refnum"=w869) -> ("error out"=w866:errorcluster, "refnum out"=w867:T5)  [unwired: 4 in, 1 out]
                    n388 = call <vilib>:"Write Key (I32).vi"("section"=w787, "error in (no error)"=w866, "value"=w837, "key"="Center segment outer radius, mm", "refnum"=w867) -> ("error out"=w863:errorcluster, "refnum out"=w864:T5)  [unwired: 4 in, 1 out]
                    n389 = call <vilib>:"Write Key (I32).vi"("section"=w787, "error in (no error)"=w863, "value"=w836, "key"="Midfield segments outer radius, mm", "refnum"=w864) -> ("error out"=w860:errorcluster, "refnum out"=w861:T5)  [unwired: 4 in, 1 out]
                    n390 = call <vilib>:"Write Key (I32).vi"("section"=w787, "error in (no error)"=w860, "value"=w835, "key"="Midfield segments starting angle", "refnum"=w861) -> ("error out"=w858:errorcluster, "refnum out"=w857:T5)  [unwired: 4 in, 1 out]
                    n391 = call <vilib>:"Write Key (I32).vi"("section"=w787, "error in (no error)"=w858, "value"=w834, "key"="Border segments starting angle", "refnum"=w857) -> ("error out"=w856:errorcluster, "refnum out"=w855:T5)  [unwired: 4 in, 1 out]
                    n392 = local read "Current User"() -> (w812:string)
                    n393 = property on="Bridge offset" class="DigNum (strict)"() -> ("Value"=w819:sgl)  [unwired: 2 in, 2 out]
                    n394 = call <vilib>:"Write Key (I32).vi"("section"=w787, "error in (no error)"=w856, "value"=w801, "key"="Cage diameter, mm", "refnum"=w855) -> ("error out"=w826:errorcluster, "refnum out"=w823:T5)  [unwired: 4 in, 1 out]
                    n395 = call <vilib>:"Open Config Data.vi"("configuration file path"=w821) -> ("error out"=w818:errorcluster, "refnum"=w816:T5)  [unwired: 8 in, 1 out]
                    n396 = property on="Bridge swap" class="Bool (strict)"() -> ("Value"=w814:bool)  [unwired: 2 in, 2 out]
                    n397 = call <vilib>:"Write Key (Double).vi"("use system decimal point (T)"=FALSE, "section"=w812, "error in (no error)"=w818, "value"=w819, "key"=w820, "refnum"=w816) -> ("error out"=w815:errorcluster, "refnum out"=w811:T5)  [unwired: 3 in, 1 out]
                    n398 = call <vilib>:"Write Key (Double).vi"("use system decimal point (T)"=FALSE, "section"=w787, "error in (no error)"=w826, "value"=w819, "key"=w820, "refnum"=w823) -> ("error out"=w825:errorcluster, "refnum out"=w824:T5)  [unwired: 3 in, 1 out]
                    n399 = call <vilib>:"Write Key (Boolean).vi"("section"=w812, "error in (no error)"=w815, "value"=w814, "key"=w813, "refnum"=w811) -> ("error out"=w810:errorcluster, "refnum out"=w809:T5)  [unwired: 4 in, 1 out]
                    n400 = call <vilib>:"Write Key (Boolean).vi"("section"=w787, "error in (no error)"=w825, "value"=w814, "key"=w813, "refnum"=w824) -> ("error out"=w830:errorcluster, "refnum out"=w831:T5)  [unwired: 4 in, 1 out]
                    n401 = call <vilib>:"Close Config Data.vi"("error in (no error)"=w810, "refnum"=w809) -> ()  [unwired: 8 in, 2 out]
                    n402 = property on="Stimulus presets" class="Arr (strict)"(error in=w830) -> (error out=w790:errorcluster, "Value"=w832:T7)  [unwired: 1 in, 1 out]
                    n403 = for {
                      tunnel: w832 -> [w902] mode=indexing
                      tunnel: w831 -> [w895]
                      tunnel: [w899] -> w791
                      tunnel: w787 -> [w890]
                      i -> [w898]
                      n404 = Unbundle By Name(w902) -> ("Stim. has been set"=w900:bool)
                      n405 = Flatten To JSON(anything=w902) -> (JSON string=w901:string, 11:w892:errorcluster)  [unwired: 2 in]
                      n406 = Format Value(string ("")="Zone " ("string"), format string="%02d", value (0)=w898) -> (output string=w893:string)
                      n407 = call <vilib>:"Remove Key.vi"("section"=w890, "error in (no error)"=w892, "key"=w893, "refnum"=w895) -> ("error out"=w891:errorcluster, "refnum out"=w894:T5)  [unwired: 5 in, 1 out]
                      n408 = case shown="False" w900 {
                        tunnel: w901 -> [_ w909]
                        tunnel: w891 -> [_ w908]
                        tunnel: [w903 w907] -> w899
                        tunnel: w893 -> [_ w906]
                        tunnel: w894 -> [w903 w905]
                        tunnel: w890 -> [_ w904]
                        frame False {
                        }
                        frame True {
                          n409 = call <vilib>:"Write Key (String).vi"("section"=w904, "error in (no error)"=w908, "value"=w909, "key"=w906, "refnum"=w905) -> ("refnum out"=w907:T5)  [unwired: 4 in, 2 out]
                        }
                      }
                    }
                    n410 = property on="IO parameters string" class="Str"(error in=w790) -> (error out=w792:errorcluster, "Value"=w793:string)  [unwired: 1 in, 1 out]
                    n411 = call <vilib>:"Write Key (String).vi"("section"=w787, "error in (no error)"=w792, "value"=w793, "key"="IO ports configuration", "refnum"=w791) -> ("error out"=w789:errorcluster, "refnum out"=w788:T5)  [unwired: 4 in, 1 out]
                    n412 = call <vilib>:"Close Config Data.vi"("error in (no error)"=w789, "refnum"=w788) -> ("error out"=w840:errorcluster)  [unwired: 8 in, 1 out]
                  }
                }
                n413 = call-poly <vilib>:"Read Delimited Spreadsheet.vi"("file path (dialog if empty)"=w761, "error in (no error)"=w760) -> ("all rows"=w752:string[][], "error out"=w759:errorcluster)  [unwired: 8 in, 4 out]
                n414 = Array Subset(array=w752, index (row)=1 ("index")) -> (w751:string[][])  [unwired: 3 in]
                n415 = Select(t=w751, s=w753, f=w752) -> (s? t:f=w748:string[][])
                n416 = call-poly <vilib>:"Write Delimited Spreadsheet.vi"("file path (dialog if empty)"=w758, "format (%s)"="%s", "2D data"=w748, "append to file? (new file:F)"=TRUE, "error in (no error)"=w759) -> ("error out"=w769:errorcluster)  [unwired: 9 in, 1 out]
                "Path to the latest saved temp file" <- w772
                "Temp file ready" <- w771
              }
              frame #1 {
                n417 = Wait (ms)(milliseconds to wait=u32 257 ("millisecond multiple")) -> ()  [unwired: 1 out]
              }
              frame #2 {
                n418 = Unbundle By Name(w919) -> ("Recording now"=w915, "Has been recorded"=w914, "Path to the latest complete temp file"=w930, "Temp file ready for processing"=w931)
                n419 = Send Notification(notification=FALSE, notifier=w931, error in (no error)=w920) -> (error out=w929:errorcluster)  [unwired: 1 out]
                n420 = Get Notifier Status(notifier=w930, error in (no error)=w929) -> (current notification=w917:path, error out=w928:errorcluster)  [unwired: 3 out]
                n421 = Delete(path (use dialog)=w917, error in=w928) -> (error out=w923:errorcluster)  [unwired: 3 in, 2 out]
                n422 = Get Notifier Status(notifier=w914, error in (no error)=w923) -> (current notification=w925:bool, error out=w922:errorcluster)  [unwired: 3 out]
                n423 = Get Notifier Status(notifier=w915, error in (no error)=w922) -> (current notification=w927:bool, error out=w921:errorcluster)  [unwired: 3 out]
                n424 = Not(x=w927) -> (.not. x?=w926:bool)
                n425 = And(x=w926, y=w925) -> (x .and. y?=w924:bool)
              }
              frame #3 {
                n426 = Wait (ms)(milliseconds to wait=u32 257 ("millisecond multiple")) -> ()  [unwired: 1 out]
              }
            }
            n427 = case "Case Here data saving will be finalized" shown="True" w691 {
              selector: w691 -> [w708 w721]
              tunnel: w697 -> [w707 w710]
              tunnel: [w708 w721] -> w689
              tunnel: w694 -> [_ w722]
              tunnel: [w707 w718] -> w690
              tunnel: w688 -> [_ w715]
              frame False {
              }
              frame True {
                n428 = Unbundle By Name(w722) -> ("Density map picture output path"=w716:path, "Density map array output path"=w712:path)
                n429 = Set Permissions(7:i16 438 ("permissions"), 8:w710, 11:w712) -> (0:w709:errorcluster, 3:w713:path)  [unwired: 2 in]
                n430 = while {
                  tunnel: w713 -> [w731]
                  tunnel: w716 -> [w729]
                  tunnel: w709 -> [w733]
                  tunnel: [w732] -> w719
                  tunnel: w715 -> [w730]
                  tunnel: [w730] -> w714
                  i -> [w726]
                  stop <- w723 stop-if-true
                  n431 = flat-sequence {
                    tunnel: w733 -> [w737]
                    tunnel: w731 -> [w735]
                    tunnel: w729 -> [w734]
                    tunnel: [w736] -> w728
                    tunnel: [w734] -> w725
                    tunnel: w728 -> [w740]
                    tunnel: [w740] -> w727
                    tunnel: w725 -> [w738]
                    tunnel: [w738] -> w724
                    tunnel: [w747] -> w732
                    tunnel: w727 -> [w747]
                    tunnel: w726 -> [w743]
                    tunnel: w724 -> [w742]
                    tunnel: [w741] -> w723
                    frame #0 {
                      n432 = Move(source path=w735, error in=w737, 10:w734) -> (error out=w736:errorcluster)  [unwired: 2 in, 2 out]
                    }
                    frame #1 {
                      n433 = Wait (ms)(milliseconds to wait=u32 500) -> ()  [unwired: 1 out]
                    }
                    frame #2 {
                      n434 = call <vilib>:"Check if File or Folder Exists.vi"("path"=w742) -> ("file or folder exists?"=w746:bool)  [unwired: 8 in, 2 out]
                      n435 = Greater?(x=w743, y=9) -> (0:w745:bool)
                      n436 = Or(x=w745, y=w746) -> (x .or. y?=w741:bool)
                    }
                  }
                }
                n437 = Unbundle By Name(w714) -> ("(Final) Data file is saved"=w720)
                n438 = Send Notification(notification=TRUE, notifier=w720, error in (no error)=w719) -> (error out=w718:errorcluster)  [unwired: 1 out]
              }
            }
          }
        }
        n439 = node-c288() -> ()  [unwired: 1 in, 1 out]
      }
      "error out" <- w648
      n440 = node-c288(w649) -> ()  [unwired: 1 out]
    }
    frame Enabled {
    }
  }
  n441 = disable-structure shown="Disabled" {
    frame Disabled {
      n442 = while {
        stop <- w948 stop-if-true
        # "Only deals with application closing and stopping"
        n443 = event shown="[1] Panel Close?" {
          selector: _ -> [_ _]
          dyn-events: _ -> [_ _]
          timeout: 500 -> [_ _]
          tunnel: [FALSE TRUE] -> w948
          event Timeout {
            n444 = event-data() -> ()  [unwired: 1 in, 3 out]
          }
          event Panel Close? {
            w954 = T18 128 items=["Flush Receive Buffer"=16, "Write Transmit Buffer to Device"=32, "Flush Receive Buffer (No I/O)"=64, "Flush Transmit Buffer"=128] ("Mask")
            w952 = FALSE ("Serial port opened")
            n445 = event-data() -> ()  [unwired: 1 in, 4 out]
            n446 = property on="Serial OUT name" class="VISAName"() -> (error out=w955:errorcluster, "Value"=w953:refnum<visa-resource-name>)  [unwired: 2 in, 1 out]
            n447 = VISA Flush I/O Buffer(VISA resource name=w953, mask (16)=w954, error in (no error)=w955) -> (VISA resource name out=w956:refnum<visa-resource-name>, error out=w957:errorcluster)
            n448 = VISA Clear(VISA resource name=w956, error in (no error)=w957) -> (VISA resource name out=w959:refnum<visa-resource-name>, error out=w958:errorcluster)
            n449 = VISA Close(VISA resource name=w959, error in (no error)=w958) -> (error out=w961:errorcluster)
            n450 = call <vilib>:"Clear Errors.vi"("error in (no error)"=w961) -> ("error out"=w962:errorcluster)  [unwired: 5 in, 1 out]
            n451 = property on="Serial port opened" class="Bool (strict)"(error in=w962, "Value"=w952) -> (error out=w960:errorcluster)  [unwired: 1 in, 1 out]
            n452 = property on="Streaming" class="Bool (strict)"(error in=w960, "Value"=w952) -> (error out=w966:errorcluster)  [unwired: 1 in, 1 out]
            n453 = Current VI's Path() -> (path=w963:path)
            n454 = Open VI Reference(vi path=w963, error in (no error)=w966) -> (vi reference=w964:refnum<vi>, error out=w965:errorcluster)  [unwired: 4 in]
            n455 = invoke class="VI" method="FP.Close"(reference=w964, error in=w965) -> ()  [unwired: 1 in, 3 out]
            n456 = event-data() -> ()  [unwired: 2 in, 1 out]
          }
        }
      }
    }
    frame Enabled {
    }
  }
  n457 = flat-sequence "Things to run at the very beginning of the program" {
    tunnel: [w976] -> w26
    tunnel: [w1096] -> w19
    tunnel: [w1004] -> w3
    frame #0 {
      w967 = T11 [{"Numeric Control"=12369084, "Numeric Control"=12369084}, {"Numeric Control"=16757760, "Numeric Control"=16757760}, {"Numeric Control"=1976113, "Numeric Control"=8355711}, {"Numeric Control"=3355443, "Numeric Control"=6710886}]  # Button port OFF colors
      w1050 = T11 [{"Numeric Control"=9868950, "Numeric Control"=15790320}, {"Numeric Control"=8388608, "Numeric Control"=8388608}, {"Numeric Control"=4934475, "Numeric Control"=7895160}, {"Numeric Control"=994319, "Numeric Control"=1657881}]  # TTL IO In colors
      w1051 = T11 [{"Numeric Control"=9868950, "Numeric Control"=15790320}, {"Numeric Control"=1988894, "Numeric Control"=3381555}, {"Numeric Control"=4934475, "Numeric Control"=7895160}, {"Numeric Control"=994319, "Numeric Control"=1657881}]  # TTL IO Out colors
      w1074 = T12."Enabled" ("Disabled")
      w1105 = FALSE ("Recording has been started with TTL")
      w981 = "Researcher"
      w1133 = enum32{"Settings", "Recording", "Analysis"}."Settings" ("Main tab control")
      w1140 = enum32{"Settings", "Recording", "Analysis"}."Analysis" ("Main tab control")
      w1148 = enum32{"Settings", "Recording", "Analysis"}."Recording" ("Main tab control")
      n458 = property on="Open serial port" class="Bool (strict)"("Value"=FALSE ("Open serial port")) -> ()  [unwired: 2 in, 2 out]
      n459 = property on="Expand/hide stream panel (Rec)" class="Bool (strict)"("Value"=FALSE ("Expand/hide stream panel (Rec)")) -> ()  [unwired: 2 in, 2 out]
      n460 = property on="Streaming" class="Bool (strict)"("DisabledEnum"=T12."Disabled and Grayed Out" ("Disabled")) -> ()  [unwired: 2 in, 2 out]
      n461 = property on="IO paramaters loaded from file" class="Bool (strict)"("Value"=FALSE ("IO paramaters loaded from file")) -> ()  [unwired: 2 in, 2 out]
      n462 = call-poly <vilib>:"Create Timing Source.vi"("error in (no error)"="error in (no error)", "name (in)"="1 kHz") -> ("error out"=w1003:errorcluster, "name (out)"=w1004:string)  [unwired: 8 in]
      n463 = property on="Jump to Analysis" class="Bool (strict)"(error in=w1003, "Value"=FALSE ("Jump to Analysis")) -> (error out=w1044:errorcluster)  [unwired: 1 in, 1 out]
      n464 = property on="IO parameters string" class="Str"(error in=w1044, "Value"="[12,1,1,0,0,0]" ("IO parameters string")) -> (error out=w1072:errorcluster)  [unwired: 1 in, 1 out]
      n465 = property on="Pane" class="Pane"(error in=w1072) -> (error out=w1082:errorcluster, "Decos[]"=w1083:refnum<vi>[])  [unwired: 1 in, 1 out]
      n466 = for {
        tunnel: w1083 -> [w1170] mode=indexing
        tunnel: w1082 -> [w1168]
        tunnel: [w1167] -> w1076
        n467 = property class="Decor"(reference=w1170, error in=w1168, "Visible"=FALSE) -> (error out=w1167:errorcluster)  [unwired: 1 out]
      }
      n468 = property on="Bridge offset" class="DigNum (strict)"(error in=w1076, "DisabledEnum"=w1074) -> (error out=w1075:errorcluster)  [unwired: 1 in, 1 out]
      n469 = property on="Back to Settings" class="Bool (strict)"(error in=w1075, "DisabledEnum"=w1074, "Visible"=FALSE) -> (error out=w1085:errorcluster)  [unwired: 1 in, 1 out]
      n470 = call "FL_Gen_Bins_for_RunTimes.vi"("Min time, s"=0.5 ("Min run, m"), "N bins"=u16 11, "Max time, s"=10.0 ("Max run, m")) -> ("Bins array"=w1011:dbl[])  [unwired: 1 in]
      n471 = Array Size(array=w1011) -> (size(s)=w1013:i32)
      n472 = Initialize Array(u32 0 ("element"), w1013) -> (w1015:u32[])
      n473 = global write "SW_Globals.vi" "Run Times distribution array"(w1015) -> ()
      n474 = call "FL_Gen_Bins_for_RunLengths.vi"("Min run, m"=0.2, "N bins"=u16 11, "Max run, m"=2.0) -> ("Bins array"=w1019:dbl[])  [unwired: 1 in]
      n475 = Array Size(array=w1019) -> (size(s)=w1021:i32)
      n476 = Initialize Array(u32 0 ("element"), w1021) -> (w1018:u32[])
      n477 = global write "SW_Globals.vi" "Run Lengts distribution array"(w1018) -> ()
      n478 = global write "SW_Globals.vi" "Run Times bins array"(w1011) -> ()
      n479 = property on="Expand/hide stream panel (Rec)" class="Bool (strict)"("Colors [4]"=w967) -> ()  [unwired: 2 in, 2 out]
      n480 = global write "SW_Globals.vi" "Run Lengths bins array"(w1019) -> ()
      n481 = property class="App"() -> ("App.Kind"=w1119:T34)  [unwired: 2 in, 2 out]
      n482 = property on="Ready" class="Bool (strict)"(error in=w1085, "Value"=FALSE ("Ready")) -> (error out=w1043:errorcluster)  [unwired: 1 in, 1 out]
      n483 = global write "SW_Globals.vi" "Run time, s"(0.0 ("Run time, s")) -> ()
      n484 = case shown="\"invalid app kind\", Default" w1119 {
        tunnel: [w1197 w1198 w1199] -> w1112
        frame "invalid app kind", Default {
          n485 = call <vilib>:"Application Directory.vi"() -> ("Application Directory"=w1197:path)
          "Application Directory" <- w1197
        }
        frame "Run Time System" {
          n486 = call <vilib>:"Application Directory.vi"() -> ("Application Directory"=w1198:path)
        }
        frame "Development System" {
          n487 = Current VI's Path() -> (path=w1200:path)
          n488 = Strip Path(path=w1200) -> (stripped path=w1199:path)  [unwired: 1 out]
        }
      }
      n489 = property on="TTL 1 counter" class="DigNum (strict)"("Value"=0 ("TTL 1 counter")) -> ()  [unwired: 2 in, 2 out]
      n490 = property on="TTL 2 counter" class="DigNum (strict)"("Value"=0 ("TTL 1 counter")) -> ()  [unwired: 2 in, 2 out]
      n491 = property on="TTL 3 counter" class="DigNum (strict)"("Value"=0 ("TTL 1 counter")) -> ()  [unwired: 2 in, 2 out]
      n492 = property on="TTL 4 counter" class="DigNum (strict)"("Value"=0 ("TTL 1 counter")) -> ()  [unwired: 2 in, 2 out]
      n493 = global write "SW_Globals.vi" "Recording start timestamp"(timestamp(0 s since 1904-01-01) ("Recording start timestamp")) -> ()
      n494 = call "SW_Generate_Color_Ramp.vi"() -> ("Colors array"=w1125:u32[])  [unwired: 2 in]
      n495 = property on="Zone-based stimulus setup" class="RadioBtnsControl (strict)"(error in=w1043, "Value"=T31."No Selection" ("Stimulus")) -> (error out=w1104:errorcluster)  [unwired: 1 in, 1 out]
      n496 = property on="Pane" class="Pane"("Origin"=T33 {"Horizontal"=0, "Vertical"=0}) -> ()  [unwired: 2 in, 2 out]
      n497 = global write "SW_Globals.vi" "Color ramp array"(w1125) -> ()
      n498 = Build Path(base path=w1112, name or relative path=path "Tracker_settings.tcf") -> (appended path=w1107:path)
      "Path to the settings file" <- w1107
      n499 = call "FL_Gen_Bins_for_Speed.vi"("Speed min"=8.0, "N bins"=u16 10, "Speed max"=300.0) -> ("Bins array"=w1037:dbl[])  [unwired: 1 in]
      n500 = global read "SW_Globals.vi" "Cluster of paths"() -> (w1108:T22)
      n501 = call <vilib>:"Open Config Data.vi"("error in (no error)"=w1104, "create file if necessary (T)"=FALSE, "configuration file path"=w1107) -> ("error out"=w1158:errorcluster, "refnum"=w1157:T5)  [unwired: 6 in, 1 out]
      n502 = Array Size(array=w1037) -> (size(s)=w1036:i32)
      n503 = Initialize Array(u32 0 ("element"), w1036) -> (w1035:u32[])
      n504 = global write "SW_Globals.vi" "Speed bins array"(w1037) -> ()
      n505 = Bundle By Name(cluster=w1108, "Path to the settings file"=w1107) -> (w1106:T22)
      n506 = call <vilib>:"Get Key Names.vi"("section"="Users", "error in (no error)"=w1158, "refnum"=w1157) -> ("error out"=w1154:errorcluster, "key names"=w1150:string[], "refnum out"=w1155:T5)  [unwired: 5 in, 1 out]
      n507 = property on="Type of histogram" class="DigNum (strict)"("Value"=u8 0 ("Type of histogram")) -> (error out=w1017:errorcluster)  [unwired: 2 in, 1 out]
      n508 = property on="Histograms (normalized)" class="WFGraph (strict)"(error in=w1017, "XScale.Ofst&Mult"=T30 {"Offset"=1.0, "Multiplier"=0.0} ("X Scale.Offset and Multiplier"), "XScale.ScaleFit"=u8 0 ("X Scale.Scale Fit"), "YScale.Mapping Mode"=u8 0 ("Y Scale.Mapping Mode"), "Plot.Fill/Pt. Color"=u32 15790320 ("Plot.Fill/Point Color"), "XScale.Range"=T21 {"Minimum"=0.0, "Maximum"=14.0, "Increment"=1.0, "Minor Increment"=1.0, "Start"=0.0} ("X Scale.Range")) -> ()  [unwired: 1 in, 2 out]
      n509 = global write "SW_Globals.vi" "Speed distribution array"(w1035) -> ()
      n510 = call <vilib>:"Read Key (U32).vi"("section"="Defaults", "error in (no error)"=w1154, "key"="Default User", "refnum"=w1155) -> ("error out"=w980:errorcluster, "value"=w1151:u32, "refnum out"=w1129:T5)  [unwired: 4 in, 1 out]
      n511 = global write "SW_Globals.vi" "Cluster of paths"(w1106) -> ()
      n512 = Index Array(array=w1150, index=w1151) -> ()  [unwired: 1 out]
      n513 = call "SW_Load_settings_to_main_tab.vi"("Refnum in"=w1129, "User Name"=w981, "error in (no error)"=w980) -> ("VISA resource name"=w976:string, "Refnum out"=→"Settings file refnum out":T5, "IO parameters cluster"=w979:T2, "Settings cluster out"=w977:T35, "Stimulus presets array"=w978:T36, "error out"=w1064:errorcluster)  [unwired: 2 in]
      "Port" <- w976
      n514 = Unbundle By Name(w977) -> ("Name prefix"=w996:string, "Twisted neck"=w995:bool, "Offset H."=w992:sgl, "Stop at"=w994:dbl, "\"Stop at\" enabled"=w993:bool, "N segments MIDFIELD"=w990:u8, "N segments BORDER"=w989:u8, "Radius, mm CENTER"=w988:u16, "Radius, mm MIDFIELD"=w987:u16, "Starting angle MIDFIELD"=w986:i16, "Starting angle BORDER"=w985:i16, "Cage diameter, mm"=w983:u16, "Bridge swap"=w984:bool, "Bridge V. offset"=w991:sgl, "Data filtering"=w972:u16)
      n515 = case "Let's set flag for alternative magnets orintation" shown="240" w983 {
        frame 180, Default {
          n516 = global write "SW_Globals.vi" "Alternative magnets orientation"(FALSE ("Alternative magnets orientation")) -> ()
        }
        frame 240 {
          n517 = global write "SW_Globals.vi" "Alternative magnets orientation"(FALSE ("Alternative magnets orientation")) -> ()
        }
        frame 290 {
          n518 = global write "SW_Globals.vi" "Alternative magnets orientation"(FALSE ("Alternative magnets orientation")) -> ()
        }
        frame 325 {
          n519 = global write "SW_Globals.vi" "Alternative magnets orientation"(FALSE ("Alternative magnets orientation")) -> ()
        }
        frame 327 {
          n520 = global write "SW_Globals.vi" "Alternative magnets orientation"(TRUE ("Alternative magnets orientation")) -> ()
        }
        frame 333 {
          n521 = global write "SW_Globals.vi" "Alternative magnets orientation"(FALSE ("Alternative magnets orientation")) -> ()
        }
      }
      n522 = local write "Name Prefix"(w996) -> ()
      n523 = local write "Twisted neck"(w995) -> ()
      n524 = local write "Bridge horizontal offset"(w992) -> ()
      n525 = local write "Stop record at"(w994) -> ()
      n526 = local write "\"Stop at\" enabled"(w993) -> ()
      n527 = local write "N segments MIDFIELD"(w990) -> ()
      n528 = local write "N segments BORDER"(w989) -> ()
      n529 = local write "Radius, mm CENTER"(w988) -> ()
      n530 = local write "Radius, mm MIDFIELD"(w987) -> ()
      n531 = local write "Bridge offset"(w991) -> ()
      n532 = local write "Starting angle MIDFIELD"(w986) -> ()
      n533 = local write "Starting angle BORDER"(w985) -> ()
      n534 = local write "Cage diameter, mm"(w983) -> ()
      n535 = local write "Data filtering"(w972) -> ()
      n536 = Unbundle By Name(w979) -> ("SYNC configuration"=w1067:u16, "IO 1 configuration"=w1008:u16, "IO 2 configuration"=w1007:u16)
      n537 = call "SW_get_config_of_Zones_and_IO.vi"("Sync parameters cluster input"=w979) -> ("Zones out config bin"=w1060:bool[], "Ports IO config (OUT is FALSE)"=w1042:bool[], "IO inversion config."=w1002:u16)  [unwired: 1 out]
      n538 = global write "SW_Globals.vi" "IO inversion config."(w1002) -> ()
      n539 = property on="Bridge swap" class="Bool (strict)"(error in=w1064, "DisabledEnum"=T12."Enabled" ("Disabled"), "Value"=w984) -> (error out=w1110:errorcluster)  [unwired: 1 in, 1 out]
      n540 = call "SW_get_config_for_Start_Stop_pulses.vi"("Sync parameters cluster input"=w979) -> ("Start/Stop out pulses config"=→"Start/Stop out pulses config":u32, "Start/Stop in config"=→"Start/Stop in config":u32, "Start/Stop in config bin"=w1062:bool[], "Start/Stop out pulses config bin"=w1061:bool[])
      n541 = call "SW_Gen_Available_TTL_outputs_array.vi"("IO 2 configuration"=w1007, "IO 1 configuration"=w1008, "SYNC configuration"=w1067) -> ("Available TTL outputs array"=w1066:cluster{"String":string, "Value":i32}[])
      n542 = global write "SW_Globals.vi" "IO parameters cluster"(w979) -> ()
      n543 = global write "SW_Globals.vi" "Start/Stop out pulses config bin"(w1061) -> ()
      n544 = property on="TTL out" class="Ring (strict)"("StringsAndValues[]"=w1066) -> ()  [unwired: 2 in, 2 out]
      n545 = global write "SW_Globals.vi" "Zones out config bin"(w1060) -> ()
      n546 = global write "SW_Globals.vi" "Start/Stop in config bin"(w1062) -> ()
      n547 = global write "SW_Globals.vi" "IO ports config"(w1042) -> ()
      n548 = call "SW_get_IO_ports_representation.vi"("Sync parameters cluster input"=w979) -> ("IO status indicator"=→"IO status indicator":T6)
      n549 = property on="Main tab control" class="TabCtl (strict)"(error in=w1110, "Value"=w1148) -> (error out=w1145:errorcluster, "Pages"=w1149:refnum<vi>[])  [unwired: 1 in, 1 out]
      n550 = Index Array(array=w1042, index=0) -> (element=w1055:bool)
      n551 = Index Array(array=w1042, index=1) -> (element=w1054:bool)
      n552 = Index Array(array=w1042, index=2) -> (element=w1053:bool)
      n553 = Index Array(array=w1042, index=3) -> (element=w1052:bool)
      n554 = To Long Integer(number=w1148) -> (32bit integer=w1147:i32)
      n555 = Select(t=w1050, s=w1055, f=w1051) -> (s? t:f=w1049:T11)
      n556 = Select(t=w1050, s=w1054, f=w1051) -> (s? t:f=w1048:T11)
      n557 = Select(t=w1050, s=w1052, f=w1051) -> (s? t:f=w1046:T11)
      n558 = Index Array(array=w1149, index=w1147) -> (element=w1146:refnum<vi>)
      n559 = Select(t=w1050, s=w1053, f=w1051) -> (s? t:f=w1047:T11)
      n560 = property class="Page"(reference=w1146, error in=w1145, "PageEnb"=T32."Page Disabled & Grayed" ("Page Enabled State")) -> (error out=w1143:errorcluster)  [unwired: 1 out]
      n561 = property on="TTL IO 1 (recording)" class="Bool (strict)"("Colors [4]"=w1049) -> ()  [unwired: 2 in, 2 out]
      n562 = property on="TTL IO 3 (recording)" class="Bool (strict)"("Colors [4]"=w1047) -> ()  [unwired: 2 in, 2 out]
      n563 = property on="TTL IO 2 (recording)" class="Bool (strict)"("Colors [4]"=w1048) -> ()  [unwired: 2 in, 2 out]
      n564 = property on="TTL IO 1 (analysis)" class="Bool"("Colors [4]"=w1049) -> ()  [unwired: 2 in, 2 out]
      n565 = property on="TTL IO 4 (recording)" class="Bool (strict)"("Colors [4]"=w1046) -> ()  [unwired: 2 in, 2 out]
      n566 = property on="Main tab control" class="TabCtl (strict)"(error in=w1143, "Value"=w1140) -> (error out=w1142:errorcluster, "Pages"=w1141:refnum<vi>[])  [unwired: 1 in, 1 out]
      n567 = To Long Integer(number=w1140) -> (32bit integer=w1139:i32)
      n568 = property on="TTL IO 3 (analysis)" class="Bool"("Colors [4]"=w1047) -> ()  [unwired: 2 in, 2 out]
      n569 = property on="TTL IO 2 (analysis)" class="Bool"("Colors [4]"=w1048) -> ()  [unwired: 2 in, 2 out]
      n570 = Index Array(array=w1141, index=w1139) -> (element=w1138:refnum<vi>)
      n571 = property on="TTL IO 4 (analysis)" class="Bool"("Colors [4]"=w1046) -> ()  [unwired: 2 in, 2 out]
      n572 = global write "SW_Globals.vi" "TTL recording start signal has been successfully reset"(w1105) -> ()
      n573 = property class="Page"(reference=w1138, error in=w1142, "PageEnb"=T32."Page Disabled & Grayed" ("Page Enabled State")) -> (error out=w1130:errorcluster)  [unwired: 1 out]
      n574 = global write "SW_Globals.vi" "Recording has been stopped with TTL"(w1105) -> ()
      n575 = global write "SW_Globals.vi" "Recording has been started with TTL"(w1105) -> ()
      n576 = property on="Main tab control" class="TabCtl (strict)"(error in=w1130, "Value"=w1133) -> (error out=w1131:errorcluster, "Pages"=w1132:refnum<vi>[])  [unwired: 1 in, 1 out]
      n577 = To Long Integer(number=w1133) -> (32bit integer=w1134:i32)
      n578 = for {
        tunnel: w978 -> [w1175] mode=indexing
        tunnel: [w1174] -> w1086 mode=indexing if=w1173
        i -> [w1172]
        n579 = Greater Than 0?(x=w1172) -> (x > 0?=w1171:bool)
        n580 = Unbundle By Name(w1175) -> ("Stim. has been set"=w1173:bool)
        n581 = case shown="True" w1171 {
          tunnel: w1173 -> [_ w1186]
          tunnel: w1172 -> [_ w1182]
          frame False {
          }
          frame True {
            w1180 = refnum<vi> refnum  # Boolean
            n582 = property on="Colors for Stim. setup" class="Arr (strict)"() -> ("Value"=w1185:T3)  [unwired: 2 in, 2 out]
            n583 = Decrement(x=w1182) -> (x-1=w1176:i32)
            n584 = property on="Zone-based stimulus setup" class="RadioBtnsControl (strict)"() -> ("Controls[]"=w1183:refnum<vi>[])  [unwired: 2 in, 2 out]
            n585 = Select(t=w1185, s=w1186, f=T11 [{"Numeric Control"=12369084, "Numeric Control"=12369084}, {"Numeric Control"=6603023, "Numeric Control"=6603023}, {"Numeric Control"=1976113, "Numeric Control"=1976113}, {"Numeric Control"=2575993, "Numeric Control"=2575993}] ("Colors [4] 2")) -> (s? t:f=w1178:T11)
            n586 = Index Array(array=w1183, index=w1176) -> (element=w1181:refnum<vi>)
            n587 = To More Specific Class(target class=w1180, reference=w1181) -> (specific class reference=w1179:refnum<vi>)  [unwired: 1 in, 1 out]
            n588 = property class="Bool"(reference=w1179, "Colors [4]"=w1178, "Value"=FALSE) -> ()  [unwired: 1 in, 2 out]
          }
        }
        n589 = To Unsigned Byte Integer(number=w1172) -> (unsigned 8bit integer=w1174:u8)
      }
      n590 = global write "SW_Globals.vi" "Regions to track"(u8[] [] ("Regions to track")) -> ()
      n591 = Index Array(array=w1132, index=w1134) -> (element=w1135:refnum<vi>)
      n592 = property class="Page"(reference=w1135, error in=w1131, "PageEnb"=T32."Page Enabled" ("Page Enabled State")) -> (error out=w1128:errorcluster)  [unwired: 1 out]
      n593 = property on="Record/Stop" class="Bool (strict)"(error in=w1128, "Value"=FALSE ("Record/Stop")) -> (error out=w1127:errorcluster)  [unwired: 1 in, 1 out]
      n594 = Flatten To String(anything="Zones presence indicator") -> (data string=w1116:string)  [unwired: 3 in, 2 out]
      n595 = String Length(string=w1116) -> (length=w1115:i32)
      n596 = global write "SW_Globals.vi" "Regions to track"(w1086) -> ()
      n597 = property on="Play/Pause" class="Bool (strict)"(error in=w1127, "Value"=FALSE ("Play/Pause")) -> (error out=w1111:errorcluster)  [unwired: 1 in, 1 out]
      n598 = global write "SW_Globals.vi" "Zone-based stimulus presets"(w978) -> ()
      n599 = property on="Stimulus presets" class="Arr (strict)"("Value"=w978) -> (error out=w1092:errorcluster)  [unwired: 2 in, 1 out]
      n600 = Initialize Array(FALSE, w1115) -> (w1025:bool[])
      "Zones presence array" <- w1025
      n601 = Initialize Array(0, w1115) -> (→"Zones allocation array":i32[])
      n602 = global write "SW_Globals.vi" "Speed detection threshold, mm/s"(1000.0 ("Speed detection threshold, mm/s")) -> ()
      n603 = property on="Stimulus presets" class="Arr (strict)"(error in=w1092, "Index Values"=u32[] [0], "DisabledEnum"=T12."Disabled and Grayed Out" ("Disabled")) -> (error out=w1071:errorcluster)  [unwired: 1 in, 1 out]
      n604 = property on="Record timestamp" class="DigNum (strict)"(error in=w1111, "DisabledEnum"=T12."Disabled and Grayed Out" ("Disabled"), "Value"=0.0 ("Record timestamp")) -> (error out=w1096:errorcluster)  [unwired: 1 in, 1 out]
      n605 = global write "SW_Globals.vi" "Zones presence array"(w1025) -> ()
      n606 = global write "SW_Globals.vi" "Run time threshold, s"(4.0 ("Run time threshold, s")) -> ()
      n607 = global write "SW_Globals.vi" "Run time pause, s"(5.0 ("Run time pause, s")) -> ()
      n608 = global write "SW_Globals.vi" "Run time stim, s"(1.0 ("Run time stim, s")) -> ()
      n609 = property on="Data filtering" class="Ring (strict)"(error in=w1071, "DisabledEnum"=T12."Enabled" ("Disabled")) -> (error out=w1070:errorcluster)  [unwired: 1 in, 1 out]
      n610 = property on="N segments BORDER" class="DigNum (strict)"(error in=w1070) -> (error out=w1097:errorcluster, "Value"=w1101:u8)  [unwired: 1 in, 1 out]
      n611 = property on="N segments MIDFIELD" class="DigNum (strict)"(error in=w1097) -> (error out=w1089:errorcluster, "Value"=w1100:u8)  [unwired: 1 in, 1 out]
      n612 = property on="Zone-based stimulus setup" class="RadioBtnsControl (strict)"(error in=w1089) -> (error out=w1095:errorcluster, "Controls[]"=w1099:refnum<vi>[])  [unwired: 1 in, 1 out]
      n613 = Compound Arithmetic op=ADD(w1101, w1100, u8 1 ("value")) -> (w1098:u8)
      n614 = for {
        tunnel: w1099 -> [w1196] mode=indexing
        tunnel: w1098 -> [w1192]
        tunnel: w1095 -> [w1187]
        tunnel: [w1189] -> w1094
        i -> [w1188]
        n615 = Increment(x=w1188) -> (x+1=w1191:i32)
        n616 = Greater Or Equal?(x=w1192, y=w1191) -> (x >= y?=w1190:bool)
        n617 = Select(t=T12."Enabled" ("Disabled"), s=w1190, f=T12."Disabled and Grayed Out") -> (s? t:f=w1194:T12)
        n618 = property class="Ctl"(reference=w1196, error in=w1187, "DisabledEnum"=w1194) -> (error out=w1189:errorcluster)  [unwired: 1 out]
      }
      n619 = property on="Zone-based stimulus setup" class="RadioBtnsControl (strict)"(error in=w1094, "Value"=T8."No Selection" ("Stim. setup")) -> (error out=w1081:errorcluster)  [unwired: 1 in, 1 out]
      n620 = property on="Pane" class="Pane"(error in=w1081) -> ("Decos[]"=w1080:refnum<vi>[])  [unwired: 1 in, 2 out]
      n621 = Index Array(array=w1080, index=2) -> (element=w1078:refnum<vi>)
      n622 = property class="Decor"(reference=w1078, "Visible"=TRUE) -> ()  [unwired: 1 in, 2 out]
      "Current User" <- w981
      "Start TTL is fired" <- FALSE ("Start/Stop TTL is fired")
      "Stop TTL is fired" <- FALSE ("Start/Stop TTL is fired")
      "Serial port opened" <- FALSE ("Serial port opened")
    }
  }
  n623 = call "SW_SG_coefficients_3-51.vi"("Select filter length"=w8, "Point of interest (can be used for extrapolation)"=0) -> ("SG coefficients"=w7:T37)  [unwired: 1 in]
  n624 = call "SW_SG_coefficients_3-51.vi"("Select filter length"=w12, "Point of interest (can be used for extrapolation)"=0) -> ("SG coefficients"=w10:T37)  [unwired: 1 in]
  n625 = call "SW_SG_coefficients_3-51.vi"("Select filter length"=w16, "Point of interest (can be used for extrapolation)"=0) -> ("SG coefficients"=w13:T37)  [unwired: 1 in]
  n626 = call "SW_SG_coefficients_3-51.vi"("Select filter length"=w6, "Point of interest (can be used for extrapolation)"=0) -> ("SG coefficients"=w4:T37)  [unwired: 1 in]
  n627 = Bundle By Name(cluster=T10 {"SG coefficients 3/5"={"0th order SG coefficients"=[], "1st order SG coefficients"=[]}, "SG coefficients 3/11"={"0th order SG coefficients"=[], "1st order SG coefficients"=[]}, "SG coefficients 3/31"={"0th order SG coefficients"=[], "1st order SG coefficients"=[]}, "SG coefficients 3/51"={"0th order SG coefficients"=[], "1st order SG coefficients"=[]}} ("Input cluster of SG coefficients"), "SG coefficients 3/5"=w13, "SG coefficients 3/11"=w10, "SG coefficients 3/31"=w7, "SG coefficients 3/51"=w4) -> (w14:T10)
  n628 = disable-structure shown="Disabled" {
    disable-tunnel: [w1208 _] -> w24
    disable-tunnel: i64 23 ("Period") -> [w1207 _]
    disable-tunnel: 900 ("Priority") -> [w1206 _]
    disable-tunnel: w20 -> [w1205 _]
    disable-tunnel: w14 -> [w1204 _]
    disable-tunnel: w3 -> [w1203 _]
    disable-tunnel: w2 -> [w1202 _]
    disable-tunnel: [w1201 _] -> w1
    frame Disabled {
      n629 = node-c288(w1203, w1207, w1206) -> (w1210:T13)
      n630 = timed-loop "This loop is all about temporary data processing and streaming to the interface part" {
        tunnel: w1202 -> [w1230]
        tunnel: w1205 -> [w1229]
        tunnel: [w1218] -> w1208
        timing: w1210 -> [_]
        timing-out: [_] -> w1209
        tunnel: w1207 -> [w1217]
        tunnel: w1204 -> [w1212]
        tunnel: [w1211] -> w1201
        i -> [w1228]
        stop <- w1216 stop-if-true
        n631 = node-c288() -> ()  [unwired: 1 in, 1 out]
        n632 = Unbundle By Name(w1230) -> ("Complete stop"=w1231:refnum<notifier>, "Play/Pause status"=w1225:refnum<notifier>)
        n633 = flat-sequence {
          tunnel: w1230 -> [w1236]
          tunnel: w1217 -> [w1246]
          tunnel: w1228 -> [w1245]
          tunnel: w1226 -> [w1244]
          tunnel: w1215 -> [w1243]
          tunnel: [w1242] -> w1224
          tunnel: w1222 -> [w1241]
          tunnel: w1221 -> [w1240]
          tunnel: w1219 -> [w1239]
          tunnel: [w1238] -> w1218
          tunnel: w1213 -> [w1237]
          tunnel: [w1236] -> w1214
          tunnel: w1212 -> [w1235]
          tunnel: [w1234] -> w1211
          tunnel: w1225 -> [w1368]
          tunnel: w1224 -> [w1359]
          tunnel: [w1367] -> w1223
          tunnel: w1214 -> [w1357]
          tunnel: w1213 -> [w1366]
          frame #0 {
            n634 = case shown="\"Play\"" w1241 {
              tunnel: w1236 -> [_ w1333]
              tunnel: w1246 -> [_ w1332]
              tunnel: w1245 -> [_ w1331]
              tunnel: w1244 -> [_ w1330]
              tunnel: w1243 -> [_ w1327]
              tunnel: [w1247 w1314] -> w1242
              tunnel: w1240 -> [w1247 w1323]
              tunnel: w1239 -> [_ w1326]
              tunnel: [_ w1321] -> w1238
              tunnel: w1237 -> [_ w1259]
              tunnel: w1235 -> [_ w1251]
              tunnel: [_ w1248] -> w1234
              frame "Pause", Default {
              }
              frame "Play" {
                w1267 = "." ("string")
                n635 = property on="Bridge horizontal offset" class="DigNum (strict)"() -> ("Value"=w1252:sgl)  [unwired: 2 in, 2 out]
                n636 = global read "SW_Globals.vi" "Alternative magnets orientation"() -> (w1257:bool)
                n637 = property on="Bridge offset" class="DigNum (strict)"() -> ("Value"=w1253:sgl)  [unwired: 2 in, 2 out]
                n638 = property on="Twisted neck" class="Bool (strict)"() -> ("Value"=w1254:bool)  [unwired: 2 in, 2 out]
                n639 = property on="Bridge swap" class="Bool (strict)"(error in=w1323) -> (error out=w1322:errorcluster, "Value"=w1258:bool)  [unwired: 1 in, 1 out]
                n640 = local read "Pixels per mm"() -> (w1324:dbl)
                n641 = Bundle By Name(cluster=T39 {"Offset V."=0.0, "Offset H."=0.0, "Bridge swap"=FALSE, "Turn magnets 90 deg."=FALSE, "Twisted neck"=FALSE} ("Offsets, swaps and rotations"), "Offset V."=w1253, "Offset H."=w1252, "Bridge swap"=w1258, "Turn magnets 90 deg."=w1257, "Twisted neck"=w1254) -> (w1255:T39)
                n642 = property on="Diagram at recording" class="Pict"() -> ("Bounds"=w1325:T19)  [unwired: 2 in, 2 out]
                n643 = call "FL_Preprocess_and_save_incrementally_TDMS.vi"("Temporary file output path"=w1327, "Loop iteration"=w1331, "Offsets, swaps and rotations"=w1255, "Loop speed in ms"=w1332, "Save every N seconds"=u32 8, "error in (no error)"=w1322, "Filter type"="Data filtering", "Sensor read input"=w1330, "Input cluster of SG coefficients"=w1251, "tdms file in"=w1259, "Pixels per mm"=w1324, "Data flow controls in"=w1333, "Diagram at recording bounds"=w1325, "Sensor board size"=w1326) -> ("Eff. save interval"=→"Eff. save interval":sgl, "Latest sensor output (decoded)"=w1249:string[][], "Fire TTL"=w1260:bool, "TTL out N"=w1261:u8, "Current TTL status"=w1306:u8, "error out"=w1315:errorcluster)
                "Current TTL status" <- w1306
                n644 = for {
                  tunnel: w1249 -> [w1337] mode=indexing
                  tunnel: [w1335] -> w1248
                  n645 = call <extravilib>:"Write.vi"("size (unlimited)"=100, "timeout in ms (-1)"=1, "element"=w1337) -> ("channel"=w1335:T40)  [unwired: 6 in, 2 out]
                }
                n646 = Index Array "TTL inputs"(array=w1249, index (col)=14) -> (element=w1308:string[])  [unwired: 1 in]
                n647 = property on="Start/Stop in config" class="DigNum (strict)"() -> ("Value"=w1311:u32)  [unwired: 2 in, 2 out]
                n648 = Decimal String To Number(string=w1308, default (0L)=u8 0 ("default (0 I32)")) -> (number=w1312:u8[])  [unwired: 1 in, 1 out]
                n649 = call <extravilib>:"Write.vi"("size (1)"=5, "lossy behavior (drop oldest)"=Lossy_Behavior."drop oldest element", "element"=w1249) -> ("channel"=w1321:T41)  [unwired: 6 in, 2 out]
                n650 = Greater Than 0?(x=w1311) -> (x > 0?=w1313:bool)
                n651 = Search 1D Array(1D array=w1312, element=w1311) -> (index of element=w1310:i32)  [unwired: 1 in]
                n652 = Greater Or Equal To 0?(x=w1310) -> (x >= 0?=w1309:bool)
                n653 = And(x=w1313, y=w1309) -> (x .and. y?=w1317:bool)
                n654 = case shown="True" w1317 {
                  tunnel: w1308 -> [_ w1356]
                  frame False {
                  }
                  frame True {
                    n655 = call "FL_Get_TTL_in_pulse_length.vi"("Latest sensor input (decoded)"=w1356) -> ("TTL pulse length, ms"=w1355:u32)
                    n656 = global read "SW_Globals.vi" "TTL recording start signal has been successfully reset"() -> (w1346:bool)
                    n657 = global read "SW_Globals.vi" "Recording has been started with TTL"() -> (w1349:bool)
                    n658 = global read "SW_Globals.vi" "Recording has been stopped with TTL"() -> (w1343:bool)
                    n659 = feedback #2(FALSE) -> (w1352:bool)
                    n660 = Not(x=w1352) -> (.not. x?=w1353:bool)
                    n661 = Greater Or Equal?(x=w1355, y=u32 225) -> (x >= y?=w1345:bool)
                    "TTL is long enough" <- w1345
                    n662 = And(x=w1353, y=w1345) -> (x .and. y?=w1350:bool)
                    n663 = Not(x=w1345) -> (.not. x?=w1348:bool)
                    n664 = And(x=w1349, y=w1348) -> (x .and. y?=w1347:bool)
                    n665 = Or(x=w1350, y=w1349) -> (x .or. y?=w1342:bool)
                    "Started" <- w1342
                    n666 = feedback-in #2(w1342) -> ()
                    n667 = Or(x=w1346, y=w1347) -> (x .or. y?=w1341:bool)
                    "Reset starting pulse" <- w1341
                    n668 = global write "SW_Globals.vi" "TTL recording start signal has been successfully reset"(w1341) -> ()
                    n669 = global write "SW_Globals.vi" "Recording has been started with TTL"(w1342) -> ()
                    n670 = Compound Arithmetic op=AND(w1341, w1342, w1345) -> (w1344:bool)
                    n671 = Or(x=w1344, y=w1343) -> (x .or. y?=w1340:bool)
                    "Stopped" <- w1340
                    n672 = Not(x=w1340) -> (.not. x?=w1339:bool)
                    n673 = global write "SW_Globals.vi" "Recording has been stopped with TTL"(w1340) -> ()
                    n674 = Compound Arithmetic op=AND(w1342, w1341, w1339) -> (w1338:bool)
                    "Record" <- w1338
                    n675 = property on="Record/Stop" class="Bool (strict)"("Value"=w1338) -> ()  [unwired: 2 in, 2 out]
                    n676 = property on="TTL REC" class="Bool (strict)"("Value"=w1338) -> ()  [unwired: 2 in, 2 out]
                  }
                }
                n677 = Number To Boolean Array(number=w1306) -> (Boolean array=w1302:bool[])
                n678 = Index Array(array=w1302, index=0) -> (element=w1294:bool)
                "TTL IO 1 (recording)" <- w1294
                n679 = Index Array(array=w1302, index=1) -> (element=w1274:bool)
                "TTL IO 2 (recording)" <- w1274
                n680 = Index Array(array=w1302, index=2) -> (element=w1273:bool)
                "TTL IO 3 (recording)" <- w1273
                n681 = Index Array(array=w1302, index=3) -> (element=w1275:bool)
                "TTL IO 4 (recording)" <- w1275
                n682 = feedback #3(TRUE) -> (w1277:bool)
                n683 = feedback-in #3(w1275) -> ()
                n684 = feedback #4(TRUE) -> (w1287:bool)
                n685 = feedback-in #4(w1273) -> ()
                n686 = feedback #5(TRUE) -> (w1299:bool)
                n687 = feedback-in #5(w1294) -> ()
                n688 = feedback #6(TRUE) -> (w1288:bool)
                n689 = feedback-in #6(w1274) -> ()
                n690 = Not(x=w1277) -> (.not. x?=w1278:bool)
                n691 = Not(x=w1287) -> (.not. x?=w1285:bool)
                n692 = Not(x=w1299) -> (.not. x?=w1298:bool)
                n693 = Not(x=w1288) -> (.not. x?=w1290:bool)
                n694 = local read "TTL 4 counter"() -> (w1280:u32)
                n695 = And(x=w1278, y=w1275) -> (x .and. y?=w1279:bool)
                n696 = local read "TTL 3 counter"() -> (w1283:u32)
                n697 = local read "TTL 1 counter"() -> (w1296:u32)
                n698 = local read "TTL 2 counter"() -> (w1292:u32)
                n699 = And(x=w1285, y=w1273) -> (x .and. y?=w1284:bool)
                n700 = And(x=w1298, y=w1294) -> (x .and. y?=w1297:bool)
                n701 = And(x=w1290, y=w1274) -> (x .and. y?=w1291:bool)
                n702 = Increment(x=w1280) -> (x+1=w1281:u32)
                n703 = Increment(x=w1283) -> (x+1=w1282:u32)
                n704 = Increment(x=w1296) -> (x+1=w1295:u32)
                n705 = Select(t=w1281, s=w1279, f=w1280) -> (s? t:f=w1269:u32)
                "TTL 4 counter" <- w1269
                n706 = Increment(x=w1292) -> (x+1=w1293:u32)
                n707 = Select(t=w1282, s=w1284, f=w1283) -> (s? t:f=w1270:u32)
                "TTL 3 counter" <- w1270
                n708 = Select(t=w1295, s=w1297, f=w1296) -> (s? t:f=w1272:u32)
                "TTL 1 counter" <- w1272
                n709 = Select(t=w1293, s=w1291, f=w1292) -> (s? t:f=w1271:u32)
                "TTL 2 counter" <- w1271
                n710 = Number To Decimal String(number=w1272) -> (decimal integer string=w1268:string)  [unwired: 1 in]
                n711 = Number To Decimal String(number=w1271) -> (decimal integer string=w1266:string)  [unwired: 1 in]
                n712 = Number To Decimal String(number=w1270) -> (decimal integer string=w1265:string)  [unwired: 1 in]
                n713 = Number To Decimal String(number=w1269) -> (decimal integer string=w1264:string)  [unwired: 1 in]
                n714 = global read "SW_Globals.vi" "IO inversion config."() -> (w1262:u16)
                n715 = global read "SW_Globals.vi" "VISA resource name"() -> (w1316:refnum<visa-resource-name>)
                n716 = call "SW_Fire_TTL_during_the_acquisition_universal.vi"("IO inversion config."=w1262, "error in (no error)"=w1315, "Serial Port In"=w1316, "TTL port(s) config to fire"=w1261, "Fire TTL"=w1260) -> ("error out"=w1314:errorcluster)  [unwired: 6 in]
                n717 = Concatenate Strings(w1268, w1267, w1266, w1267, w1265, w1267, w1264) -> (→"IO pulses count":string)
              }
            }
          }
          frame #1 {
            n718 = Unbundle By Name(w1357) -> ("Recording now"=w1365:refnum<notifier>, "Has been recorded"=w1364:refnum<notifier>)
            n719 = Get Notifier Status(notifier=w1364) -> (current notification=w1362:bool)  [unwired: 1 in, 4 out]
            n720 = Get Notifier Status(notifier=w1365) -> (current notification=w1363:bool)  [unwired: 1 in, 4 out]
            n721 = Not(x=w1363) -> (.not. x?=w1361:bool)
            n722 = And(x=w1362, y=w1361) -> (x .and. y?=w1360:bool)
            n723 = case shown="True" w1360 {
              tunnel: w1366 -> [_ w1378]
              tunnel: w1359 -> [w1369 w1377]
              tunnel: [w1369 w1370] -> w1358
              tunnel: w1357 -> [_ w1374]
              frame False {
              }
              frame True {
                n724 = Unbundle By Name(w1374) -> ("(Final) Data file is saved"=w1373:refnum<notifier>)
                n725 = TDMS Close(8:w1377, 11:w1378) -> (0:w1376:errorcluster)  [unwired: 1 out]
                n726 = call <vilib>:"Clear Errors.vi"("error in (no error)"=w1376, "specific error code to clear (0: all)"=-2501) -> ("error out"=w1371:errorcluster)  [unwired: 4 in, 1 out]
                n727 = Send Notification(notification=TRUE, notifier=w1373, error in (no error)=w1371) -> (error out=w1370:errorcluster)  [unwired: 1 out]
              }
            }
            n728 = Get Notifier Status(notifier=w1368, error in (no error)=w1358) -> (current notification=w1367:string)  [unwired: 4 out]
          }
        }
        n729 = Flush Queue(queue=w1229) -> (remaining elements=w1226:T42, error out=w1221:errorcluster)  [unwired: 1 in, 1 out]
        n730 = local read "Board size"() -> (w1219:string)
        n731 = global read "SW_Globals.vi" "Cluster of paths"() -> (w1227:T22)
        n732 = Get Notifier Status(notifier=w1231) -> (current notification=w1216:bool)  [unwired: 1 in, 4 out]
        n733 = Unbundle By Name(w1227) -> ("Temporary file output path"=w1215:path, "TDMS file reference"=w1213:refnum<k34>)
        n734 = feedback-in #7(w1223) -> ()
        n735 = feedback #7("Pause" ("String")) -> (w1222:string)
        n736 = node-c288() -> ()  [unwired: 1 in, 1 out]
      }
      n737 = node-c288(w1209) -> ()  [unwired: 1 out]
    }
    frame Enabled {
    }
  }
  n738 = disable-structure shown="Disabled" {
    disable-tunnel: w3 -> [w1394 _]
    disable-tunnel: w2 -> [w1393 _]
    disable-tunnel: w1 -> [w1392 _]
    frame Disabled {
      n739 = node-c288(w1394, i64 2 ("Period"), 100 ("Priority"), 1000 ("Timeout")) -> (w1396:T13)  [unwired: 1 in]
      n740 = timed-loop {
        timing: w1396 -> [_]
        timing-out: [_] -> w1395
        tunnel: w1393 -> [w1398]
        tunnel: w1392 -> [w1399]
        stop <- w1397 stop-if-true
        n741 = node-c288() -> ()  [unwired: 1 in, 1 out]
        n742 = Unbundle By Name(w1398) -> ("Complete stop"=w1402:refnum<notifier>)
        n743 = Get Notifier Status(notifier=w1402) -> (current notification=w1397:bool)  [unwired: 1 in, 4 out]
        n744 = event shown="[2] \"Open serial port\": Value Change" {
          selector: _ -> [_ _ _]
          dyn-events: _ -> [_ _ _]
          timeout: 0 -> [_ _ _]
          event Timeout {
            n745 = event-data() -> ()  [unwired: 1 in, 3 out]
          }
          event "Expand/hide stream panel (Rec)": Value Change {
            n746 = event-data() -> ("NewVal"=w1438:bool)  [unwired: 1 in, 5 out]
            n747 = case shown="True" w1438 {
              tunnel: [w1443 w1458] -> w1437
              tunnel: 120 ("y") -> [w1439 w1454]
              frame True {
                n748 = property on="Main tab control" class="TabCtl (strict)"() -> ("PaneHeight"=w1451:u32)  [unwired: 2 in, 2 out]
                n749 = Current VI's Path() -> (path=w1449:path)
                n750 = property on="Expand/hide stream panel (Rec)" class="Bool (strict)"() -> ("Top"=w1453:i32)  [unwired: 2 in, 2 out]
                n751 = Open VI Reference(vi path=w1449) -> (vi reference=w1448:refnum<vi>, error out=w1447:errorcluster)  [unwired: 5 in]
                n752 = Add(x=w1453, y=w1439) -> (x+y=w1452:i32)
                n753 = property class="VI"(reference=w1448, error in=w1447) -> (reference out=w1445:refnum<vi>, error out=w1444:errorcluster, "Front Panel.PanelBounds"=w1442:T43)
                n754 = Add(x=w1451, y=w1439) -> (x+y=w1450:u32)
                n755 = property on="Expand/hide stream panel (Rec)" class="Bool (strict)"("Top"=w1452) -> ()  [unwired: 2 in, 2 out]
                n756 = property on="Main tab control" class="TabCtl (strict)"("PaneHeight"=w1450) -> ()  [unwired: 2 in, 2 out]
                n757 = Unbundle By Name(w1442) -> ("Bottom"=w1446:i16)
                n758 = Add(x=w1446, y=w1439) -> (x+y=w1441:i32)
                n759 = Bundle By Name(cluster=w1442, "Bottom"=w1441) -> (w1440:T43)
                n760 = property class="VI"(reference=w1445, error in=w1444, "Front Panel.PanelBounds"=w1440) -> (error out=w1443:errorcluster)  [unwired: 1 out]
              }
              frame False {
                n761 = property on="Main tab control" class="TabCtl (strict)"() -> ("PaneHeight"=w1466:u32)  [unwired: 2 in, 2 out]
                n762 = Current VI's Path() -> (path=w1464:path)
                n763 = property on="Expand/hide stream panel (Rec)" class="Bool (strict)"() -> ("Top"=w1468:i32)  [unwired: 2 in, 2 out]
                n764 = Open VI Reference(vi path=w1464) -> (vi reference=w1463:refnum<vi>, error out=w1462:errorcluster)  [unwired: 5 in]
                n765 = Subtract(x=w1468, y=w1454) -> (x-y=w1467:i32)
                n766 = property class="VI"(reference=w1463, error in=w1462) -> (reference out=w1460:refnum<vi>, error out=w1459:errorcluster, "Front Panel.PanelBounds"=w1457:T43)
                n767 = Subtract(x=w1466, y=w1454) -> (x-y=w1465:u32)
                n768 = property on="Expand/hide stream panel (Rec)" class="Bool (strict)"("Top"=w1467) -> ()  [unwired: 2 in, 2 out]
                n769 = property on="Main tab control" class="TabCtl (strict)"("PaneHeight"=w1465) -> ()  [unwired: 2 in, 2 out]
                n770 = Unbundle By Name(w1457) -> ("Bottom"=w1461:i16)
                n771 = Subtract(x=w1461, y=w1454) -> (x-y=w1456:i32)
                n772 = Bundle By Name(cluster=w1457, "Bottom"=w1456) -> (w1455:T43)
                n773 = property class="VI"(reference=w1460, error in=w1459, "Front Panel.PanelBounds"=w1455) -> (error out=w1458:errorcluster)  [unwired: 1 out]
              }
            }
            "FP size change error" <- w1437
          }
          event "Open serial port": Value Change {
            n774 = event-data() -> ()  [unwired: 1 in, 6 out]
            n775 = property on="Serial port opened" class="Bool (strict)"() -> ("Value"=w1469:bool)  [unwired: 2 in, 2 out]
            n776 = case shown="True" w1469 {
              frame False {
                w1475 = T44 4 items=["VISA Defaults"=0, "Exclusive Lock"=1, "Load Configured Settings"=4] ("Access Mode")
                n777 = property on="Serial OUT name" class="VISAName"("DisabledEnum"=T12."Disabled and Grayed Out" ("Disabled")) -> ("Value"=w1471:refnum<visa-resource-name>)  [unwired: 2 in, 2 out]
                n778 = VISA Open(access mode=w1475, VISA resource name=w1471) -> (VISA resource name=w1476:refnum<visa-resource-name>, error out=w1477:errorcluster)  [unwired: 3 in]
                n779 = property class="Instr"(reference=w1476, error in=w1477, "General Settings:Timeout Value"=u32 10) -> (reference out=w1472:refnum<visa-resource-name>, error out=w1473:errorcluster)
                n780 = case shown="Error" w1473 {
                  tunnel: w1472 -> [_ w1485]
                  frame No Error {
                    w1478 = T11 [{"Numeric Control"=6603023, "Numeric Control"=6603023}, {"Numeric Control"=3381555, "Numeric Control"=3381555}, {"Numeric Control"=1976113, "Numeric Control"=8355711}, {"Numeric Control"=3355443, "Numeric Control"=6710886}]  # Button port ON colors
                    n781 = property on="Expand/hide stream panel (Rec)" class="Bool (strict)"("Colors [4]"=w1478) -> ()  [unwired: 2 in, 2 out]
                    n782 = property on="Serial port opened" class="Bool (strict)"("Value"=TRUE ("Serial port opened")) -> ()  [unwired: 2 in, 2 out]
                    n783 = property on="Streaming" class="Bool (strict)"("DisabledEnum"=T12."Enabled" ("Disabled"), "Value"=FALSE ("Streaming")) -> ()  [unwired: 2 in, 2 out]
                  }
                  frame Error {
                    w1482 = T11 [{"Numeric Control"=12369084, "Numeric Control"=12369084}, {"Numeric Control"=16757760, "Numeric Control"=16757760}, {"Numeric Control"=1976113, "Numeric Control"=8355711}, {"Numeric Control"=3355443, "Numeric Control"=6710886}]  # Button port OFF colors
                    w1483 = FALSE ("Serial port opened")
                    n784 = property on="Expand/hide stream panel (Rec)" class="Bool (strict)"("Colors [4]"=w1482) -> ()  [unwired: 2 in, 2 out]
                    n785 = Not A Number/Path/Refnum?(number/path/refnum=w1485) -> (NaN/Path/Refnum?=w1486:bool)
                    n786 = case shown="False" w1486 {
                      tunnel: w1485 -> [w1487 _]
                      frame False {
                        n787 = VISA Close(VISA resource name=w1487) -> ()  [unwired: 1 in, 1 out]
                      }
                      frame True {
                      }
                    }
                    n788 = property on="Serial port opened" class="Bool (strict)"("Value"=w1483) -> ()  [unwired: 2 in, 2 out]
                    n789 = property on="Streaming" class="Bool (strict)"("DisabledEnum"=T12."Disabled and Grayed Out" ("Disabled"), "Value"=w1483) -> ()  [unwired: 2 in, 2 out]
                  }
                }
              }
              frame True {
                w1488 = T11 [{"Numeric Control"=12369084, "Numeric Control"=12369084}, {"Numeric Control"=16757760, "Numeric Control"=16757760}, {"Numeric Control"=1976113, "Numeric Control"=8355711}, {"Numeric Control"=3355443, "Numeric Control"=6710886}]  # Button port OFF colors
                w1493 = FALSE ("Serial port opened")
                n790 = property on="Serial OUT name" class="VISAName"("DisabledEnum"=T12."Enabled" ("Disabled")) -> (error out=w1491:errorcluster, "Value"=w1492:refnum<visa-resource-name>)  [unwired: 2 in, 1 out]
                n791 = property on="Serial port opened" class="Bool (strict)"("Value"=w1493) -> ()  [unwired: 2 in, 2 out]
                n792 = VISA Close(VISA resource name=w1492, error in (no error)=w1491) -> (error out=w1490:errorcluster)
                n793 = property on="Streaming" class="Bool (strict)"("DisabledEnum"=T12."Disabled and Grayed Out" ("Disabled"), "Value"=w1493) -> ()  [unwired: 2 in, 2 out]
                n794 = property on="VISA streaming error out" class="Clust (strict)"("Value"=w1490) -> (error out=w1489:errorcluster)  [unwired: 2 in, 1 out]
                n795 = property on="Expand/hide stream panel (Rec)" class="Bool (strict)"(error in=w1489, "Colors [4]"=w1488) -> ()  [unwired: 1 in, 2 out]
              }
            }
          }
        }
        n796 = property on="Serial port opened" class="Bool (strict)"() -> ("Value"=w1400:bool)  [unwired: 2 in, 2 out]
        n797 = case shown="True" w1400 {
          tunnel: w1399 -> [_ w1431]
          tunnel: w1398 -> [_ w1408]
          frame False {
          }
          frame True {
            w1413 = "\t"
            n798 = Unbundle By Name(w1408) -> ("Recording now"=w1407:refnum<notifier>)
            n799 = call <extravilib>:"Read.vi"("channel"=w1431) -> ("element"=w1411:string[])  [unwired: 6 in, 4 out]
            "Latest frame" <- w1411
            n800 = Index Array "Timestamp"(array=w1411, index=5) -> (element=w1404:string)
            n801 = Index Array "R"(array=w1411, index=6) -> (element=w1425:string)
            n802 = Index Array "phi"(array=w1411, index=7) -> (element=w1424:string)
            n803 = Index Array "X"(array=w1411, index=9) -> (element=w1418:string)
            n804 = Index Array "w"(array=w1411, index=11) -> (element=w1416:string)
            n805 = Index Array "Y"(array=w1411, index=10) -> (element=w1417:string)
            n806 = Index Array "alpha"(array=w1411, index=8) -> (element=w1419:string)
            n807 = Index Array "Zone"(array=w1411, index=12) -> (element=w1414:string)
            n808 = Get Notifier Status(notifier=w1407) -> (current notification=w1405:bool)  [unwired: 1 in, 4 out]
            n809 = Select(t=w1404, s=w1405, f="00:00:00.000") -> (s? t:f=w1406:string)
            n810 = property on="Streaming" class="Bool (strict)"() -> ("Value"=w1429:bool)  [unwired: 2 in, 2 out]
            n811 = Index Array "Speed"(array=w1411, index=16) -> (element=w1410:string)
            n812 = Concatenate Strings(w1406, w1413, w1425, w1413, w1424, w1413, w1419, w1413, w1418, w1413, w1417, w1413, w1416, w1413, w1414, w1413, w1410, "\r\n") -> (w1428:string)
            n813 = property on="Output to the external terminal" class="Str"("Value"=w1428) -> ()  [unwired: 2 in, 2 out]
            n814 = case shown="True" w1429 {
              tunnel: w1428 -> [_ w1434]
              frame False {
              }
              frame True {
                n815 = property on="Serial OUT name" class="VISAName"() -> ("Value"=w1433:refnum<visa-resource-name>)  [unwired: 2 in, 2 out]
                n816 = VISA Write(VISA resource name=w1433, write buffer=w1434) -> (return count=→"Last send packet size, bytes":u32, error out=→"VISA streaming error out":errorcluster)  [unwired: 1 in, 1 out]
              }
            }
          }
        }
        n817 = node-c288() -> ()  [unwired: 1 in, 1 out]
      }
      n818 = node-c288(w1395) -> (w1389:errorcluster)
      n819 = property on="Serial OUT name" class="VISAName"(error in=w1389) -> (error out=w1386:errorcluster, "Value"=w1387:refnum<visa-resource-name>)  [unwired: 1 in, 1 out]
      n820 = VISA Close(VISA resource name=w1387, error in (no error)=w1386) -> (error out=→"Timed structure (Streaming) and VISA error(s)":errorcluster)
    }
    frame Enabled {
    }
  }
  n821 = Tick Count (ms)() -> (millisecond timer value=w25:u32)
  n822 = disable-structure shown="Disabled" {
    disable-tunnel: w25 -> [w1513 _]
    disable-tunnel: w24 -> [w1512 _]
    disable-tunnel: w20 -> [w1510 _]
    disable-tunnel: w19 -> [w1509 _]
    disable-tunnel: w3 -> [w1507 _]
    disable-tunnel: w2 -> [w1506 _]
    frame Disabled {
      w1511 = i64 37 ("Period")
      n823 = node-c288(w1507, w1511, 200 ("Priority")) -> (w1515:T13)  [unwired: 1 in]
      n824 = timed-loop {
        tunnel: w1510 -> [w1529]
        tunnel: w1506 -> [w1516]
        tunnel: w1509 -> [w1527]
        tunnel: w1513 -> [w1526]
        tunnel: w1512 -> [w1525]
        timing: w1515 -> [_]
        timing-out: [_] -> w1514
        tunnel: w1511 -> [w1518]
        i -> [w1528]
        stop <- w1522 stop-if-true
        n825 = node-c288() -> ()  [unwired: 1 in, 1 out]
        n826 = Unbundle By Name(w1516) -> ("Complete stop"=w1523:refnum<notifier>)
        n827 = property on="Main tab control" class="TabCtl (strict)"(error in=w1527) -> (error out=w1517:errorcluster, "Value"=w1530:enum32{"Settings", "Recording", "Analysis"})  [unwired: 1 in, 1 out]
        n828 = Send Notification(notification="Stop Button", notifier=w1523) -> (notifier out=w1519:refnum<notifier>, error out=w1520:errorcluster)  [unwired: 1 in]
        n829 = case shown="\"Settings\", Default" w1530 {
          tunnel: w1517 -> [w1537 _ _]
          tunnel: w1529 -> [_ w2280 _]
          tunnel: w1518 -> [_ w2282 w2767]
          tunnel: w1528 -> [_ _ _]
          tunnel: w1516 -> [w1533 w2215 w2769]
          tunnel: w1526 -> [_ w2277 _]
          tunnel: w1525 -> [_ w2270 _]
          frame "Settings", Default {
            n830 = flat-sequence {
              tunnel: w1537 -> [w1541]
              tunnel: [w1541] -> w1534
              tunnel: [w1588] -> w1535
              tunnel: w1534 -> [w1588]
              tunnel: [w1947] -> w1536
              tunnel: w1535 -> [w1947]
              tunnel: w1536 -> [w1989]
              tunnel: w1533 -> [w1984]
              frame #0 {
                n831 = property on="IO paramaters loaded from file" class="Bool (strict)"() -> ("Value"=w1538:bool)  [unwired: 2 in, 2 out]
                n832 = Or(x="Set IO config", y=w1538) -> (x .or. y?=w1539:bool)
                n833 = case shown="True" w1539 {
                  tunnel: w1538 -> [_ w1543]
                  frame False {
                  }
                  frame True {
                    w1555 = u16 4 ("y")
                    n834 = global read "SW_Globals.vi" "IO parameters cluster"() -> (w1549:T2)
                    n835 = local read "Sync capability"() -> (w1548:u8)
                    n836 = case shown="False" w1543 {
                      tunnel: w1549 -> [w1575 w1578]
                      tunnel: w1548 -> [w1576 _]
                      tunnel: [w1574 w1579] -> w1547
                      tunnel: [w1573 w1577] -> w1546
                      frame False {
                        n837 = call "HW_set_IO_ports_3-pos.vi"("Sync capability"=w1576, "Sync parameters cluster input"=w1575) -> ("Sync parameters cluster output"=w1574:T2)
                        n838 = Equal?(x=w1575, y=w1574) -> (x = y?=w1573:T48)
                      }
                      frame True {
                        n839 = property on="IO parameters loaded cluster" class="Clust (strict)"() -> ("Value"=w1579:T2)  [unwired: 2 in, 2 out]
                        n840 = Equal?(x=w1578, y=w1579) -> (x = y?=w1577:T48)
                      }
                    }
                    n841 = Greater Than 0?(x=w1548) -> (x > 0?=w1558:bool)
                    n842 = global read "SW_Globals.vi" "VISA resource name"() -> (w1551:refnum<visa-resource-name>)
                    n843 = Unbundle By Name(w1547) -> ("IO 1 configuration"=w1553:u16, "IO 2 configuration"=w1554:u16)
                    n844 = global write "SW_Globals.vi" "IO parameters cluster"(w1547) -> ()
                    n845 = Cluster To Array(cluster=w1547) -> (array=w1542:u16[])
                    n846 = call "SW_get_IO_ports_representation.vi"("Sync parameters cluster input"=w1547) -> ("IO status indicator"=w1570:T6)
                    n847 = call "SW_get_config_for_Start_Stop_pulses.vi"("Sync parameters cluster input"=w1547) -> ("Start/Stop out pulses config"=w1564:u32, "Start/Stop in config"=w1563:u32, "Start/Stop in config bin"=w1562:bool[], "Start/Stop out pulses config bin"=w1561:bool[])
                    n848 = call "SW_get_config_of_Zones_and_IO.vi"("Sync parameters cluster input"=w1547) -> ("Zones out config bin"=w1560:bool[], "Ports IO config (OUT is FALSE)"=w1559:bool[], "IO inversion config."=w1550:u16)  [unwired: 1 out]
                    n849 = property on="Start/Stop out pulses config" class="DigNum (strict)"("Value"=w1564) -> ()  [unwired: 2 in, 2 out]
                    n850 = property on="Start/Stop in config" class="DigNum (strict)"("Value"=w1563) -> ()  [unwired: 2 in, 2 out]
                    n851 = global write "SW_Globals.vi" "Start/Stop in config bin"(w1562) -> ()
                    n852 = global write "SW_Globals.vi" "Start/Stop out pulses config bin"(w1561) -> ()
                    n853 = global write "SW_Globals.vi" "Zones out config bin"(w1560) -> ()
                    n854 = global write "SW_Globals.vi" "IO ports config"(w1559) -> ()
                    n855 = global write "SW_Globals.vi" "IO inversion config."(w1550) -> ()
                    n856 = Equal?(x=w1553, y=w1555) -> (x = y?=w1556:bool)
                    n857 = Equal?(x=w1554, y=w1555) -> (x = y?=w1557:bool)
                    n858 = call "HW_Set_IO_Dir_on_ECU.vi"("IO ports config"=w1559, "VISA resource name"=w1551, "IO inversion config."=w1550) -> ("error out"=w1552:errorcluster)  [unwired: 1 in, 1 out]
                    n859 = Cluster To Array(cluster=w1546) -> (array=w1568:bool[])
                    n860 = To Variant(anything=w1570) -> (Variant=w1569:variant)
                    n861 = Flatten To JSON(anything=w1542) -> (JSON string=w1572:string, 11:w1571:errorcluster)  [unwired: 2 in]
                    n862 = case shown="True" w1558 {
                      tunnel: w1551 -> [_ w1582]
                      tunnel: w1552 -> [_ w1583]
                      tunnel: w1556 -> [_ w1581]
                      tunnel: w1557 -> [_ w1580]
                      frame False {
                      }
                      frame True {
                        n863 = call "SW_Set_SYNC_Status.vi"("error in (no error)"=w1583, "SYNC 2"=w1581, "SYNC 1"=w1580, "VISA Resource name IN"=w1582) -> ()  [unwired: 6 in, 2 out]
                      }
                    }
                    n864 = property on="IO status indicator" class="Clust"("Value"=w1569) -> ()  [unwired: 2 in, 2 out]
                    n865 = property on="IO parameters string" class="Str"(error in=w1571, "Value"=w1572) -> ()  [unwired: 1 in, 2 out]
                    n866 = Not(x=w1568) -> (.not. x?=w1567:bool[])
                    n867 = Boolean Array To Number(Boolean array=w1567) -> (number=w1566:u32)
                    n868 = Not(x=w1543) -> (.not. x?=w1544:bool)
                    n869 = Greater Than 0?(x=w1566) -> (x > 0?=w1565:bool)
                    n870 = And(x=w1565, y=w1544) -> (x .and. y?=w1545:bool)
                    n871 = case shown="False" w1545 {
                      frame False {
                        n872 = property on="IO paramaters loaded from file" class="Bool (strict)"("Value"=FALSE ("IO paramaters loaded from file")) -> ()  [unwired: 2 in, 2 out]
                      }
                      frame True {
                        n873 = property on="IO paramaters loaded from file" class="Bool (strict)"("Value"=FALSE ("IO paramaters loaded from file")) -> ()  [unwired: 2 in, 2 out]
                        n874 = property on="Changed IO" class="Bool (strict)"("Val(Sgnl)"=TRUE ("Value (Signaling)")) -> ()  [unwired: 2 in, 2 out]
                      }
                    }
                  }
                }
              }
              frame #1 {
                n875 = event shown="[2] \"N segments BORDER\", \"N segments MIDFIELD\": Value Change" {
                  selector: _ -> [_ _ _ _ _ _ _ _ _]
                  dyn-events: _ -> [_ _ _ _ _ _ _ _ _]
                  timeout: 1 -> [_ _ _ _ _ _ _ _ _]
                  event Timeout {
                    n876 = event-data() -> ()  [unwired: 1 in, 3 out]
                  }
                  event "Segments diagram": Mouse Down {
                    n877 = event-data() -> ("Coords"=→"Coords":T4, "Button"=→"Button":u16)  [unwired: 1 in, 6 out]
                  }
                  event "N segments BORDER", "N segments MIDFIELD": Value Change {
                    n878 = event-data() -> ()  [unwired: 1 in, 6 out]
                    n879 = global read "SW_Globals.vi" "IO parameters cluster"() -> (w1600:T2)
                    n880 = Unbundle By Name(w1600) -> ("SYNC configuration"=w1599:u16, "IO 1 configuration"=w1596:u16, "IO 2 configuration"=w1595:u16)
                    n881 = property on="N segments BORDER" class="DigNum (strict)"() -> (error out=w1605:errorcluster, "Value"=w1608:u8)  [unwired: 2 in, 1 out]
                    n882 = call "SW_Gen_Available_TTL_outputs_array.vi"("IO 2 configuration"=w1595, "IO 1 configuration"=w1596, "SYNC configuration"=w1599) -> ("Available TTL outputs array"=w1594:cluster{"String":string, "Value":i32}[])
                    n883 = property on="N segments MIDFIELD" class="DigNum (strict)"(error in=w1605) -> (error out=w1604:errorcluster, "Value"=w1607:u8)  [unwired: 1 in, 1 out]
                    n884 = Index Array(array=w1594, index=0) -> (element=w1597:cluster{"String":string, "Value":i32})
                    n885 = global read "SW_Globals.vi" "Zone-based stimulus presets"() -> (w1602:T49)
                    n886 = property on="TTL out" class="Ring (strict)"("StringsAndValues[]"=w1594) -> ()  [unwired: 2 in, 2 out]
                    n887 = property on="Zone-based stimulus setup" class="RadioBtnsControl (strict)"(error in=w1604) -> ("Controls[]"=w1606:refnum<vi>[])  [unwired: 1 in, 2 out]
                    n888 = Compound Arithmetic op=ADD(w1608, w1607, u8 1 ("value")) -> (w1603:u8)
                    n889 = Unbundle By Name(w1597) -> ("Value"=w1601:i32)
                    n890 = for {
                      tunnel: w1606 -> [w1625] mode=indexing
                      tunnel: w1603 -> [w1616]
                      tunnel: w1602 -> [w1621]
                      tunnel: w1601 -> [w1620]
                      tunnel: [w1619] -> w1592 mode=indexing
                      i -> [w1615]
                      n891 = Increment(x=w1615) -> (x+1=w1617:i32)
                      n892 = Greater Or Equal?(x=w1616, y=w1617) -> (x >= y?=w1614:bool)
                      n893 = Select(t=T12."Enabled" ("Disabled"), s=w1614, f=T12."Disabled and Grayed Out") -> (s? t:f=w1623:T12)
                      n894 = property class="Ctl"(reference=w1625, "DisabledEnum"=w1623) -> (reference out=w1618:refnum<vi>)  [unwired: 1 in, 1 out]
                      n895 = case shown="True" w1614 {
                        tunnel: w1621 -> [_ w1635]
                        tunnel: w1620 -> [w1633 _]
                        tunnel: [w1631 w1634] -> w1619
                        tunnel: w1618 -> [w1626 _]
                        frame False {
                          w1628 = refnum<vi> refnum  # Boolean
                          n896 = Bundle By Name(cluster=T45 {"Event type"=0, "Cond., s"=0.0, "Stim., s"=0.0, "Set/Clear"=FALSE, "TTL out N"=1, "Stim. has been set"=FALSE} ("Cluster of the stimuls settings"), "TTL out N"=w1633) -> (w1631:T45)
                          n897 = To More Specific Class(target class=w1628, reference=w1626) -> (specific class reference=w1627:refnum<vi>)  [unwired: 1 in, 1 out]
                          n898 = property class="Bool"(reference=w1627, "Colors [4]"=T11 [{"Numeric Control"=12369084, "Numeric Control"=12369084}, {"Numeric Control"=6603023, "Numeric Control"=6603023}, {"Numeric Control"=1976113, "Numeric Control"=1976113}, {"Numeric Control"=2575993, "Numeric Control"=2575993}] ("Colors [4] 2"), "Value"=FALSE) -> ()  [unwired: 1 in, 2 out]
                        }
                        frame True {
                          n899 = Index Array(array=w1635) -> (element=w1634:T45)  [unwired: 1 in]
                        }
                      }
                    }
                    n900 = for {
                      tunnel: w1592 -> [w1613] mode=indexing
                      tunnel: [w1610] -> w1593 mode=indexing if=w1611
                      i -> [w1612]
                      n901 = Unbundle By Name(w1613) -> ("Stim. has been set"=w1611:bool)
                      n902 = To Unsigned Byte Integer(number=w1612) -> (unsigned 8bit integer=w1610:u8)
                    }
                    n903 = global write "SW_Globals.vi" "Zone-based stimulus presets"(w1592) -> ()
                    n904 = property on="Stimulus presets" class="Arr (strict)"("Value"=w1592) -> ()  [unwired: 2 in, 2 out]
                    n905 = global write "SW_Globals.vi" "Regions to track"(w1593) -> ()
                  }
                  event "Zone-based stimulus setup": Value Change {
                    n906 = event-data() -> ("NewVal"=w1637:T8)  [unwired: 1 in, 5 out]
                    n907 = To Unsigned Byte Integer(number=w1637) -> (unsigned 8bit integer=w1636:u8)
                    n908 = case shown="1.." w1636 {
                      selector: w1636 -> [w1638 w1641]
                      frame 0, Default {
                        n909 = Build Array(w1638) -> (w1640:u8[])
                        n910 = property on="Stimulus presets" class="Arr (strict)"("Index Values"=w1640, "DisabledEnum"=T12."Disabled and Grayed Out" ("Disabled")) -> ()  [unwired: 2 in, 2 out]
                      }
                      frame 1.. {
                        n911 = Build Array(w1641) -> (w1643:u8[])
                        n912 = property on="Stimulus presets" class="Arr (strict)"("Index Values"=w1643, "DisabledEnum"=T12."Enabled" ("Disabled")) -> ()  [unwired: 2 in, 2 out]
                      }
                    }
                  }
                  event "Stimulus presets", "Adv. Stim. set": Value Change {
                    n913 = event-data() -> ()  [unwired: 1 in, 6 out]
                    n914 = property on="Stimulus presets" class="Arr (strict)"() -> ("Value"=w1647:T7)  [unwired: 2 in, 2 out]
                    n915 = disable-structure shown="Disabled" {
                      frame Disabled {
                        n916 = case shown="1" {
                          selector: _ -> [_ _ _ _ _ _ _ _ _ _ _ _ _ _]
                          tunnel: _ -> [_ w1674 w1678 w1682 w1686 w1690 w1694 w1698 w1702 w1706 w1710 w1714 w1718 w1722]
                          frame 0, Default {
                          }
                          frame 1 {
                            n917 = property on="Colors for Stim. setup" class="Arr (strict)"() -> ("Value"=w1673:T3)  [unwired: 2 in, 2 out]
                            n918 = Select(t=w1673, s=w1674, f=T11 [{"Numeric Control"=12369084, "Numeric Control"=12369084}, {"Numeric Control"=6603023, "Numeric Control"=6603023}, {"Numeric Control"=1976113, "Numeric Control"=1976113}, {"Numeric Control"=2575993, "Numeric Control"=2575993}] ("Colors [4] 2")) -> (s? t:f=w1676:T11)
                            n919 = property on="Zone 01" class="Bool (strict)"("Colors [4]"=w1676) -> ()  [unwired: 2 in, 2 out]
                          }
                          frame 2 {
                            n920 = property on="Colors for Stim. setup" class="Arr (strict)"() -> ("Value"=w1677:T3)  [unwired: 2 in, 2 out]
                            n921 = Select(t=w1677, s=w1678, f=T11 [{"Numeric Control"=12369084, "Numeric Control"=12369084}, {"Numeric Control"=6603023, "Numeric Control"=6603023}, {"Numeric Control"=1976113, "Numeric Control"=1976113}, {"Numeric Control"=2575993, "Numeric Control"=2575993}] ("Colors [4] 2")) -> (s? t:f=w1680:T11)
                            n922 = property on="Zone 02" class="Bool (strict)"("Colors [4]"=w1680) -> ()  [unwired: 2 in, 2 out]
                          }
                          frame 3 {
                            n923 = property on="Colors for Stim. setup" class="Arr (strict)"() -> ("Value"=w1681:T3)  [unwired: 2 in, 2 out]
                            n924 = Select(t=w1681, s=w1682, f=T11 [{"Numeric Control"=12369084, "Numeric Control"=12369084}, {"Numeric Control"=6603023, "Numeric Control"=6603023}, {"Numeric Control"=1976113, "Numeric Control"=1976113}, {"Numeric Control"=2575993, "Numeric Control"=2575993}] ("Colors [4] 2")) -> (s? t:f=w1684:T11)
                            n925 = property on="Zone 03" class="Bool (strict)"("Colors [4]"=w1684) -> ()  [unwired: 2 in, 2 out]
                          }
                          frame 4 {
                            n926 = property on="Colors for Stim. setup" class="Arr (strict)"() -> ("Value"=w1685:T3)  [unwired: 2 in, 2 out]
                            n927 = Select(t=w1685, s=w1686, f=T11 [{"Numeric Control"=12369084, "Numeric Control"=12369084}, {"Numeric Control"=6603023, "Numeric Control"=6603023}, {"Numeric Control"=1976113, "Numeric Control"=1976113}, {"Numeric Control"=2575993, "Numeric Control"=2575993}] ("Colors [4] 2")) -> (s? t:f=w1688:T11)
                            n928 = property on="Zone 04" class="Bool (strict)"("Colors [4]"=w1688) -> ()  [unwired: 2 in, 2 out]
                          }
                          frame 5 {
                            n929 = property on="Colors for Stim. setup" class="Arr (strict)"() -> ("Value"=w1689:T3)  [unwired: 2 in, 2 out]
                            n930 = Select(t=w1689, s=w1690, f=T11 [{"Numeric Control"=12369084, "Numeric Control"=12369084}, {"Numeric Control"=6603023, "Numeric Control"=6603023}, {"Numeric Control"=1976113, "Numeric Control"=1976113}, {"Numeric Control"=2575993, "Numeric Control"=2575993}] ("Colors [4] 2")) -> (s? t:f=w1692:T11)
                            n931 = property on="Zone 05" class="Bool (strict)"("Colors [4]"=w1692) -> ()  [unwired: 2 in, 2 out]
                          }
                          frame 6 {
                            n932 = property on="Colors for Stim. setup" class="Arr (strict)"() -> ("Value"=w1693:T3)  [unwired: 2 in, 2 out]
                            n933 = Select(t=w1693, s=w1694, f=T11 [{"Numeric Control"=12369084, "Numeric Control"=12369084}, {"Numeric Control"=6603023, "Numeric Control"=6603023}, {"Numeric Control"=1976113, "Numeric Control"=1976113}, {"Numeric Control"=2575993, "Numeric Control"=2575993}] ("Colors [4] 2")) -> (s? t:f=w1696:T11)
                            n934 = property on="Zone 06" class="Bool (strict)"("Colors [4]"=w1696) -> ()  [unwired: 2 in, 2 out]
                          }
                          frame 7 {
                            n935 = property on="Colors for Stim. setup" class="Arr (strict)"() -> ("Value"=w1697:T3)  [unwired: 2 in, 2 out]
                            n936 = Select(t=w1697, s=w1698, f=T11 [{"Numeric Control"=12369084, "Numeric Control"=12369084}, {"Numeric Control"=6603023, "Numeric Control"=6603023}, {"Numeric Control"=1976113, "Numeric Control"=1976113}, {"Numeric Control"=2575993, "Numeric Control"=2575993}] ("Colors [4] 2")) -> (s? t:f=w1700:T11)
                            n937 = property on="Zone 07" class="Bool (strict)"("Colors [4]"=w1700) -> ()  [unwired: 2 in, 2 out]
                          }
                          frame 8 {
                            n938 = property on="Colors for Stim. setup" class="Arr (strict)"() -> ("Value"=w1701:T3)  [unwired: 2 in, 2 out]
                            n939 = Select(t=w1701, s=w1702, f=T11 [{"Numeric Control"=12369084, "Numeric Control"=12369084}, {"Numeric Control"=6603023, "Numeric Control"=6603023}, {"Numeric Control"=1976113, "Numeric Control"=1976113}, {"Numeric Control"=2575993, "Numeric Control"=2575993}] ("Colors [4] 2")) -> (s? t:f=w1704:T11)
                            n940 = property on="Zone 08" class="Bool (strict)"("Colors [4]"=w1704) -> ()  [unwired: 2 in, 2 out]
                          }
                          frame 9 {
                            n941 = property on="Colors for Stim. setup" class="Arr (strict)"() -> ("Value"=w1705:T3)  [unwired: 2 in, 2 out]
                            n942 = Select(t=w1705, s=w1706, f=T11 [{"Numeric Control"=12369084, "Numeric Control"=12369084}, {"Numeric Control"=6603023, "Numeric Control"=6603023}, {"Numeric Control"=1976113, "Numeric Control"=1976113}, {"Numeric Control"=2575993, "Numeric Control"=2575993}] ("Colors [4] 2")) -> (s? t:f=w1708:T11)
                            n943 = property on="Zone 09" class="Bool (strict)"("Colors [4]"=w1708) -> ()  [unwired: 2 in, 2 out]
                          }
                          frame 10 {
                            n944 = property on="Colors for Stim. setup" class="Arr (strict)"() -> ("Value"=w1709:T3)  [unwired: 2 in, 2 out]
                            n945 = Select(t=w1709, s=w1710, f=T11 [{"Numeric Control"=12369084, "Numeric Control"=12369084}, {"Numeric Control"=6603023, "Numeric Control"=6603023}, {"Numeric Control"=1976113, "Numeric Control"=1976113}, {"Numeric Control"=2575993, "Numeric Control"=2575993}] ("Colors [4] 2")) -> (s? t:f=w1712:T11)
                            n946 = property on="Zone 10" class="Bool (strict)"("Colors [4]"=w1712) -> ()  [unwired: 2 in, 2 out]
                          }
                          frame 11 {
                            n947 = property on="Colors for Stim. setup" class="Arr (strict)"() -> ("Value"=w1713:T3)  [unwired: 2 in, 2 out]
                            n948 = Select(t=w1713, s=w1714, f=T11 [{"Numeric Control"=12369084, "Numeric Control"=12369084}, {"Numeric Control"=6603023, "Numeric Control"=6603023}, {"Numeric Control"=1976113, "Numeric Control"=1976113}, {"Numeric Control"=2575993, "Numeric Control"=2575993}] ("Colors [4] 2")) -> (s? t:f=w1716:T11)
                            n949 = property on="Zone 11" class="Bool (strict)"("Colors [4]"=w1716) -> ()  [unwired: 2 in, 2 out]
                          }
                          frame 12 {
                            n950 = property on="Colors for Stim. setup" class="Arr (strict)"() -> ("Value"=w1717:T3)  [unwired: 2 in, 2 out]
                            n951 = Select(t=w1717, s=w1718, f=T11 [{"Numeric Control"=12369084, "Numeric Control"=12369084}, {"Numeric Control"=6603023, "Numeric Control"=6603023}, {"Numeric Control"=1976113, "Numeric Control"=1976113}, {"Numeric Control"=2575993, "Numeric Control"=2575993}] ("Colors [4] 2")) -> (s? t:f=w1720:T11)
                            n952 = property on="Zone 12" class="Bool (strict)"("Colors [4]"=w1720) -> ()  [unwired: 2 in, 2 out]
                          }
                          frame 13 {
                            n953 = property on="Colors for Stim. setup" class="Arr (strict)"() -> ("Value"=w1721:T3)  [unwired: 2 in, 2 out]
                            n954 = Select(t=w1721, s=w1722, f=T11 [{"Numeric Control"=12369084, "Numeric Control"=12369084}, {"Numeric Control"=6603023, "Numeric Control"=6603023}, {"Numeric Control"=1976113, "Numeric Control"=1976113}, {"Numeric Control"=2575993, "Numeric Control"=2575993}] ("Colors [4] 2")) -> (s? t:f=w1724:T11)
                            n955 = property on="Zone 13" class="Bool (strict)"("Colors [4]"=w1724) -> ()  [unwired: 2 in, 2 out]
                          }
                        }
                      }
                      frame Enabled {
                      }
                    }
                    n956 = property on="Stimulus presets" class="Arr (strict)"() -> ("Index Values"=w1662:u32[])  [unwired: 2 in, 2 out]
                    n957 = Index Array(array=w1662, index=0) -> (element=w1648:u32)
                    n958 = Index Array(array=w1647, index=w1648) -> (element=w1656:T50)
                    n959 = property on="Zone-based stimulus setup" class="RadioBtnsControl (strict)"() -> ("Value"=w1660:T8)  [unwired: 2 in, 2 out]
                    n960 = Unbundle By Name(w1656) -> ("Set/Clear"=w1657:bool, "Time, s"=w1652:sgl, "Stimulus, s"=w1650:sgl)
                    n961 = Format Into String(w1660) -> ()  [unwired: 3 in, 2 out]
                    n962 = Greater Than 0?(x=w1652) -> (x > 0?=w1659:bool)
                    n963 = Greater Than 0?(x=w1650) -> (x > 0?=w1658:bool)
                    n964 = expression code="floor(x * 100) / 100"(w1652) -> (w1651:sgl)
                    n965 = expression code="floor(x * 100) / 100"(w1650) -> (w1649:sgl)
                    n966 = To Unsigned Byte Integer(number=w1660) -> (unsigned 8bit integer=w1645:u8)
                    n967 = Compound Arithmetic op=AND(w1657, w1659, w1658) -> (w1646:bool)
                    n968 = Greater Than 0?(x=w1645) -> (x > 0?=w1644:bool)
                    n969 = Bundle By Name(cluster=w1656, "Stim. has been set"=w1646, "Set/Clear"=w1646, "Time, s"=w1651, "Stimulus, s"=w1649) -> (w1655:T50)
                    n970 = case shown="True" w1644 {
                      tunnel: w1646 -> [_ w1666]
                      tunnel: w1645 -> [_ w1665]
                      frame False {
                      }
                      frame True {
                        w1670 = refnum<vi> refnum  # Boolean
                        n971 = property on="Colors for Stim. setup" class="Arr (strict)"() -> ("Value"=w1667:T3)  [unwired: 2 in, 2 out]
                        n972 = Decrement(x=w1665) -> (x-1=w1664:u8)
                        n973 = Select(t=w1667, s=w1666, f=T11 [{"Numeric Control"=12369084, "Numeric Control"=12369084}, {"Numeric Control"=6603023, "Numeric Control"=6603023}, {"Numeric Control"=1976113, "Numeric Control"=1976113}, {"Numeric Control"=2575993, "Numeric Control"=2575993}] ("Colors [4] 2")) -> (s? t:f=w1672:T11)
                        n974 = property on="Zone-based stimulus setup" class="RadioBtnsControl (strict)"() -> ("Controls[]"=w1663:refnum<vi>[])  [unwired: 2 in, 2 out]
                        n975 = Index Array(array=w1663, index=w1664) -> (element=w1669:refnum<vi>)
                        n976 = To More Specific Class(target class=w1670, reference=w1669) -> (specific class reference=w1671:refnum<vi>)  [unwired: 1 in, 1 out]
                        n977 = property class="Bool"(reference=w1671, "Colors [4]"=w1672) -> ()  [unwired: 1 in, 2 out]
                      }
                    }
                    n978 = Replace Array Subset(array=w1647, new element=w1655, index=w1648) -> (w1653:T7)
                    n979 = global write "SW_Globals.vi" "Zone-based stimulus presets"(w1653) -> ()
                    n980 = property on="Stimulus presets" class="Arr (strict)"("Value"=w1653) -> ()  [unwired: 2 in, 2 out]
                    n981 = for {
                      tunnel: w1653 -> [w1728] mode=indexing
                      tunnel: [w1725] -> w1654 mode=indexing if=w1726
                      i -> [w1727]
                      n982 = Unbundle By Name(w1728) -> ("Stim. has been set"=w1726:bool)
                      n983 = To Unsigned Byte Integer(number=w1727) -> (unsigned 8bit integer=w1725:u8)
                    }
                    n984 = global write "SW_Globals.vi" "Regions to track"(w1654) -> ()
                  }
                  event "Reset stimuli", "Changed IO": Value Change {
                    n985 = event-data() -> ("OldVal"=w1730:bool, "NewVal"=w1731:bool)  [unwired: 1 in, 4 out]
                    n986 = property on="Reset stimuli" class="Bool (strict)"("Value"=w1730) -> ()  [unwired: 2 in, 2 out]
                    n987 = property on="Changed IO" class="Bool (strict)"("Value"=FALSE ("Changed IO")) -> ()  [unwired: 2 in, 2 out]
                    n988 = case shown="True" w1731 {
                      selector: w1731 -> [_ w1755]
                      frame False {
                      }
                      frame True {
                        w1743 = T11 [{"Numeric Control"=9868950, "Numeric Control"=15790320}, {"Numeric Control"=8388608, "Numeric Control"=8388608}, {"Numeric Control"=4934475, "Numeric Control"=7895160}, {"Numeric Control"=994319, "Numeric Control"=1657881}]  # TTL IO In colors
                        w1744 = T11 [{"Numeric Control"=9868950, "Numeric Control"=15790320}, {"Numeric Control"=1988894, "Numeric Control"=3381555}, {"Numeric Control"=4934475, "Numeric Control"=7895160}, {"Numeric Control"=994319, "Numeric Control"=1657881}]  # TTL IO Out colors
                        n989 = global write "SW_Globals.vi" "Regions to track"(u8[] []) -> ()
                        n990 = global read "SW_Globals.vi" "IO ports config"() -> (w1742:bool[])
                        n991 = Index Array(array=w1742, index=1) -> (element=w1747:bool)
                        n992 = Index Array(array=w1742, index=2) -> (element=w1746:bool)
                        n993 = Index Array(array=w1742, index=3) -> (element=w1745:bool)
                        n994 = Index Array(array=w1742, index=0) -> (element=w1748:bool)
                        n995 = Select(t=w1743, s=w1747, f=w1744) -> (s? t:f=w1740:T11)
                        n996 = Select(t=w1743, s=w1746, f=w1744) -> (s? t:f=w1739:T11)
                        n997 = Select(t=w1743, s=w1745, f=w1744) -> (s? t:f=w1738:T11)
                        n998 = Select(t=w1743, s=w1748, f=w1744) -> (s? t:f=w1741:T11)
                        n999 = property on="TTL IO 2 (analysis)" class="Bool"("Colors [4]"=w1740) -> ()  [unwired: 2 in, 2 out]
                        n1000 = property on="TTL IO 2 (recording)" class="Bool (strict)"("Colors [4]"=w1740) -> ()  [unwired: 2 in, 2 out]
                        n1001 = property on="TTL IO 3 (analysis)" class="Bool"("Colors [4]"=w1739) -> ()  [unwired: 2 in, 2 out]
                        n1002 = property on="TTL IO 3 (recording)" class="Bool (strict)"("Colors [4]"=w1739) -> ()  [unwired: 2 in, 2 out]
                        n1003 = property on="TTL IO 4 (analysis)" class="Bool"("Colors [4]"=w1738) -> ()  [unwired: 2 in, 2 out]
                        n1004 = property on="TTL IO 4 (recording)" class="Bool (strict)"("Colors [4]"=w1738) -> ()  [unwired: 2 in, 2 out]
                        n1005 = property on="TTL IO 1 (analysis)" class="Bool"("Colors [4]"=w1741) -> ()  [unwired: 2 in, 2 out]
                        n1006 = property on="TTL IO 1 (recording)" class="Bool (strict)"("Colors [4]"=w1741) -> ()  [unwired: 2 in, 2 out]
                        n1007 = global read "SW_Globals.vi" "IO parameters cluster"() -> (w1754:T2)
                        n1008 = Unbundle By Name(w1754) -> ("SYNC configuration"=w1753:u16, "IO 1 configuration"=w1733:u16, "IO 2 configuration"=w1732:u16)
                        n1009 = call "SW_Gen_Available_TTL_outputs_array.vi"("IO 2 configuration"=w1732, "IO 1 configuration"=w1733, "SYNC configuration"=w1753) -> ("Available TTL outputs array"=w1737:cluster{"String":string, "Value":i32}[])
                        n1010 = property on="TTL out" class="Ring (strict)"("StringsAndValues[]"=w1737) -> ()  [unwired: 2 in, 2 out]
                        n1011 = disable-structure shown="Disabled" {
                          frame Disabled {
                            n1012 = case shown="6" {
                              selector: _ -> [_ _ _ _ _ _ _ _ _ _ _ _ _ _]
                              frame 0, Default {
                              }
                              frame 1 {
                                n1013 = property on="Zone 01" class="Bool (strict)"("Colors [4]"=T11 [{"Numeric Control"=12369084, "Numeric Control"=12369084}, {"Numeric Control"=6603023, "Numeric Control"=6603023}, {"Numeric Control"=1976113, "Numeric Control"=1976113}, {"Numeric Control"=2575993, "Numeric Control"=2575993}] ("Colors [4] 2"), "Value"=FALSE) -> ()  [unwired: 2 in, 2 out]
                              }
                              frame 2 {
                                n1014 = property on="Zone 02" class="Bool (strict)"("Colors [4]"=T11 [{"Numeric Control"=12369084, "Numeric Control"=12369084}, {"Numeric Control"=6603023, "Numeric Control"=6603023}, {"Numeric Control"=1976113, "Numeric Control"=1976113}, {"Numeric Control"=2575993, "Numeric Control"=2575993}] ("Colors [4] 2"), "Value"=FALSE) -> ()  [unwired: 2 in, 2 out]
                              }
                              frame 3 {
                                n1015 = property on="Zone 03" class="Bool (strict)"("Colors [4]"=T11 [{"Numeric Control"=12369084, "Numeric Control"=12369084}, {"Numeric Control"=6603023, "Numeric Control"=6603023}, {"Numeric Control"=1976113, "Numeric Control"=1976113}, {"Numeric Control"=2575993, "Numeric Control"=2575993}] ("Colors [4] 2"), "Value"=FALSE) -> ()  [unwired: 2 in, 2 out]
                              }
                              frame 4 {
                                n1016 = property on="Zone 04" class="Bool (strict)"("Colors [4]"=T11 [{"Numeric Control"=12369084, "Numeric Control"=12369084}, {"Numeric Control"=6603023, "Numeric Control"=6603023}, {"Numeric Control"=1976113, "Numeric Control"=1976113}, {"Numeric Control"=2575993, "Numeric Control"=2575993}] ("Colors [4] 2"), "Value"=FALSE) -> ()  [unwired: 2 in, 2 out]
                              }
                              frame 5 {
                                n1017 = property on="Zone 05" class="Bool (strict)"("Colors [4]"=T11 [{"Numeric Control"=12369084, "Numeric Control"=12369084}, {"Numeric Control"=6603023, "Numeric Control"=6603023}, {"Numeric Control"=1976113, "Numeric Control"=1976113}, {"Numeric Control"=2575993, "Numeric Control"=2575993}] ("Colors [4] 2"), "Value"=FALSE) -> ()  [unwired: 2 in, 2 out]
                              }
                              frame 6 {
                                n1018 = property on="Zone 06" class="Bool (strict)"("Colors [4]"=T11 [{"Numeric Control"=12369084, "Numeric Control"=12369084}, {"Numeric Control"=6603023, "Numeric Control"=6603023}, {"Numeric Control"=1976113, "Numeric Control"=1976113}, {"Numeric Control"=2575993, "Numeric Control"=2575993}] ("Colors [4] 2"), "Value"=FALSE) -> ()  [unwired: 2 in, 2 out]
                              }
                              frame 7 {
                                n1019 = property on="Zone 07" class="Bool (strict)"("Colors [4]"=T11 [{"Numeric Control"=12369084, "Numeric Control"=12369084}, {"Numeric Control"=6603023, "Numeric Control"=6603023}, {"Numeric Control"=1976113, "Numeric Control"=1976113}, {"Numeric Control"=2575993, "Numeric Control"=2575993}] ("Colors [4] 2"), "Value"=FALSE) -> ()  [unwired: 2 in, 2 out]
                              }
                              frame 8 {
                                n1020 = property on="Zone 08" class="Bool (strict)"("Colors [4]"=T11 [{"Numeric Control"=12369084, "Numeric Control"=12369084}, {"Numeric Control"=6603023, "Numeric Control"=6603023}, {"Numeric Control"=1976113, "Numeric Control"=1976113}, {"Numeric Control"=2575993, "Numeric Control"=2575993}] ("Colors [4] 2"), "Value"=FALSE) -> ()  [unwired: 2 in, 2 out]
                              }
                              frame 9 {
                                n1021 = property on="Zone 09" class="Bool (strict)"("Colors [4]"=T11 [{"Numeric Control"=12369084, "Numeric Control"=12369084}, {"Numeric Control"=6603023, "Numeric Control"=6603023}, {"Numeric Control"=1976113, "Numeric Control"=1976113}, {"Numeric Control"=2575993, "Numeric Control"=2575993}] ("Colors [4] 2"), "Value"=FALSE) -> ()  [unwired: 2 in, 2 out]
                              }
                              frame 10 {
                                n1022 = property on="Zone 10" class="Bool (strict)"("Colors [4]"=T11 [{"Numeric Control"=12369084, "Numeric Control"=12369084}, {"Numeric Control"=6603023, "Numeric Control"=6603023}, {"Numeric Control"=1976113, "Numeric Control"=1976113}, {"Numeric Control"=2575993, "Numeric Control"=2575993}] ("Colors [4] 2"), "Value"=FALSE) -> ()  [unwired: 2 in, 2 out]
                              }
                              frame 11 {
                                n1023 = property on="Zone 11" class="Bool (strict)"("Colors [4]"=T11 [{"Numeric Control"=12369084, "Numeric Control"=12369084}, {"Numeric Control"=6603023, "Numeric Control"=6603023}, {"Numeric Control"=1976113, "Numeric Control"=1976113}, {"Numeric Control"=2575993, "Numeric Control"=2575993}] ("Colors [4] 2"), "Value"=FALSE) -> ()  [unwired: 2 in, 2 out]
                              }
                              frame 12 {
                                n1024 = property on="Zone 12" class="Bool (strict)"("Colors [4]"=T11 [{"Numeric Control"=12369084, "Numeric Control"=12369084}, {"Numeric Control"=6603023, "Numeric Control"=6603023}, {"Numeric Control"=1976113, "Numeric Control"=1976113}, {"Numeric Control"=2575993, "Numeric Control"=2575993}] ("Colors [4] 2"), "Value"=FALSE) -> ()  [unwired: 2 in, 2 out]
                              }
                              frame 13 {
                                n1025 = property on="Zone 13" class="Bool (strict)"("Colors [4]"=T11 [{"Numeric Control"=12369084, "Numeric Control"=12369084}, {"Numeric Control"=6603023, "Numeric Control"=6603023}, {"Numeric Control"=1976113, "Numeric Control"=1976113}, {"Numeric Control"=2575993, "Numeric Control"=2575993}] ("Colors [4] 2"), "Value"=FALSE) -> ()  [unwired: 2 in, 2 out]
                              }
                            }
                          }
                          frame Enabled {
                          }
                        }
                        n1026 = Index Array(array=w1737, index=0) -> (element=w1735:cluster{"String":string, "Value":i32})
                        n1027 = Unbundle By Name(w1735) -> ("Value"=w1734:i32)
                        n1028 = for {
                          N: 14 -> [_]
                          tunnel: [w1792] -> w1760 mode=indexing
                          tunnel: [w1789] -> w1756
                          tunnel: w1755 -> [w1789]
                          tunnel: w1734 -> [w1790]
                          i -> [w1788]
                          n1029 = Greater Than 0?(x=w1788) -> (x > 0?=w1787:bool)
                          n1030 = case shown="True" w1787 {
                            tunnel: w1788 -> [_ w1796]
                            frame False {
                            }
                            frame True {
                              w1799 = refnum<vi> refnum  # Boolean
                              n1031 = Decrement(x=w1796) -> (x-1=w1795:i32)
                              n1032 = property on="Zone-based stimulus setup" class="RadioBtnsControl (strict)"() -> ("Controls[]"=w1797:refnum<vi>[])  [unwired: 2 in, 2 out]
                              n1033 = Index Array(array=w1797, index=w1795) -> (element=w1798:refnum<vi>)
                              n1034 = To More Specific Class(target class=w1799, reference=w1798) -> (specific class reference=w1800:refnum<vi>)  [unwired: 1 in, 1 out]
                              n1035 = property class="Bool"(reference=w1800, "Colors [4]"=T11 [{"Numeric Control"=12369084, "Numeric Control"=12369084}, {"Numeric Control"=6603023, "Numeric Control"=6603023}, {"Numeric Control"=1976113, "Numeric Control"=1976113}, {"Numeric Control"=2575993, "Numeric Control"=2575993}] ("Colors [4] 2"), "Value"=FALSE) -> ()  [unwired: 1 in, 2 out]
                            }
                          }
                          n1036 = Bundle By Name(cluster=T45 {"Event type"=0, "Cond., s"=0.0, "Stim., s"=0.0, "Set/Clear"=FALSE, "TTL out N"=1, "Stim. has been set"=FALSE} ("Cluster of the stimuls settings"), "TTL out N"=w1790) -> (w1792:T45)
                        }
                        n1037 = global write "SW_Globals.vi" "Zone-based stimulus presets"(w1760) -> ()
                        n1038 = property on="Stimulus presets" class="Arr (strict)"("Value"=w1760) -> (error out=w1757:errorcluster)  [unwired: 2 in, 1 out]
                        n1039 = property on="Reset STIM" class="Bool (strict)"(error in=w1757, "Val(Sgnl)"=w1756) -> ()  [unwired: 1 in, 2 out]
                      }
                    }
                  }
                  event "Reset regions": Value Change {
                    n1040 = event-data() -> ("OldVal"=w1801:bool, "NewVal"=w1802:bool)  [unwired: 1 in, 4 out]
                    n1041 = property on="Reset regions" class="Bool (strict)"("Value"=w1801) -> ()  [unwired: 2 in, 2 out]
                    n1042 = case shown="True" w1802 {
                      selector: w1802 -> [_ w1804]
                      frame False {
                      }
                      frame True {
                        n1043 = local read "Cage diameter, mm"() -> (w1805:u16)
                        n1044 = case shown="240" w1805 {
                          tunnel: w1804 -> [w1806 w1813 w1820 w1827 w1834 w1841]
                          tunnel: [w1806 w1813 w1820 w1827 w1834 w1841] -> w1803
                          frame 180, Default {
                            n1045 = local write "Starting angle BORDER"(i16 0 ("Starting angle")) -> ()
                            n1046 = local write "N segments BORDER"(u8 4 ("N segments")) -> ()
                            n1047 = local write "N segments MIDFIELD"(u8 2 ("N segments")) -> ()
                            n1048 = local write "Starting angle MIDFIELD"(i16 0 ("Starting angle")) -> ()
                            n1049 = local write "Radius, mm CENTER"(u16 30 ("Radius, mm")) -> ()
                            n1050 = local write "Radius, mm MIDFIELD"(u16 75 ("Radius, mm")) -> ()
                          }
                          frame 240 {
                            n1051 = local write "Starting angle BORDER"(i16 0 ("Starting angle")) -> ()
                            n1052 = local write "N segments BORDER"(u8 4 ("N segments")) -> ()
                            n1053 = local write "N segments MIDFIELD"(u8 2 ("N segments")) -> ()
                            n1054 = local write "Starting angle MIDFIELD"(i16 0 ("Starting angle")) -> ()
                            n1055 = local write "Radius, mm CENTER"(u16 32 ("Radius, mm")) -> ()
                            n1056 = local write "Radius, mm MIDFIELD"(u16 75 ("Radius, mm")) -> ()
                          }
                          frame 290 {
                            n1057 = local write "Starting angle BORDER"(i16 0 ("Starting angle")) -> ()
                            n1058 = local write "N segments BORDER"(u8 4 ("N segments")) -> ()
                            n1059 = local write "N segments MIDFIELD"(u8 2 ("N segments")) -> ()
                            n1060 = local write "Starting angle MIDFIELD"(i16 0 ("Starting angle")) -> ()
                            n1061 = local write "Radius, mm CENTER"(u16 48 ("Radius, mm")) -> ()
                            n1062 = local write "Radius, mm MIDFIELD"(u16 121 ("Radius, mm")) -> ()
                          }
                          frame 325 {
                            n1063 = local write "Starting angle BORDER"(i16 0 ("Starting angle")) -> ()
                            n1064 = local write "N segments BORDER"(u8 4 ("N segments")) -> ()
                            n1065 = local write "N segments MIDFIELD"(u8 2 ("N segments")) -> ()
                            n1066 = local write "Starting angle MIDFIELD"(i16 0 ("Starting angle")) -> ()
                            n1067 = local write "Radius, mm CENTER"(u16 50 ("Radius, mm")) -> ()
                            n1068 = local write "Radius, mm MIDFIELD"(u16 148 ("Radius, mm")) -> ()
                          }
                          frame 327 {
                            n1069 = local write "Starting angle BORDER"(i16 0 ("Starting angle")) -> ()
                            n1070 = local write "N segments BORDER"(u8 4 ("N segments")) -> ()
                            n1071 = local write "N segments MIDFIELD"(u8 2 ("N segments")) -> ()
                            n1072 = local write "Starting angle MIDFIELD"(i16 0 ("Starting angle")) -> ()
                            n1073 = local write "Radius, mm CENTER"(u16 50 ("Radius, mm")) -> ()
                            n1074 = local write "Radius, mm MIDFIELD"(u16 150 ("Radius, mm")) -> ()
                          }
                          frame 333 {
                            n1075 = local write "Starting angle BORDER"(i16 0 ("Starting angle")) -> ()
                            n1076 = local write "N segments BORDER"(u8 4 ("N segments")) -> ()
                            n1077 = local write "N segments MIDFIELD"(u8 2 ("N segments")) -> ()
                            n1078 = local write "Starting angle MIDFIELD"(i16 0 ("Starting angle")) -> ()
                            n1079 = local write "Radius, mm CENTER"(u16 50 ("Radius, mm")) -> ()
                            n1080 = local write "Radius, mm MIDFIELD"(u16 152 ("Radius, mm")) -> ()
                          }
                        }
                        n1081 = property on="Reset REG" class="Bool (strict)"("Val(Sgnl)"=w1803) -> ()  [unwired: 2 in, 2 out]
                      }
                    }
                  }
                  event "Set advanced stimulus": Value Change {
                    n1082 = event-data() -> ("OldVal"=w1849:bool)  [unwired: 1 in, 5 out]
                    n1083 = property on="Set advanced stimulus" class="Bool (strict)"("Value"=w1849) -> (error out=w1851:errorcluster)  [unwired: 2 in, 1 out]
                    n1084 = property on="Adv. Stim. set" class="Bool (strict)"(error in=w1851, "Value"=w1849) -> (error out=w1850:errorcluster)  [unwired: 1 in, 1 out]
                    n1085 = flat-sequence {
                      tunnel: w1850 -> [_]
                      tunnel: [w1852] -> w1848
                      tunnel: w1848 -> [w1867]
                      frame #0 {
                        n1086 = property on="Stimulus presets" class="Arr (strict)"() -> ("Value"=w1853:T7)  [unwired: 2 in, 2 out]
                        n1087 = local read "N segments MIDFIELD"() -> (w1864:u8)
                        n1088 = local read "N segments BORDER"() -> (w1865:u8)
                        n1089 = global read "SW_Globals.vi" "Speed detection threshold, mm/s"() -> (w1858:dbl)
                        n1090 = global read "SW_Globals.vi" "Run time threshold, s"() -> (w1859:dbl)
                        n1091 = global read "SW_Globals.vi" "Run time pause, s"() -> (w1860:dbl)
                        n1092 = Compound Arithmetic op=ADD(w1865, w1864, u8 1 ("value")) -> (w1862:u8)
                        n1093 = global read "SW_Globals.vi" "Run time stim, s"() -> (w1861:dbl)
                        n1094 = call "SW_Set_Adv_Stimulus_interface.vi"("Zone-based stimulus presents"=w1853, "Total amount of segments"=w1862, "Run time stim, s"=w1861, "Run time pause, s"=w1860, "Run time threshold, s"=w1859, "Speed detection threshold, mm/s"=w1858) -> ("Modified Zone-based stimulus presents"=w1852:T7, "Out Run time stim, s"=w1857:dbl, "Out Run time pause, s"=w1856:dbl, "Out Run time threshold, s"=w1855:dbl, "Out Speed detection threshold, mm/s"=w1854:dbl)  [unwired: 4 in, 1 out]
                        n1095 = property on="Stimulus presets" class="Arr (strict)"("Value"=w1852) -> ()  [unwired: 2 in, 2 out]
                        n1096 = global write "SW_Globals.vi" "Speed detection threshold, mm/s"(w1854) -> ()
                        n1097 = global write "SW_Globals.vi" "Run time stim, s"(w1857) -> ()
                        n1098 = global write "SW_Globals.vi" "Run time pause, s"(w1856) -> ()
                        n1099 = global write "SW_Globals.vi" "Run time threshold, s"(w1855) -> ()
                      }
                      frame #1 {
                        n1100 = for {
                          tunnel: [w1872] -> w1866 mode=indexing if=w1870
                          tunnel: w1867 -> [w1871] mode=indexing
                          i -> [w1869]
                          n1101 = Unbundle By Name(w1871) -> ("Stim. has been set"=w1870:bool)
                          n1102 = Greater Than 0?(x=w1869) -> (x > 0?=w1868:bool)
                          n1103 = case shown="True" w1868 {
                            tunnel: w1870 -> [_ w1883]
                            tunnel: w1869 -> [_ w1874]
                            frame False {
                            }
                            frame True {
                              w1878 = refnum<vi> refnum  # Boolean
                              n1104 = Decrement(x=w1874) -> (x-1=w1873:i32)
                              n1105 = property on="Colors for Stim. setup" class="Arr (strict)"() -> ("Value"=w1882:T3)  [unwired: 2 in, 2 out]
                              n1106 = Select(t=w1882, s=w1883, f=T11 [{"Numeric Control"=12369084, "Numeric Control"=12369084}, {"Numeric Control"=6603023, "Numeric Control"=6603023}, {"Numeric Control"=1976113, "Numeric Control"=1976113}, {"Numeric Control"=2575993, "Numeric Control"=2575993}] ("Colors [4] 2")) -> (s? t:f=w1876:T11)
                              n1107 = property on="Zone-based stimulus setup" class="RadioBtnsControl (strict)"() -> ("Controls[]"=w1880:refnum<vi>[])  [unwired: 2 in, 2 out]
                              n1108 = Index Array(array=w1880, index=w1873) -> (element=w1879:refnum<vi>)
                              n1109 = To More Specific Class(target class=w1878, reference=w1879) -> (specific class reference=w1877:refnum<vi>)  [unwired: 1 in, 1 out]
                              n1110 = property class="Bool"(reference=w1877, "Colors [4]"=w1876, "Value"=FALSE) -> ()  [unwired: 1 in, 2 out]
                            }
                          }
                          n1111 = To Unsigned Byte Integer(number=w1869) -> (unsigned 8bit integer=w1872:u8)
                        }
                        n1112 = global write "SW_Globals.vi" "Regions to track"(w1866) -> ()
                      }
                      frame #2 {
                        n1113 = property on="Adv. Stim. set" class="Bool (strict)"("Val(Sgnl)"=TRUE ("Value (Signaling)")) -> ()  [unwired: 2 in, 2 out]
                      }
                    }
                  }
                  event "Load settings": Value Change {
                    (unwired) "*.trset; *.tdms" ("default name")
                    w1898 = T51 2 items=["User Home"=0, "User Desktop"=1, "User Documents"=2, "User Application Data"=3, "User Preferences"=4, "User Temporary"=5, "Public Documents"=6, "Public Application Data"=7, "Public Preferences"=8, "Public Cache"=13, "System Core Libraries"=9, "System Installed Libraries"=10, "Application Files"=11, "Boot Volume Root"=12] ("system directory type")
                    n1114 = event-data() -> ("OldVal"=w1903:bool)  [unwired: 1 in, 5 out]
                    n1115 = property on="Load settings" class="Bool (strict)"("Value"=w1903) -> ()  [unwired: 2 in, 2 out]
                    n1116 = call <vilib>:"Get System Directory.vi"("system directory type"=w1898) -> ("system directory"=w1894:path)  [unwired: 10 in]
                    n1117 = Build Path(base path=w1894, name or relative path="MHC_Tracker" ("string")) -> (appended path=w1895:path)
                    n1118 = call <vilib>:"Check if File or Folder Exists.vi"("path"=w1895) -> ("file or folder exists?"=w1896:bool)  [unwired: 8 in, 2 out]
                    n1119 = Select(t=w1895, s=w1896, f=w1894) -> (s? t:f=w1893:path)
                    n1120 = call "Load Settings"("start path"=w1893, "prompt"="Please choose file to load settings from", "button label"="Load", "pattern (all files)"="*.trset; *.tdms" ("default name"), "pattern label"="Settings or track") -> ("selected path"=w1888:path, "exists"=w1890:bool, "cancelled"=w1891:bool, "error out"=w1887:errorcluster)  [unwired: 7 in]
                    n1121 = Not(x=w1891) -> (.not. x?=w1892:bool)
                    n1122 = And(x=w1890, y=w1892) -> (x .and. y?=w1889:bool)
                    n1123 = case shown="True" w1889 {
                      tunnel: w1888 -> [_ w1928]
                      tunnel: w1887 -> [w1904 w1929]
                      tunnel: [w1904 w1907] -> w1886
                      tunnel: [FALSE ("IO paramaters loaded") TRUE ("IO paramaters loaded")] -> w1885
                      frame False {
                      }
                      frame True {
                        n1124 = local read "Current User"() -> (w1930:string)
                        n1125 = call "SW_Load_settings_from_previous_experiments.vi"("File to load data from"=w1928, "User Name"=w1930, "error in (no error)"=w1929) -> ("Settings cluster out"=w1927:T35, "IO parameters cluster"=→"IO parameters loaded cluster":T2, "Stimulus presets array"=w1909:T36, "error out"=w1907:errorcluster)  [unwired: 4 in]
                        n1126 = Unbundle By Name(w1927) -> ("Name prefix"=w1926:string, "N segments MIDFIELD"=w1913:u8, "N segments BORDER"=w1925:u8, "Radius, mm CENTER"=w1924:u16, "Radius, mm MIDFIELD"=w1923:u16, "Starting angle MIDFIELD"=w1922:i16, "Starting angle BORDER"=w1921:i16, "Cage diameter, mm"=w1920:u16, "Bridge swap"=w1919:bool, "Bridge V. offset"=w1918:sgl, "Twisted neck"=w1916:bool, "Offset H."=w1917:sgl, "\"Stop at\" enabled"=w1915:bool, "Stop at"=w1914:dbl, "Data filtering"=w1908:u16)
                        n1127 = local write "N segments BORDER"(w1925) -> ()
                        n1128 = local write "Radius, mm CENTER"(w1924) -> ()
                        n1129 = local write "Radius, mm MIDFIELD"(w1923) -> ()
                        n1130 = local write "Starting angle MIDFIELD"(w1922) -> ()
                        n1131 = local write "Starting angle BORDER"(w1921) -> ()
                        n1132 = local write "Cage diameter, mm"(w1920) -> ()
                        n1133 = property on="Bridge swap" class="Bool (strict)"("Value"=w1919) -> ()  [unwired: 2 in, 2 out]
                        n1134 = local write "Bridge offset"(w1918) -> ()
                        n1135 = local write "Twisted neck"(w1916) -> ()
                        n1136 = local write "Bridge horizontal offset"(w1917) -> ()
                        n1137 = local write "\"Stop at\" enabled"(w1915) -> ()
                        n1138 = local write "Stop record at"(w1914) -> ()
                        n1139 = local write "Data filtering"(w1908) -> ()
                        n1140 = local write "Name Prefix"(w1926) -> ()
                        n1141 = property on="N segments MIDFIELD" class="DigNum (strict)"("Val(Sgnl)"=w1913) -> (error out=w1911:errorcluster)  [unwired: 2 in, 1 out]
                        n1142 = property on="Stimulus presets" class="Arr (strict)"(error in=w1911, "Value"=w1909) -> ()  [unwired: 1 in, 2 out]
                        n1143 = for {
                          tunnel: [w1935] -> w1910 mode=indexing if=w1933
                          tunnel: w1909 -> [w1934] mode=indexing
                          i -> [w1932]
                          n1144 = Unbundle By Name(w1934) -> ("Stim. has been set"=w1933:bool)
                          n1145 = Greater Than 0?(x=w1932) -> (x > 0?=w1931:bool)
                          n1146 = case shown="True" w1931 {
                            tunnel: w1933 -> [_ w1946]
                            tunnel: w1932 -> [_ w1937]
                            frame False {
                            }
                            frame True {
                              w1941 = refnum<vi> refnum  # Boolean
                              n1147 = Decrement(x=w1937) -> (x-1=w1936:i32)
                              n1148 = property on="Colors for Stim. setup" class="Arr (strict)"() -> ("Value"=w1945:T3)  [unwired: 2 in, 2 out]
                              n1149 = Select(t=w1945, s=w1946, f=T11 [{"Numeric Control"=12369084, "Numeric Control"=12369084}, {"Numeric Control"=6603023, "Numeric Control"=6603023}, {"Numeric Control"=1976113, "Numeric Control"=1976113}, {"Numeric Control"=2575993, "Numeric Control"=2575993}] ("Colors [4] 2")) -> (s? t:f=w1939:T11)
                              n1150 = property on="Zone-based stimulus setup" class="RadioBtnsControl (strict)"() -> ("Controls[]"=w1943:refnum<vi>[])  [unwired: 2 in, 2 out]
                              n1151 = Index Array(array=w1943, index=w1936) -> (element=w1942:refnum<vi>)
                              n1152 = To More Specific Class(target class=w1941, reference=w1942) -> (specific class reference=w1940:refnum<vi>)  [unwired: 1 in, 1 out]
                              n1153 = property class="Bool"(reference=w1940, "Colors [4]"=w1939, "Value"=FALSE) -> ()  [unwired: 1 in, 2 out]
                            }
                          }
                          n1154 = To Unsigned Byte Integer(number=w1932) -> (unsigned 8bit integer=w1935:u8)
                        }
                        n1155 = global write "SW_Globals.vi" "Regions to track"(w1910) -> ()
                        "Settings load path" <- w1928
                      }
                    }
                    n1156 = property on="IO paramaters loaded from file" class="Bool (strict)"(error in=w1886, "Value"=w1885) -> ()  [unwired: 1 in, 2 out]
                  }
                }
                "Adv. Stim. set" <- FALSE ("Adv. Stim. set")
              }
              frame #2 {
                # "Segments scheme can be reset here"
                n1157 = First Call?() -> (First Call?: T/F=w1949:bool)
                n1158 = case shown="True" w1949 {
                  selector: w1949 -> [_ w1952]
                  tunnel: [_ w1951] -> w1950
                  frame False {
                  }
                  frame True {
                    n1159 = property on="Init plot" class="Bool (strict)"("Val(Sgnl)"=w1952) -> (error out=w1951:errorcluster)  [unwired: 2 in, 1 out]
                  }
                }
                n1160 = event shown="[0] \"Init plot\", \"Zone-based stimulus setup\", \"N segments MIDFIELD\", \"N segments BORDER\", \"Starting angle MIDFIELD\", \"Starting angle BORDER\", \"Radius, mm MIDFIELD\", \"Radius, mm CENTER\", \"Cage diameter, mm\", \"Reset stimuli\", \"Reset regions\", \"Reset REG\", \"Reset STIM\", \"Adv. Stim. set\": Value Change" {
                  selector: _ -> [_ _]
                  dyn-events: _ -> [_ _]
                  timeout: 1 -> [_ _]
                  tunnel: w1950 -> [_ _]
                  event "Init plot", "Zone-based stimulus setup", "N segments MIDFIELD", "N segments BORDER", "Starting angle MIDFIELD", "Starting angle BORDER", "Radius, mm MIDFIELD", "Radius, mm CENTER", "Cage diameter, mm", "Reset stimuli", "Reset regions", "Reset REG", "Reset STIM", "Adv. Stim. set": Value Change {
                    n1161 = event-data() -> ()  [unwired: 1 in, 6 out]
                    n1162 = local read "Cage diameter, mm"() -> (w1953:u16)
                    n1163 = case "Let's set flag for alternative magnets orintation" shown="333" w1953 {
                      frame 180, Default {
                        n1164 = global write "SW_Globals.vi" "Alternative magnets orientation"(FALSE ("Alternative magnets orientation")) -> ()
                      }
                      frame 240 {
                        n1165 = global write "SW_Globals.vi" "Alternative magnets orientation"(FALSE ("Alternative magnets orientation")) -> ()
                      }
                      frame 290 {
                        n1166 = global write "SW_Globals.vi" "Alternative magnets orientation"(FALSE ("Alternative magnets orientation")) -> ()
                      }
                      frame 325 {
                        n1167 = global write "SW_Globals.vi" "Alternative magnets orientation"(FALSE ("Alternative magnets orientation")) -> ()
                      }
                      frame 327 {
                        n1168 = global write "SW_Globals.vi" "Alternative magnets orientation"(TRUE ("Alternative magnets orientation")) -> ()
                      }
                      frame 333 {
                        n1169 = global write "SW_Globals.vi" "Alternative magnets orientation"(FALSE ("Alternative magnets orientation")) -> ()
                      }
                    }
                    n1170 = global read "SW_Globals.vi" "Regions to track"() -> (w1975:u8[])
                    n1171 = To Unsigned Byte Integer(number="Zone-based stimulus setup") -> (unsigned 8bit integer=w1976:u8)
                    n1172 = Bundle("N segments BORDER"="N segments BORDER", "Starting angle BORDER"="Starting angle BORDER", "N segments MIDFIELD"="N segments MIDFIELD", "Starting angle MIDFIELD"="Starting angle MIDFIELD", "Radius, mm MIDFIELD"="Radius, mm MIDFIELD", u8 1, "Radius, mm CENTER"="Radius, mm CENTER", "Cage diameter, mm"=w1953, 10) -> (w1963:T52)  [unwired: 1 in]
                    n1173 = property on="Segments diagram" class="Pict"() -> ("Bounds"=w1973:T19)  [unwired: 2 in, 2 out]
                    n1174 = Build Array(w1976) -> (w1972:u8[])
                    n1175 = Build Array (concatenate)(w1972, w1975) -> (w1974:u8[])
                    n1176 = call "SW_Gen_Check_segments_parameters.vi"("Image plotting parameters"=w1963) -> ("Corrected image plotting parameters"=w1962:T53)  [unwired: 2 in]
                    n1177 = Unbundle By Name(w1962) -> ("N segments BORDER"=w1961:u8, "N segments MIDFIELD"=w1959:u8, "Radius, mm MIDFIELD"=w1958:u16, "Radius, mm CENTER"=w1960:u16)
                    n1178 = call "SW_Generate_Segmented_Plot_v3.vi"("Draw Area Size"=w1973, "Regions to mark set"=w1974, "Regions to mark selected"=w1972, "Input cluster of parameters"=w1962) -> ("Zones layout output"=w1955:picture, "No zones image"=w1954:picture, "Array of the pixel to color correspondences"=w1956:u32[][], "Array of the segment to color correspondences"=w1957:u32[][])  [unwired: 6 in, 2 out]
                    "Segments diagram" <- w1955
                    n1179 = global write "SW_Globals.vi" "Full track with zones"(w1955) -> ()
                    n1180 = global write "SW_Globals.vi" "Diagram"(w1955) -> ()
                    n1181 = global write "SW_Globals.vi" "Diagram no zones"(w1954) -> ()
                    n1182 = global write "SW_Globals.vi" "Full track with no zones"(w1954) -> ()
                    n1183 = global write "SW_Globals.vi" "Array of the pixel to color correspondences"(w1956) -> ()
                    n1184 = global write "SW_Globals.vi" "Array of the segment to color correspondences"(w1957) -> ()
                    n1185 = property on="N segments BORDER" class="DigNum (strict)"("Value"=w1961) -> ()  [unwired: 2 in, 2 out]
                    n1186 = property on="N segments MIDFIELD" class="DigNum (strict)"("Value"=w1959) -> ()  [unwired: 2 in, 2 out]
                    n1187 = property on="Radius, mm MIDFIELD" class="DigNum (strict)"("Value"=w1958) -> ()  [unwired: 2 in, 2 out]
                    n1188 = property on="Radius, mm CENTER" class="DigNum (strict)"("Value"=w1960) -> ()  [unwired: 2 in, 2 out]
                  }
                  event Timeout {
                    n1189 = event-data() -> ()  [unwired: 1 in, 3 out]
                  }
                }
              }
              frame #3 {
                # "Save settings and set important variables before actual start of the recording. Also initial \"Play\" command is sent from here."
                n1190 = Build Array("Start Tracking button", "Jump to Analysis") -> (w1987:bool[])
                n1191 = Boolean Array To Number(Boolean array=w1987) -> (number=w1985:u32)
                n1192 = case shown="1" w1985 {
                  tunnel: w1989 -> [_ w2057 w2187]
                  tunnel: w1984 -> [_ w2000 _]
                  frame 0, Default {
                  }
                  frame 1 {
                    w2001 = T54 {"Zone[1]"=FALSE, "Zone[2]"=FALSE, "Zone[3]"=FALSE, "Zone[4]"=FALSE, "Zone[5]"=FALSE, "Zone[6]"=FALSE, "Zone[7]"=FALSE, "Zone[8]"=FALSE, "Zone[9]"=FALSE, "Zone[10]"=FALSE, "Zone[11]"=FALSE, "Zone[12]"=FALSE, "Zone[13]"=FALSE} ("Zones presence indicator")
                    w2091 = enum32{"Settings", "Recording", "Analysis"}."Recording" ("Main tab control")
                    w2095 = enum32{"Settings", "Recording", "Analysis"}."Analysis" ("Main tab control")
                    w2104 = enum32{"Settings", "Recording", "Analysis"}."Settings" ("Main tab control")
                    n1193 = flat-sequence {
                      tunnel: w2057 -> [w2151]
                      tunnel: w2000 -> [w2145]
                      tunnel: [w2151] -> w2056
                      tunnel: w2056 -> [w2153]
                      tunnel: [w2153] -> w2010
                      tunnel: [w2156] -> w1993
                      tunnel: w2010 -> [w2163]
                      frame #0 {
                        n1194 = Unbundle By Name(w2145) -> ("Play/Pause status"=w2149:refnum<notifier>, "Recording now"=w2144:refnum<notifier>, "(Final) Data file is saved"=w2141:refnum<notifier>, "Data loaded"=w2139:refnum<notifier>, "Temp file ready for processing"=w2138:refnum<notifier>, "Has been recorded"=w2135:refnum<notifier>)  [unwired: 1 out]
                        n1195 = Send Notification(notification=FALSE, notifier=w2144) -> ()  [unwired: 1 in, 2 out]
                        n1196 = Send Notification(notification=FALSE, notifier=w2141) -> ()  [unwired: 1 in, 2 out]
                        n1197 = Send Notification(notification=FALSE, notifier=w2139) -> ()  [unwired: 1 in, 2 out]
                        n1198 = Send Notification(notification=FALSE, notifier=w2138) -> ()  [unwired: 1 in, 2 out]
                        n1199 = Send Notification(notification=FALSE, notifier=w2135) -> ()  [unwired: 1 in, 2 out]
                        n1200 = Select(t="Play", s=TRUE, f="Pause") -> (s? t:f=w2148:string)
                        n1201 = Send Notification(notification=w2148, notifier=w2149) -> ()  [unwired: 1 in, 2 out]
                      }
                      frame #1 {
                        n1202 = Wait (ms)(milliseconds to wait=u32 1500) -> ()  [unwired: 1 out]
                      }
                      frame #2 {
                        n1203 = global write "SW_Globals.vi" "Incrementally save First Call"(TRUE ("Incrementally save First Call")) -> ()
                        n1204 = global read "SW_Globals.vi" "Zones allocation array"() -> (w2165:i32[])
                        n1205 = property on="Jump to Analysis" class="Bool (strict)"(error in=w2163, "Value"=FALSE ("Jump to Analysis")) -> (error out=w2161:errorcluster)  [unwired: 1 in, 1 out]
                        n1206 = property on="Record start First Call" class="Bool (strict)"(error in=w2161, "Value"=TRUE ("Record start First Call")) -> (error out=w2159:errorcluster)  [unwired: 1 in, 1 out]
                        n1207 = Array Size(array=w2165) -> (size(s)=w2164:i32)
                        n1208 = Initialize Array(0 ("element"), w2164) -> (w2167:i32[])
                        n1209 = global write "SW_Globals.vi" "Zones allocation array"(w2167) -> ()
                        n1210 = property on="Temp file ready" class="Bool (strict)"(error in=w2159, "Value"=FALSE ("Temp file ready")) -> (error out=w2157:errorcluster)  [unwired: 1 in, 1 out]
                        n1211 = property on="Save files First Call" class="Bool (strict)"(error in=w2157, "Value"=TRUE ("Save files First Call")) -> (error out=w2156:errorcluster)  [unwired: 1 in, 1 out]
                      }
                    }
                    n1212 = property on="Additional record settings" class="Bool (strict)"(error in=w1993, "DisabledEnum"=T12."Enabled" ("Disabled"), "BoolText.Text"="Set" ("Boolean Text.Text")) -> (error out=w1992:errorcluster)  [unwired: 1 in, 1 out]
                    n1213 = property on="Pane" class="Pane"(error in=w1992) -> (error out=w2034:errorcluster, "Decos[]"=w2035:refnum<vi>[])  [unwired: 1 in, 1 out]
                    n1214 = Index Array(array=w2035, index=2) -> (element=w2040:refnum<vi>)
                    n1215 = property class="Decor"(reference=w2040, error in=w2034, "Visible"=FALSE) -> (error out=w2033:errorcluster)  [unwired: 1 out]
                    n1216 = Index Array(array=w2035, index=1) -> (element=w2037:refnum<vi>)
                    n1217 = property class="Decor"(reference=w2037, error in=w2033, "Visible"=TRUE) -> (error out=w2032:errorcluster)  [unwired: 1 out]
                    n1218 = property on="Main tab control" class="TabCtl (strict)"(error in=w2032, "Value"=w2104) -> (error out=w2100:errorcluster, "Pages"=w2105:refnum<vi>[])  [unwired: 1 in, 1 out]
                    n1219 = To Long Integer(number=w2104) -> (32bit integer=w2103:i32)
                    n1220 = Index Array(array=w2105, index=w2103) -> (element=w2102:refnum<vi>)
                    n1221 = property class="Page"(reference=w2102, error in=w2100, "PageEnb"=T32."Page Disabled & Grayed" ("Page Enabled State")) -> (error out=w2093:errorcluster)  [unwired: 1 out]
                    n1222 = property on="Main tab control" class="TabCtl (strict)"(error in=w2093, "Value"=w2095) -> (error out=w2099:errorcluster, "Pages"=w2094:refnum<vi>[])  [unwired: 1 in, 1 out]
                    n1223 = To Long Integer(number=w2095) -> (32bit integer=w2096:i32)
                    n1224 = Index Array(array=w2094, index=w2096) -> (element=w2097:refnum<vi>)
                    n1225 = property class="Page"(reference=w2097, error in=w2099, "PageEnb"=T32."Page Disabled & Grayed" ("Page Enabled State")) -> (error out=w2086:errorcluster)  [unwired: 1 out]
                    n1226 = property on="Main tab control" class="TabCtl (strict)"(error in=w2086, "Value"=w2091) -> (error out=w2087:errorcluster, "Pages"=w2092:refnum<vi>[])  [unwired: 1 in, 1 out]
                    n1227 = To Long Integer(number=w2091) -> (32bit integer=w2090:i32)
                    n1228 = local read "Settings file refnum out"() -> (w2085:T5)
                    n1229 = local read "N segments MIDFIELD"() -> (w2083:u8)
                    n1230 = Index Array(array=w2092, index=w2090) -> (element=w2089:refnum<vi>)
                    n1231 = local read "Current User"() -> (w2012:string)
                    n1232 = local read "N segments BORDER"() -> (w2078:u8)
                    n1233 = property class="Page"(reference=w2089, error in=w2087, "PageEnb"=T32."Page Enabled" ("Page Enabled State")) -> (error out=w2082:errorcluster)  [unwired: 1 out]
                    n1234 = local read "Radius, mm CENTER"() -> (w2077:u16)
                    n1235 = call <vilib>:"Write Key (I32).vi"("section"=w2012, "error in (no error)"=w2082, "value"=w2083, "key"="Amount of midfield segments", "refnum"=w2085) -> ("error out"=w2080:errorcluster, "refnum out"=w2079:T5)  [unwired: 4 in, 1 out]
                    n1236 = local read "Radius, mm MIDFIELD"() -> (w2070:u16)
                    n1237 = call <vilib>:"Write Key (I32).vi"("section"=w2012, "error in (no error)"=w2080, "value"=w2078, "key"="Amount of border segments", "refnum"=w2079) -> ("error out"=w2074:errorcluster, "refnum out"=w2075:T5)  [unwired: 4 in, 1 out]
                    n1238 = local read "Starting angle MIDFIELD"() -> (w2069:i16)
                    n1239 = call <vilib>:"Write Key (I32).vi"("section"=w2012, "error in (no error)"=w2074, "value"=w2077, "key"="Center segment outer radius, mm", "refnum"=w2075) -> ("error out"=w2071:errorcluster, "refnum out"=w2072:T5)  [unwired: 4 in, 1 out]
                    n1240 = local read "Starting angle BORDER"() -> (w2062:i16)
                    n1241 = call <vilib>:"Write Key (I32).vi"("section"=w2012, "error in (no error)"=w2071, "value"=w2070, "key"="Midfield segments outer radius, mm", "refnum"=w2072) -> ("error out"=w2066:errorcluster, "refnum out"=w2067:T5)  [unwired: 4 in, 1 out]
                    n1242 = local read "Cage diameter, mm"() -> (w2042:u16)
                    n1243 = call <vilib>:"Write Key (I32).vi"("section"=w2012, "error in (no error)"=w2066, "value"=w2069, "key"="Midfield segments starting angle", "refnum"=w2067) -> ("error out"=w2064:errorcluster, "refnum out"=w2063:T5)  [unwired: 4 in, 1 out]
                    n1244 = global read "SW_Globals.vi" "Zone-based stimulus presets"() -> (w1999:T49)
                    n1245 = call <vilib>:"Write Key (I32).vi"("section"=w2012, "error in (no error)"=w2064, "value"=w2062, "key"="Border segments starting angle", "refnum"=w2063) -> ("error out"=w2061:errorcluster, "refnum out"=w2060:T5)  [unwired: 4 in, 1 out]
                    n1246 = call <vilib>:"Write Key (I32).vi"("section"=w2012, "error in (no error)"=w2061, "value"=w2042, "key"="Cage diameter, mm", "refnum"=w2060) -> ("error out"=w1996:errorcluster, "refnum out"=w2009:T5)  [unwired: 4 in, 1 out]
                    n1247 = for {
                      tunnel: w1999 -> [w2118] mode=indexing
                      tunnel: w2009 -> [w2111]
                      tunnel: [w2115] -> w2015
                      tunnel: w2012 -> [w2109]
                      i -> [w2114]
                      n1248 = Unbundle By Name(w2118) -> ("Stim. has been set"=w2116:bool)
                      n1249 = Flatten To JSON(anything=w2118) -> (JSON string=w2117:string, 11:w2107:errorcluster)  [unwired: 2 in]
                      n1250 = Format Value(string ("")="Zone " ("string"), format string="%02d", value (0)=w2114) -> (output string=w2108:string)
                      n1251 = call <vilib>:"Remove Key.vi"("section"=w2109, "error in (no error)"=w2107, "key"=w2108, "refnum"=w2111) -> ("error out"=w2106:errorcluster, "refnum out"=w2110:T5)  [unwired: 5 in, 1 out]
                      n1252 = case shown="True" w2116 {
                        tunnel: w2117 -> [_ w2125]
                        tunnel: w2106 -> [_ w2124]
                        tunnel: [w2119 w2123] -> w2115
                        tunnel: w2109 -> [_ w2122]
                        tunnel: w2108 -> [_ w2121]
                        tunnel: w2110 -> [w2119 w2120]
                        frame False {
                        }
                        frame True {
                          n1253 = call <vilib>:"Write Key (String).vi"("section"=w2122, "error in (no error)"=w2124, "value"=w2125, "key"=w2121, "refnum"=w2120) -> ("refnum out"=w2123:T5)  [unwired: 4 in, 2 out]
                        }
                      }
                    }
                    n1254 = global read "SW_Globals.vi" "IO parameters cluster"() -> (w1998:T2)
                    n1255 = local read "N segments MIDFIELD"() -> (w2017:u8)
                    n1256 = local read "N segments BORDER"() -> (w2018:u8)
                    n1257 = property on="Zones presence indicator" class="Clust"() -> ("Controls[]"=w2055:refnum<vi>[])  [unwired: 2 in, 2 out]
                    n1258 = Cluster To Array(cluster=w1998) -> (array=w1990:u16[])
                    n1259 = Flatten To JSON(anything=w1990, error in (no error)=w1996) -> (JSON string=w1997:string, 11:w1995:errorcluster)  [unwired: 1 in]
                    n1260 = Compound Arithmetic op=ADD(w2018, w2017, u8 1 ("value")) -> (w2051:u8)
                    n1261 = Increment(x=w2051) -> (x+1=w2050:u8)
                    n1262 = for {
                      tunnel: w2055 -> [w2134] mode=indexing
                      tunnel: w2051 -> [w2128]
                      tunnel: [w2126] -> w2002
                      i -> [w2133]
                      n1263 = Increment(x=w2133) -> (x+1=w2127:i32)
                      n1264 = Less Or Equal?(x=w2127, y=w2128) -> (x <= y?=w2132:bool)
                      n1265 = Select(t=T12."Disabled" ("Disabled"), s=w2132, f=T12."Disabled and Grayed Out" ("Disabled")) -> (s? t:f=w2130:T12)
                      n1266 = property class="Ctl"(reference=w2134, "DisabledEnum"=w2130) -> (error out=w2126:errorcluster)  [unwired: 1 in, 1 out]
                    }
                    n1267 = global write "SW_Globals.vi" "Active segments amount"(w2051) -> ()
                    n1268 = call <vilib>:"Write Key (String).vi"("section"=w2012, "error in (no error)"=w1995, "value"=w1997, "key"="IO ports configuration", "refnum"=w2015) -> ("error out"=w2014:errorcluster, "refnum out"=w2013:T5)  [unwired: 4 in, 1 out]
                    n1269 = local read "Starting angle MIDFIELD"() -> (w2022:i16)
                    n1270 = local read "Starting angle BORDER"() -> (w2023:i16)
                    n1271 = local read "Radius, mm MIDFIELD"() -> (w2021:u16)
                    n1272 = local read "Radius, mm CENTER"() -> (w2019:u16)
                    n1273 = local read "Cage diameter, mm"() -> (w2016:u16)
                    n1274 = call <vilib>:"Close Config Data.vi"("error in (no error)"=w2014, "refnum"=w2013) -> ("error out"=w2058:errorcluster)  [unwired: 8 in, 1 out]
                    n1275 = Bundle By Name(cluster=T21 {"Minimum"=0.0, "Maximum"=14.0, "Increment"=1.0, "Minor Increment"=1.0, "Start"=0.0} ("X Scale.Range"), "Maximum"=w2050) -> (w2052:T21)
                    n1276 = property on="Diagram at recording" class="Pict"(error in=w2058) -> ("Bounds"=w2031:T19)  [unwired: 1 in, 2 out]
                    n1277 = property on="Histograms (normalized)" class="WFGraph (strict)"("XScale.Range"=w2052, "Caption.Text"="Zone preference (normalized)" ("Label.Text"), "XScale.ScaleFit"=u8 2 ("X Scale.Scale Fit"), "XScale.Ofst&Mult"=T30 {"Offset"=1.0, "Multiplier"=0.0} ("X Scale.Offset and Multiplier"), "YScale.Mapping Mode"=u8 0 ("Y Scale.Mapping Mode")) -> ()  [unwired: 2 in, 2 out]
                    n1278 = Bundle By Name(cluster=T20 {"Amount of border segments"=8, "Border segments starting angle"=0, "Amount of midfield segments"=4, "Midfield segments starting angle"=0, "Midfield segments outer radius, mm"=60, "Amount of central segments"=1, "Center segment outer radius, mm"=30, "Diameter of the cage, mm"=180, "R-gap between segments, mm"=10} ("Input cluster of parameters"), "Amount of border segments"=w2018, "Border segments starting angle"=w2023, "Amount of midfield segments"=w2017, "Midfield segments starting angle"=w2022, "Midfield segments outer radius, mm"=w2021, "Amount of central segments"=u8 1, "Center segment outer radius, mm"=w2019, "Diameter of the cage, mm"=w2016) -> (w2024:T20)
                    n1279 = global read "SW_Globals.vi" "Regions to track"() -> (w2030:u8[])
                    n1280 = call "SW_Generate_Segmented_Plot_v3.vi"("Draw Area Size"=w2031, "Regions to mark set"=w2030, "Input cluster of parameters"=w2024) -> ("Zones layout output"=w2007:picture, "No zones image"=w2008:picture, "Array of the pixel to color correspondences"=w2026:u32[][], "Array of the segment to color correspondences"=w2029:u32[][], "Cluster of image geometrical and scaling parameters"=w2028:T27)  [unwired: 7 in, 1 out]
                    n1281 = global write "SW_Globals.vi" "Diagram"(w2007) -> ()
                    n1282 = global write "SW_Globals.vi" "Full track with zones"(w2007) -> ()
                    n1283 = local write "Diagram at recording"(w2007) -> ()
                    n1284 = global write "SW_Globals.vi" "Diagram no zones"(w2008) -> ()
                    n1285 = global write "SW_Globals.vi" "Full track with no zones"(w2008) -> ()
                    n1286 = global write "SW_Globals.vi" "Array of the pixel to color correspondences"(w2026) -> ()
                    n1287 = global write "SW_Globals.vi" "Array of the segment to color correspondences"(w2029) -> ()
                    n1288 = Unbundle By Name(w2028) -> ("Pixels per mm"=→"Pixels per mm":dbl)
                    n1289 = Array Size(array=w2026) -> (size(s)=w2047:i32[])
                    n1290 = Index Array(array=w2047, index=0) -> (element=w2046:i32)
                    n1291 = Index Array(array=w2047, index=1) -> (element=w2045:i32)
                    n1292 = Initialize Array(u32 0 ("element"), w2046, w2045) -> (w2043:u32[][])
                    n1293 = property on="Zones presence indicator" class="Clust"(error in=w2002, "Value"=w2001) -> ()  [unwired: 1 in, 2 out]
                    n1294 = global write "SW_Globals.vi" "Zones presence indicator"(w2001) -> ()
                    n1295 = global write "SW_Globals.vi" "Array of the presence count"(w2043) -> ()
                  }
                  frame 2 {
                    w2173 = T12."Disabled and Grayed Out" ("Disabled")
                    w2174 = FALSE ("Zones an.")
                    w2193 = enum32{"Settings", "Recording", "Analysis"}."Analysis" ("Main tab control")
                    w2197 = enum32{"Settings", "Recording", "Analysis"}."Recording" ("Main tab control")
                    w2206 = enum32{"Settings", "Recording", "Analysis"}."Settings" ("Main tab control")
                    n1296 = property on="Main tab control" class="TabCtl (strict)"(error in=w2187, "Value"=w2206) -> (error out=w2202:errorcluster, "Pages"=w2207:refnum<vi>[])  [unwired: 1 in, 1 out]
                    n1297 = To Long Integer(number=w2206) -> (32bit integer=w2205:i32)
                    n1298 = Index Array(array=w2207, index=w2205) -> (element=w2204:refnum<vi>)
                    n1299 = property class="Page"(reference=w2204, error in=w2202, "PageEnb"=T32."Page Disabled & Grayed" ("Page Enabled State")) -> (error out=w2195:errorcluster)  [unwired: 1 out]
                    n1300 = property on="Main tab control" class="TabCtl (strict)"(error in=w2195, "Value"=w2197) -> (error out=w2201:errorcluster, "Pages"=w2196:refnum<vi>[])  [unwired: 1 in, 1 out]
                    n1301 = To Long Integer(number=w2197) -> (32bit integer=w2198:i32)
                    n1302 = Index Array(array=w2196, index=w2198) -> (element=w2199:refnum<vi>)
                    n1303 = property class="Page"(reference=w2199, error in=w2201, "PageEnb"=T32."Page Disabled & Grayed" ("Page Enabled State")) -> (error out=w2188:errorcluster)  [unwired: 1 out]
                    n1304 = property on="Main tab control" class="TabCtl (strict)"(error in=w2188, "Value"=w2193) -> (error out=w2189:errorcluster, "Pages"=w2194:refnum<vi>[])  [unwired: 1 in, 1 out]
                    n1305 = To Long Integer(number=w2193) -> (32bit integer=w2192:i32)
                    n1306 = Index Array(array=w2194, index=w2192) -> (element=w2191:refnum<vi>)
                    n1307 = property class="Page"(reference=w2191, error in=w2189, "PageEnb"=T32."Page Enabled" ("Page Enabled State")) -> (error out=w2186:errorcluster)  [unwired: 1 out]
                    n1308 = property on="Zones (analysis)" class="Bool (strict)"(error in=w2186, "Value"=w2174, "DisabledEnum"=w2173) -> (error out=w2185:errorcluster)  [unwired: 1 in, 1 out]
                    n1309 = property on="Show heatmap (analysis)" class="Bool (strict)"("DisabledEnum"=w2173, "Value"=w2174) -> ()  [unwired: 2 in, 2 out]
                    n1310 = property on="Show full track (analysis)" class="Bool (strict)"("DisabledEnum"=w2173, "Value"=w2174) -> ()  [unwired: 2 in, 2 out]
                    n1311 = property on="Play/Pause" class="Bool (strict)"(error in=w2185, "DisabledEnum"=w2173) -> (error out=w2184:errorcluster)  [unwired: 1 in, 1 out]
                    n1312 = property on="Back to Settings" class="Bool (strict)"(error in=w2184, "Visible"=TRUE, "Value"=FALSE ("Back to Settings")) -> (error out=w2179:errorcluster)  [unwired: 1 in, 1 out]
                    n1313 = property on="Pane" class="Pane"(error in=w2179) -> (error out=w2172:errorcluster, "Decos[]"=w2175:refnum<vi>[])  [unwired: 1 in, 1 out]
                    n1314 = Index Array(array=w2175, index=0) -> (element=w2177:refnum<vi>)
                    n1315 = Index Array(array=w2175, index=2) -> (element=w2181:refnum<vi>)
                    n1316 = property on="Map index (analysis)" class="DigNum (strict)"(error in=w2172, "Value"=0 ("Map index (analysis)")) -> (error out=w2169:errorcluster)  [unwired: 1 in, 1 out]
                    n1317 = property class="Decor"(reference=w2177, "Visible"=TRUE) -> ()  [unwired: 1 in, 2 out]
                    n1318 = property class="Decor"(reference=w2181, "Visible"=FALSE) -> ()  [unwired: 1 in, 2 out]
                    n1319 = property on="Jump to Analysis" class="Bool (strict)"(error in=w2169, "Value"=FALSE ("Jump to Analysis")) -> ()  [unwired: 1 in, 2 out]
                  }
                }
              }
            }
          }
          frame "Recording" {
            w2249 = FALSE ("use system decimal point (T)")
            n1320 = Divide(x=u32 1000, y=w2282) -> (x/y=w2281:dbl)
            n1321 = call <extravilib>:"Read.vi"("channel"=w2270) -> ("element"=w2246:string[][])  [unwired: 5 in, 5 out]
            n1322 = First Call?() -> (First Call?: T/F=w2229:bool)
            n1323 = case shown="True" w2229 {
              tunnel: [w2368 w2369] -> w2208
              frame False {
                n1324 = property on="Type of histogram" class="DigNum (strict)"() -> ("Value"=w2368:u8)  [unwired: 2 in, 2 out]
              }
              frame True {
                w2369 = u8 3 ("Value (Signaling)")
                n1325 = property on="Type of histogram" class="DigNum (strict)"("Val(Sgnl)"=w2369) -> ()  [unwired: 2 in, 2 out]
              }
            }
            n1326 = feedback #8(w2277) -> (w2278:u32)
            n1327 = Tick Count (ms)() -> (millisecond timer value=w2279:u32)
            n1328 = feedback-in #8(w2279) -> ()
            n1329 = call "FL_Last_N_Samples_2D_array_of_strings.vi"("BufferLengthSamples"=u32 5, "Input Array of strings"=w2246) -> ("Output Array of strings"=w2245:string[][])
            n1330 = Subtract(x=w2279, y=w2278) -> (x-y=w2276:u32)
            n1331 = Array Size(array=w2245) -> (size(s)=w2263:i32[])
            n1332 = global read "SW_Globals.vi" "Zones presence indicator"() -> (w2244:T54)
            n1333 = Multiply(x=w2281, y="Trace, s") -> (x*y=w2285:dbl)
            n1334 = Index Array(array=w2263, index=0) -> (element=w2261:i32)
            n1335 = Divide(x=w2276, y=u32 1000) -> (x/y=w2271:dbl)
            n1336 = event shown="[3] \"Additional record settings\": Value Change" {
              selector: _ -> [_ _ _ _]
              dyn-events: _ -> [_ _ _ _]
              timeout: 0 -> [_ _ _ _]
              tunnel: w2208 -> [_ _ w2404 _]
              event Timeout {
                n1337 = event-data() -> ()  [unwired: 1 in, 3 out]
              }
              event "Multiplyer of chart RX": Value Change {
                n1338 = event-data() -> ("NewVal"=w2395:u8)  [unwired: 1 in, 5 out]
                n1339 = Multiply(x=w2395, y=10.0) -> (x*y=w2396:dbl)
                n1340 = property on="Mouse speed" class="WFChart (strict)"() -> (error out=w2397:errorcluster, "XScale.Maximum"=w2400:dbl)  [unwired: 2 in, 1 out]
                n1341 = Subtract(x=w2400, y=w2396) -> (x-y=w2398:dbl)
                n1342 = property on="Mouse speed" class="WFChart (strict)"(error in=w2397, "XScale.Minimum"=w2398) -> ()  [unwired: 1 in, 2 out]
              }
              event "Histograms (normalized)": Mouse Down; "Type of histogram": Value Change {
                n1343 = event-data() -> ()  [unwired: 1 in, 4 out]
                n1344 = Increment(x=w2404) -> (x+1=w2401:u8)
                n1345 = Quotient & Remainder(x=w2401, y=u8 4) -> (x-y*floor(x/y)=w2402:u8)  [unwired: 1 out]
                n1346 = property on="Type of histogram" class="DigNum (strict)"("Value"=w2402) -> ()  [unwired: 2 in, 2 out]
                n1347 = case shown="0, Default" w2402 {
                  frame 0, Default {
                    w2405 = FALSE ("Speed distrib. indicator")
                    # "Show zones preference"
                    n1348 = Wait (ms)(milliseconds to wait=u32 100) -> ()  [unwired: 1 out]
                    n1349 = property on="Zones presense indicator" class="Bool (strict)"("Value"=TRUE ("Zones presense indicator")) -> ()  [unwired: 2 in, 2 out]
                    n1350 = property on="Run times distrib. indicator" class="Bool (strict)"("Value"=w2405) -> ()  [unwired: 2 in, 2 out]
                    n1351 = property on="Run lengts distrib. indicator" class="Bool (strict)"("Value"=w2405) -> ()  [unwired: 2 in, 2 out]
                    n1352 = property on="Speed distrib. indicator" class="Bool (strict)"("Value"=w2405) -> ()  [unwired: 2 in, 2 out]
                    n1353 = global read "SW_Globals.vi" "Active segments amount"() -> (w2418:u8)
                    n1354 = Increment(x=w2418) -> (x+1=w2417:u8)
                    n1355 = global read "SW_Globals.vi" "Zones normalized allocation array"() -> (w2411:dbl[])
                    n1356 = Bundle By Name(cluster=T21 {"Minimum"=0.0, "Maximum"=14.0, "Increment"=1.0, "Minor Increment"=1.0, "Start"=0.0} ("X Scale.Range"), "Maximum"=w2417) -> (w2419:T21)
                    n1357 = property on="Histograms (normalized)" class="WFGraph (strict)"("XScale.Range"=w2419, "Caption.Text"="Zone preference (normalized)" ("Label.Text"), "XScale.Multiplier"=1.0 ("X Scale.Offset and Multiplier:Multiplier"), "XScale.Offset"=0.0 ("X Scale.Offset and Multiplier:Offset"), "XScale.ScaleFit"=u8 2 ("X Scale.Scale Fit"), "YScale.Mapping Mode"=u8 0 ("Y Scale.Mapping Mode"), "Value"=w2411, "Plot.Fill/Pt. Color"=u32 15790320 ("Plot.Fill/Point Color"), "XScale.ScaleFit"=u8 1 ("X Scale.Scale Fit"), "XScale.Precision"=u8 0 ("X Scale.Display Format:Precision")) -> ()  [unwired: 2 in, 2 out]
                  }
                  frame 1 {
                    w2421 = FALSE ("Zones presense indicator")
                    # "Speed distribution"
                    n1358 = Wait (ms)(milliseconds to wait=u32 100) -> ()  [unwired: 1 out]
                    n1359 = property on="Speed distrib. indicator" class="Bool (strict)"("Value"=TRUE ("Speed distrib. indicator")) -> ()  [unwired: 2 in, 2 out]
                    n1360 = property on="Run times distrib. indicator" class="Bool (strict)"("Value"=w2421) -> ()  [unwired: 2 in, 2 out]
                    n1361 = property on="Run lengts distrib. indicator" class="Bool (strict)"("Value"=w2421) -> ()  [unwired: 2 in, 2 out]
                    n1362 = property on="Zones presense indicator" class="Bool (strict)"("Value"=w2421) -> ()  [unwired: 2 in, 2 out]
                    n1363 = global read "SW_Globals.vi" "Speed bins array"() -> (w2434:dbl[])
                    n1364 = Array Size(array=w2434) -> (size(s)=w2436:i32)
                    n1365 = global read "SW_Globals.vi" "Speed distribution array"() -> (w2427:u32[])
                    n1366 = Decrement(x=w2436) -> (x-1=w2430:i32)
                    n1367 = property on="Histograms (normalized)" class="WFGraph (strict)"("XScale.ScaleFit"=u8 0 ("X Scale.Scale Fit")) -> (error out=w2429:errorcluster)  [unwired: 2 in, 1 out]
                    n1368 = Bundle By Name(cluster=T21 {"Minimum"=0.0, "Maximum"=14.0, "Increment"=1.0, "Minor Increment"=1.0, "Start"=0.0} ("X Scale.Range"), "Maximum"=w2430) -> (w2437:T21)
                    n1369 = call "SW_Get_1D_Array_normalize.vi"("1D array"=w2427) -> ("Normalized 1D array"=w2426:dbl[])  [unwired: 2 in, 1 out]
                    n1370 = property on="Histograms (normalized)" class="WFGraph (strict)"(error in=w2429, "XScale.Range"=w2437, "Caption.Text"="Speed histogram (normalized)" ("Label.Text"), "XScale.Multiplier"=36.5 ("X Scale.Offset and Multiplier:Multiplier 2"), "XScale.Offset"=0 ("index"), "YScale.Mapping Mode"=u8 1 ("X Scale.Scale Fit"), "Value"=w2426, "Plot.Fill/Pt. Color"=u32 16777120 ("Plot.Fill/Point Color"), "XScale.ScaleFit"=u8 0 ("X Scale.Scale Fit")) -> ()  [unwired: 1 in, 2 out]
                  }
                  frame 2 {
                    w2439 = FALSE ("Zones presense indicator")
                    # "Runing bout distribution"
                    n1371 = Wait (ms)(milliseconds to wait=u32 100) -> ()  [unwired: 1 out]
                    n1372 = property on="Run lengts distrib. indicator" class="Bool (strict)"("Value"=TRUE ("Speed distrib. indicator")) -> ()  [unwired: 2 in, 2 out]
                    n1373 = property on="Run times distrib. indicator" class="Bool (strict)"("Value"=w2439) -> ()  [unwired: 2 in, 2 out]
                    n1374 = property on="Speed distrib. indicator" class="Bool (strict)"("Value"=w2439) -> ()  [unwired: 2 in, 2 out]
                    n1375 = property on="Zones presense indicator" class="Bool (strict)"("Value"=w2439) -> ()  [unwired: 2 in, 2 out]
                    n1376 = global read "SW_Globals.vi" "Run Lengths bins array"() -> (w2445:dbl[])
                    n1377 = Array Size(array=w2445) -> (size(s)=w2459:i32)
                    n1378 = Decrement(x=w2459) -> (x-1=w2440:i32)
                    n1379 = global read "SW_Globals.vi" "Run Lengts distribution array"() -> (w2452:u32[])
                    n1380 = property on="Histograms (normalized)" class="WFGraph (strict)"("XScale.ScaleFit"=u8 0 ("X Scale.Scale Fit")) -> (error out=w2454:errorcluster)  [unwired: 2 in, 1 out]
                    n1381 = Array Subset(array=w2445, index=0, length=w2440) -> ()  [unwired: 1 out]
                    n1382 = Bundle By Name(cluster=T21 {"Minimum"=0.0, "Maximum"=2.0, "Increment"=0.2, "Minor Increment"=0.2, "Start"=0.0} ("X Scale.Range"), "Maximum"=w2440) -> (w2441:T21)
                    n1383 = call "SW_Get_1D_Array_normalize.vi"("1D array"=w2452) -> ("Normalized 1D array"=w2451:dbl[])  [unwired: 2 in, 1 out]
                    n1384 = property on="Histograms (normalized)" class="WFGraph (strict)"(error in=w2454, "XScale.Range"=w2441, "Caption.Text"="Running bout dist. hist. (norm.)" ("Label.Text"), "XScale.Multiplier"=0.2 ("X Scale.Offset and Multiplier:Multiplier 2"), "XScale.Offset"=0.2 ("index"), "YScale.Mapping Mode"=u8 0 ("X Scale.Scale Fit"), "Value"=w2451, "Plot.Fill/Pt. Color"=u32 12320699 ("Plot.Fill/Point Color"), "XScale.ScaleFit"=u8 1 ("X Scale.Scale Fit"), "XScale.Format"=u8 0 ("X Scale.Display Format:Format"), "XScale.Precision"=u8 1 ("X Scale.Display Format:Precision")) -> ()  [unwired: 1 in, 2 out]
                  }
                  frame 3 {
                    w2460 = FALSE ("Zones presense indicator")
                    # "Running times distribution"
                    n1385 = Wait (ms)(milliseconds to wait=u32 100) -> ()  [unwired: 1 out]
                    n1386 = property on="Run times distrib. indicator" class="Bool (strict)"("Value"=TRUE ("Run times distrib. indicator")) -> ()  [unwired: 2 in, 2 out]
                    n1387 = property on="Run lengts distrib. indicator" class="Bool (strict)"("Value"=w2460) -> ()  [unwired: 2 in, 2 out]
                    n1388 = property on="Speed distrib. indicator" class="Bool (strict)"("Value"=w2460) -> ()  [unwired: 2 in, 2 out]
                    n1389 = property on="Zones presense indicator" class="Bool (strict)"("Value"=w2460) -> ()  [unwired: 2 in, 2 out]
                    n1390 = global read "SW_Globals.vi" "Run Times bins array"() -> (w2467:dbl[])
                    n1391 = Array Size(array=w2467) -> (size(s)=w2480:i32)
                    n1392 = Decrement(x=w2480) -> (x-1=w2462:i32)
                    n1393 = global read "SW_Globals.vi" "Run Times distribution array"() -> (w2473:u32[])
                    n1394 = property on="Histograms (normalized)" class="WFGraph (strict)"("XScale.ScaleFit"=u8 0 ("X Scale.Scale Fit")) -> (error out=w2475:errorcluster)  [unwired: 2 in, 1 out]
                    n1395 = Array Subset(array=w2467, index=0, length=w2462) -> ()  [unwired: 1 out]
                    n1396 = Bundle By Name(cluster=T21 {"Minimum"=0.0, "Maximum"=2.0, "Increment"=0.2, "Minor Increment"=0.2, "Start"=0.0} ("X Scale.Range"), "Maximum"=w2462) -> (w2463:T21)
                    n1397 = call "SW_Get_1D_Array_normalize.vi"("1D array"=w2473) -> ("Normalized 1D array"=w2472:dbl[])  [unwired: 2 in, 1 out]
                    n1398 = property on="Histograms (normalized)" class="WFGraph (strict)"(error in=w2475, "XScale.Range"=w2463, "Caption.Text"="Run times dist. hist. (norm.)" ("Label.Text"), "XScale.Multiplier"=1.0 ("X Scale.Offset and Multiplier:Multiplier 2"), "XScale.Offset"=0.5 ("index"), "YScale.Mapping Mode"=u8 0 ("X Scale.Scale Fit"), "Value"=w2472, "Plot.Fill/Pt. Color"=u32 16771022 ("Plot.Fill/Point Color"), "XScale.ScaleFit"=u8 1 ("X Scale.Scale Fit"), "XScale.Format"=u8 0 ("X Scale.Display Format:Format"), "XScale.Precision"=u8 1 ("X Scale.Display Format:Precision")) -> ()  [unwired: 1 in, 2 out]
                  }
                }
              }
              event "Additional record settings": Value Change {
                n1399 = event-data() -> ("OldVal"=w2498:bool)  [unwired: 1 in, 5 out]
                n1400 = property on="Additional record settings" class="Bool (strict)"("Value"=w2498) -> ()  [unwired: 2 in, 2 out]
                n1401 = property on="Twisted neck" class="Bool (strict)"() -> ("Value"=w2485:bool)  [unwired: 2 in, 2 out]
                n1402 = property on="Bridge horizontal offset" class="DigNum (strict)"() -> ("Value"=w2484:sgl)  [unwired: 2 in, 2 out]
                n1403 = property on="Name Prefix" class="Str"() -> ("Value"=w2483:string)  [unwired: 2 in, 2 out]
                n1404 = property on="Stop record at" class="DigNum (strict)"() -> ("Value"=w2482:dbl)  [unwired: 2 in, 2 out]
                n1405 = property on="Bridge offset" class="DigNum (strict)"() -> ("Value"=w2495:sgl)  [unwired: 2 in, 2 out]
                n1406 = property on="Bridge swap" class="Bool (strict)"() -> ("Value"=w2494:bool)  [unwired: 2 in, 2 out]
                n1407 = property on="\"Stop at\" enabled" class="Bool (strict)"() -> ("Value"=w2481:bool)  [unwired: 2 in, 2 out]
                n1408 = Bundle By Name(cluster=T46 {"Offset V."=0.0, "Offset H."=0.0, "Bridge swap"=FALSE, "Twisted neck"=FALSE, "Name prefix"="SavedTrack", "Stop at"=0.0, "\"Stop at\" enabled"=FALSE} ("Offsets, swaps and rotations in"), "Offset V."=w2495, "Bridge swap"=w2494, "Twisted neck"=w2485, "Name prefix"=w2483, "Stop at"=w2482, "\"Stop at\" enabled"=w2481, "Offset H."=w2484) -> (w2496:T46)
                n1409 = call "SW_Set_Add_Recording_Settings.vi"("Offsets, swaps and rotations in"=w2496) -> ("Offsets, swaps and rotations out"=w2493:T46)  [unwired: 1 in]
                n1410 = Unbundle By Name(w2493) -> ("Offset V."=w2492:sgl, "Offset H."=w2489:sgl, "Bridge swap"=w2491:bool, "Twisted neck"=w2490:bool, "Name prefix"=w2486:string, "Stop at"=w2488:dbl, "\"Stop at\" enabled"=w2487:bool)
                n1411 = property on="\"Stop at\" enabled" class="Bool (strict)"("Value"=w2487) -> ()  [unwired: 2 in, 2 out]
                n1412 = property on="Bridge offset" class="DigNum (strict)"("Value"=w2492) -> ()  [unwired: 2 in, 2 out]
                n1413 = property on="Name Prefix" class="Str"("Value"=w2486) -> ()  [unwired: 2 in, 2 out]
                n1414 = property on="Stop record at" class="DigNum (strict)"("Value"=w2488) -> ()  [unwired: 2 in, 2 out]
                n1415 = property on="Bridge swap" class="Bool (strict)"("Value"=w2491) -> ()  [unwired: 2 in, 2 out]
                n1416 = property on="Bridge horizontal offset" class="DigNum (strict)"("Value"=w2489) -> ()  [unwired: 2 in, 2 out]
                n1417 = property on="Twisted neck" class="Bool (strict)"("Value"=w2490) -> ()  [unwired: 2 in, 2 out]
                n1418 = disable-structure shown="Disabled" {
                  disable-tunnel: w2486 -> [w2499 _]
                  frame Disabled {
                    n1419 = global read "SW_Globals.vi" "Cluster of paths"() -> (w2501:T22)
                    n1420 = call "SW_Get_save_paths.vi"("Input cluster of paths"=w2501, "Final file name prefix"=w2499) -> ("Output cluster of paths"=w2500:T22)  [unwired: 2 in, 2 out]
                    n1421 = global write "SW_Globals.vi" "Cluster of paths"(w2500) -> ()
                  }
                  frame Enabled {
                  }
                }
              }
            }
            n1422 = Round To Nearest(number=w2285) -> (nearest integer value=w2284:dbl)
            n1423 = Decrement(x=w2261) -> (x-1=w2260:i32)
            n1424 = property on="Zones presence indicator" class="Clust"("Value"=w2244) -> ()  [unwired: 2 in, 2 out]
            n1425 = Index Array(array=w2245, index (row)=w2260) -> (element=w2209:string[])  [unwired: 1 in]
            n1426 = Index Array "Timestamp"(array=w2209, index=4) -> (element=w2258:string)
            n1427 = Index Array "X (filtered)"(array=w2209, index=9) -> (element=w2252:string)
            n1428 = Index Array "Y (filtered)"(array=w2209, index=10) -> (element=w2251:string)
            n1429 = Index Array "w (mouse rot. angle)"(array=w2209, index=8) -> (element=w2250:string)
            n1430 = global read "SW_Globals.vi" "Diagram no zones"() -> (w2291:picture)
            n1431 = String Length(string=w2258) -> (length=w2257:i32)
            n1432 = Fract/Exp String To Number(use system decimal point (T)=w2249, string=w2252) -> (number=w2211:dbl)  [unwired: 2 in, 1 out]
            n1433 = Fract/Exp String To Number(use system decimal point (T)=w2249, string=w2251) -> (number=w2212:dbl)  [unwired: 2 in, 1 out]
            n1434 = global read "SW_Globals.vi" "Diagram"() -> (w2292:picture)
            n1435 = property on="Diagram at recording" class="Pict"() -> ("Bounds"=w2289:T19)  [unwired: 2 in, 2 out]
            n1436 = global read "SW_Globals.vi" "Speed bins array"() -> (w2242:dbl[])
            n1437 = local read "Pixels per mm"() -> (w2290:dbl)
            n1438 = Fract/Exp String To Number(use system decimal point (T)=w2249, string=w2250) -> (number=w2210:dbl)  [unwired: 2 in, 1 out]
            n1439 = Select(t=w2292, s="Zones", f=w2291) -> (s? t:f=w2293:picture)
            n1440 = Greater Than 0?(x=w2257) -> (x > 0?=w2256:bool)
            n1441 = Not(x="Zones") -> (.not. x?=w2287:bool)
            n1442 = call "FL_Calc_speed_on_the_fly.vi"("Y coord, mm"=w2212, "X coord, mm"=w2211, "Time per frame, s"=w2271) -> ("Mouse speed, mm/s"=w2225:dbl)
            "Mouse speed digi" <- w2225
            n1443 = global read "SW_Globals.vi" "Speed distribution array"() -> (w2238:u32[])
            n1444 = case shown="True" w2256 {
              tunnel: [w2373 w2376] -> w2213
              tunnel: w2258 -> [_ w2375]
              frame False {
                n1445 = Get Date/Time In Seconds() -> (seconds since 1Jan1904=w2373:timestamp)
              }
              frame True {
                (unwired) "%<%H:%M:%S%3u%p%d.%m.%Y>T" ("format string")
                n1446 = Get Date/Time In Seconds() -> (seconds since 1Jan1904=w2374:timestamp)
                n1447 = Scan From String(format string="%<%H:%M:%S%,;%3u %d.%m.%Y>T", input string=w2375, default 1=w2374) -> (output 1=w2376:timestamp)  [unwired: 2 in, 3 out]
              }
            }
            n1448 = call "SW_Draw_mouse_br.vi"("Input picture (background)"=w2293, "Size of the image"=w2289, "Pixels per mm"=w2290, "Mouse coord cartesian X, mm"=w2211, "Mouse coord cartesian Y, mm"=w2212, "Mouse angle of rotation, deg"=w2210, "Show mouse lineout"=w2287, "Trace length, samples"=w2284) -> ("Output picture (with mouse overlay)"=→"Diagram at recording":picture)  [unwired: 6 in, 1 out]
            n1449 = call "FL_Get_Histogram_Bin_number.vi"("Current value"=w2225, "Bins array"=w2242) -> ("Bin assignment"=w2241:i32)
            n1450 = global read "SW_Globals.vi" "Run Lengts distribution array"() -> (w2223:u32[])
            n1451 = global read "SW_Globals.vi" "Run Times distribution array"() -> (w2220:u32[])
            n1452 = global read "SW_Globals.vi" "Run Lengths bins array"() -> (w2222:dbl[])
            n1453 = Index Array(array=w2238, index=w2241) -> (element=w2240:u32)
            n1454 = global read "SW_Globals.vi" "Run Times bins array"() -> (w2219:dbl[])
            n1455 = global read "SW_Globals.vi" "Speed detection threshold, mm/s"() -> (w2214:dbl)
            n1456 = Increment(x=w2240) -> (x+1=w2239:u32)
            n1457 = call "FL_Get_Run_Bout_and_Time.vi"("Speed, mm/s"=w2225, "Run Lengts distribution array in"=w2223, "Speed lower threshold, mm/s"=w2214, "Run times distribution array in"=w2220, "Run Lengths bin array"=w2222, "Run times bin array"=w2219) -> ("Run Lengts distribution array out"=w2221:u32[], "Run time, s"=w2216:dbl, "Run times distribution array out"=w2218:u32[])  [unwired: 1 in]
            n1458 = Replace Array Subset(array=w2238, new element=w2239, index=w2241) -> (w2237:u32[])
            n1459 = property on="Type of histogram" class="DigNum (strict)"() -> ("Value"=w2226:u8)  [unwired: 2 in, 2 out]
            n1460 = global write "SW_Globals.vi" "Run Lengts distribution array"(w2221) -> ()
            n1461 = global write "SW_Globals.vi" "Run time, s"(w2216) -> ()
            n1462 = global write "SW_Globals.vi" "Run Times distribution array"(w2218) -> ()
            n1463 = global write "SW_Globals.vi" "Speed distribution array"(w2237) -> ()
            n1464 = call "SW_Get_1D_Array_normalize.vi"("1D array"=w2221) -> ("Normalized 1D array"=w2224:dbl[])  [unwired: 2 in, 1 out]
            n1465 = call "SW_Get_1D_Array_normalize.vi"("1D array"=w2218) -> ("Normalized 1D array"=w2217:dbl[])  [unwired: 2 in, 1 out]
            n1466 = call "SW_Get_1D_Array_normalize.vi"("1D array"=w2237) -> ("Normalized 1D array"=w2227:dbl[])  [unwired: 2 in, 1 out]
            n1467 = case shown="0, Default" w2226 {
              tunnel: [w2364 w2365 w2366 w2367] -> w2228
              tunnel: w2227 -> [_ w2365 _ _]
              tunnel: w2224 -> [_ _ w2366 _]
              tunnel: w2217 -> [_ _ _ w2367]
              frame 0, Default {
                n1468 = global read "SW_Globals.vi" "Zones normalized allocation array"() -> (w2364:dbl[])
              }
              frame 1 {
              }
              frame 2 {
              }
              frame 3 {
              }
            }
            "Histograms (normalized)" <- w2228
            n1469 = Delete From Array(array=w2227, length=1, index=0) -> (array with subset deleted=w2234:dbl[])  [unwired: 1 out]
            n1470 = for {
              tunnel: w2234 -> [w2372] mode=indexing
              shift-right: [w2371] -> w2232
              shift-left: 0.0 -> [w2370]
              n1471 = Add(x=w2370, y=w2372) -> (x+y=w2371:dbl)
            }
            n1472 = Not(x="Exit (recording)") -> (.not. x?=w2266:bool)
            n1473 = And(x=w2266, y="Record/Stop") -> (x .and. y?=w2267:bool)
            n1474 = Multiply(x=w2232, y=100.0) -> (x*y=→"Mouse running, perc. of time":dbl)
            n1475 = Build Array(w2225) -> (w2269:dbl[])
            n1476 = property on="Current Time" class="AbsTime (strict)"("Value"=w2213) -> ()  [unwired: 2 in, 2 out]
            n1477 = Bundle By Name("t0"=w2213, "Y"=w2269) -> (→"Mouse speed":waveform(dbl))  [unwired: 1 in]
            n1478 = case shown="True" w2267 {
              tunnel: w2215 -> [w2504 w2598]
              tunnel: w2213 -> [_ w2597]
              tunnel: w2280 -> [_ w2596]
              tunnel: [w2506 w2594] -> w2272
              tunnel: "Exit (recording)" -> [w2503 _]
              frame False {
                n1479 = Unbundle By Name(w2504) -> ("Has been recorded"=w2508:refnum<notifier>)
                n1480 = Get Notifier Status(notifier=w2508) -> (current notification=w2502:bool, error out=w2507:errorcluster)  [unwired: 1 in, 3 out]
                n1481 = Or(x=w2503, y=w2502) -> (x .or. y?=w2505:bool)
                n1482 = case shown="False" w2505 {
                  tunnel: w2504 -> [_ w2571]
                  tunnel: w2507 -> [_ w2550]
                  tunnel: [FALSE FALSE] -> w2506
                  tunnel: w2502 -> [_ w2530]
                  frame False {
                    w2509 = FALSE ("Show full track (analysis)")
                    n1483 = property on="Start TTL is fired" class="Bool (strict)"("Value"=FALSE ("Start TTL is fired")) -> ()  [unwired: 2 in, 2 out]
                    n1484 = property on="Stop TTL is fired" class="Bool (strict)"("Value"=FALSE ("Start TTL is fired")) -> ()  [unwired: 2 in, 2 out]
                    n1485 = property on="Show full track (analysis)" class="Bool (strict)"("Value"=w2509) -> ()  [unwired: 2 in, 2 out]
                    n1486 = property on="Show heatmap (analysis)" class="Bool (strict)"("Value"=w2509) -> ()  [unwired: 2 in, 2 out]
                    n1487 = disable-structure shown="Disabled" {
                      frame Disabled {
                        n1488 = global read "SW_Globals.vi" "Cluster of paths"() -> (w2522:T22)
                        n1489 = Unbundle By Name(w2522) -> ("Path to the settings file"=w2515:path)
                        n1490 = property on="Bridge swap" class="Bool (strict)"() -> (error out=w2516:errorcluster, "Value"=w2513:bool)  [unwired: 2 in, 1 out]
                        n1491 = local read "Current User"() -> (w2514:string)
                        n1492 = call <vilib>:"Open Config Data.vi"("error in (no error)"=w2516, "create file if necessary (T)"=w2513, "configuration file path"=w2515) -> ("error out"=w2519:errorcluster, "refnum"=w2521:T5)  [unwired: 6 in, 1 out]
                        n1493 = call <vilib>:"Write Key (Boolean).vi"("section"=w2514, "error in (no error)"=w2519, "key"="Bridge swap?", "refnum"=w2521) -> ("error out"=w2518:errorcluster, "refnum out"=w2520:T5)  [unwired: 5 in, 1 out]
                        n1494 = call <vilib>:"Close Config Data.vi"("error in (no error)"=w2518, "refnum"=w2520) -> ()  [unwired: 8 in, 2 out]
                      }
                      frame Enabled {
                      }
                    }
                  }
                  frame True {
                    w2556 = enum32{"Settings", "Recording", "Analysis"}."Analysis" ("Main tab control")
                    w2560 = enum32{"Settings", "Recording", "Analysis"}."Recording" ("Main tab control")
                    w2569 = enum32{"Settings", "Recording", "Analysis"}."Settings" ("Main tab control")
                    n1495 = flat-sequence {
                      tunnel: w2571 -> [w2579]
                      tunnel: w2550 -> [w2575]
                      tunnel: [w2572] -> w2549
                      tunnel: [w2581] -> w2525
                      tunnel: w2549 -> [w2581]
                      frame #0 {
                        n1496 = Unbundle By Name(w2579) -> ("Play/Pause status"=w2580:refnum<notifier>, "Recording now"=w2577:refnum<notifier>)
                        n1497 = Send Notification(notification=FALSE, notifier=w2577, error in (no error)=w2575) -> (error out=w2573:errorcluster)  [unwired: 1 out]
                        n1498 = Send Notification(notification="Pause" ("f"), notifier=w2580) -> (error out=w2574:errorcluster)  [unwired: 1 in, 1 out]
                        n1499 = Merge Errors(w2574, w2573) -> (w2572:errorcluster)
                      }
                      frame #1 {
                        n1500 = Wait (ms)(milliseconds to wait=u32 500) -> ()  [unwired: 1 out]
                      }
                    }
                    n1501 = property on="Additional record settings" class="Bool (strict)"(error in=w2525, "BoolText.Text"="Set" ("Boolean Text.Text")) -> (error out=w2524:errorcluster)  [unwired: 1 in, 1 out]
                    n1502 = property on="Exit (recording)" class="Bool"(error in=w2524, "DisabledEnum"=T12."Enabled" ("Disabled")) -> (error out=w2548:errorcluster)  [unwired: 1 in, 1 out]
                    n1503 = property on="Main tab control" class="TabCtl (strict)"(error in=w2548, "Value"=w2569) -> (error out=w2565:errorcluster, "Pages"=w2570:refnum<vi>[])  [unwired: 1 in, 1 out]
                    n1504 = To Long Integer(number=w2569) -> (32bit integer=w2568:i32)
                    n1505 = Index Array(array=w2570, index=w2568) -> (element=w2567:refnum<vi>)
                    n1506 = property class="Page"(reference=w2567, error in=w2565, "PageEnb"=T32."Page Disabled & Grayed" ("Page Enabled State")) -> (error out=w2558:errorcluster)  [unwired: 1 out]
                    n1507 = property on="Main tab control" class="TabCtl (strict)"(error in=w2558, "Value"=w2560) -> (error out=w2564:errorcluster, "Pages"=w2559:refnum<vi>[])  [unwired: 1 in, 1 out]
                    n1508 = To Long Integer(number=w2560) -> (32bit integer=w2561:i32)
                    n1509 = Index Array(array=w2559, index=w2561) -> (element=w2562:refnum<vi>)
                    n1510 = property class="Page"(reference=w2562, error in=w2564, "PageEnb"=T32."Page Disabled & Grayed" ("Page Enabled State")) -> (error out=w2551:errorcluster)  [unwired: 1 out]
                    n1511 = property on="Main tab control" class="TabCtl (strict)"(error in=w2551, "Value"=w2556) -> (error out=w2552:errorcluster, "Pages"=w2557:refnum<vi>[])  [unwired: 1 in, 1 out]
                    n1512 = To Long Integer(number=w2556) -> (32bit integer=w2555:i32)
                    n1513 = Index Array(array=w2557, index=w2555) -> (element=w2554:refnum<vi>)
                    n1514 = property class="Page"(reference=w2554, error in=w2552, "PageEnb"=T32."Page Enabled" ("Page Enabled State")) -> (error out=w2537:errorcluster)  [unwired: 1 out]
                    n1515 = property on="Pane" class="Pane"(error in=w2537) -> (error out=w2536:errorcluster, "Decos[]"=w2538:refnum<vi>[])  [unwired: 1 in, 1 out]
                    n1516 = Index Array(array=w2538, index=1) -> (element=w2543:refnum<vi>)
                    n1517 = property class="Decor"(reference=w2543, error in=w2536, "Visible"=FALSE) -> (error out=w2535:errorcluster)  [unwired: 1 out]
                    n1518 = Index Array(array=w2538, index=0) -> (element=w2540:refnum<vi>)
                    n1519 = property class="Decor"(reference=w2540, error in=w2535, "Visible"=TRUE) -> (error out=w2534:errorcluster)  [unwired: 1 out]
                    n1520 = property on="Back to Settings" class="Bool (strict)"(error in=w2534, "Visible"=TRUE) -> (error out=w2527:errorcluster)  [unwired: 1 in, 1 out]
                    n1521 = Select(t=T12."Enabled" ("Disabled"), s=w2530, f=T12."Disabled and Grayed Out" ("Disabled")) -> (s? t:f=w2529:T12)
                    n1522 = property on="Show heatmap (analysis)" class="Bool (strict)"(error in=w2527, "DisabledEnum"=w2529) -> (error out=w2532:errorcluster)  [unwired: 1 in, 1 out]
                    n1523 = property on="Show full track (analysis)" class="Bool (strict)"(error in=w2532, "DisabledEnum"=w2529) -> (error out=w2531:errorcluster)  [unwired: 1 in, 1 out]
                    n1524 = property on="Map index (analysis)" class="DigNum (strict)"(error in=w2531, "Value"=0 ("Map index (analysis)")) -> ()  [unwired: 1 in, 2 out]
                  }
                }
              }
              frame True {
                n1525 = flat-sequence {
                  tunnel: w2597 -> [w2608]
                  tunnel: [w2615] -> w2599
                  tunnel: w2598 -> [w2612]
                  tunnel: w2597 -> [w2610]
                  tunnel: [w2610] -> w2595
                  tunnel: w2596 -> [w2609]
                  tunnel: [w2607] -> w2594
                  frame #0 {
                    n1526 = case shown="True" "Record start First Call" {
                      tunnel: w2608 -> [_ w2698]
                      tunnel: [w2620 w2698] -> w2615
                      tunnel: [_ w2713] -> w2611
                      tunnel: w2609 -> [_ w2719]
                      tunnel: [FALSE TRUE] -> w2607
                      frame False {
                        n1527 = global read "SW_Globals.vi" "Recording start timestamp"() -> (w2620:timestamp)
                      }
                      frame True {
                        w2640 = FALSE ("use system decimal point (T)")
                        w2680 = 400
                        w2679 = "NI_MinimumBufferSize"
                        w2660 = T12."Disabled and Grayed Out" ("Disabled")
                        n1528 = property on="Record start First Call" class="Bool (strict)"("Value"=FALSE ("Record start First Call")) -> ()  [unwired: 2 in, 2 out]
                        n1529 = property on="Stimulus presets" class="Arr (strict)"() -> ("Value"=w2690:T7)  [unwired: 2 in, 2 out]
                        n1530 = for {
                          tunnel: w2690 -> [w2744] mode=indexing
                          shift-right: [w2737] -> w2688
                          shift-left: string[] [] -> [w2736]
                          i -> [w2743]
                          n1531 = Unbundle By Name(w2744) -> ("Stim. has been set"=w2740:bool)
                          n1532 = Flatten To JSON(anything=w2744) -> (JSON string=w2738:string)  [unwired: 2 in, 1 out]
                          n1533 = Format Value(string ("")="Zone " ("string"), format string="%02d", value (0)=w2743) -> (output string=w2739:string)
                          n1534 = case shown="True" w2740 {
                            tunnel: w2739 -> [_ w2751]
                            tunnel: w2738 -> [_ w2749]
                            tunnel: [w2745 w2747] -> w2737
                            tunnel: w2736 -> [w2745 w2746]
                            frame False {
                            }
                            frame True {
                              n1535 = Concatenate Strings(w2751, ": " ("string"), w2749) -> (w2748:string)
                              n1536 = Build Array (concatenate)(w2746, w2748) -> (w2747:string[])
                            }
                          }
                        }
                        n1537 = property on="\"Stop at\" enabled" class="Bool (strict)"() -> ("Value"=w2635:bool)  [unwired: 2 in, 2 out]
                        n1538 = property on="Stop record at" class="DigNum (strict)"() -> ("Value"=w2638:dbl)  [unwired: 2 in, 2 out]
                        n1539 = property on="Bridge horizontal offset" class="DigNum (strict)"() -> ("Value"=w2648:sgl)  [unwired: 2 in, 2 out]
                        n1540 = property on="Twisted neck" class="Bool (strict)"() -> ("Value"=w2653:bool)  [unwired: 2 in, 2 out]
                        n1541 = local read "Starting angle MIDFIELD"() -> (w2705:i16)
                        n1542 = local read "Starting angle BORDER"() -> (w2708:i16)
                        n1543 = local read "N segments MIDFIELD"() -> (w2706:u8)
                        n1544 = local read "Radius, mm MIDFIELD"() -> (w2704:u16)
                        n1545 = local read "N segments BORDER"() -> (w2707:u8)
                        n1546 = local read "Radius, mm CENTER"() -> (w2702:u16)
                        n1547 = local read "Cage diameter, mm"() -> (w2686:u16)
                        n1548 = property on="IO parameters string" class="Str"() -> ("Value"=w2687:string)  [unwired: 2 in, 2 out]
                        n1549 = property on="Bridge offset" class="DigNum (strict)"() -> ("Value"=w2662:sgl)  [unwired: 2 in, 2 out]
                        n1550 = property on="Bridge swap" class="Bool (strict)"() -> ("Value"=w2661:bool)  [unwired: 2 in, 2 out]
                        n1551 = property on="Data filtering" class="Ring (strict)"() -> ("Value"=w2621:u16)  [unwired: 2 in, 2 out]
                        n1552 = local read "Current User"() -> (w2625:string)
                        n1553 = property on="Name Prefix" class="Str"() -> ("Value"=w2644:string)  [unwired: 2 in, 2 out]
                        n1554 = Bundle By Name ("Geometrical parameters")(cluster=T47 {"N segments BORDER"=0, "Starting angle BORDER"=0, "N segments MIDFIELD"=0, "Starting angle MIDFIELD"=0, "Radius, mm MIDFIELD"=0, "Amount of central segments"=0, "Radius, mm CENTER"=0, "Bridge swap"=FALSE, "Bridge V. offset"=0.0, "Twisted neck"=FALSE, "Offset H."=0.0, "Zones configuration"=[], "IO parameters string"="[12,1,1,0,0,0]", "Cage diameter, mm"=180, "Name prefix"="SavedTrack", "Stop at"=0.0, "\"Stop at\" enabled"=FALSE, "Data filtering"=0} ("Parameters"), "N segments BORDER"=w2707, "Starting angle BORDER"=w2708, "N segments MIDFIELD"=w2706, "Starting angle MIDFIELD"=w2705, "Radius, mm MIDFIELD"=w2704, "Amount of central segments"=u8 1, "Radius, mm CENTER"=w2702, "Bridge V. offset"=w2662, "Bridge swap"=w2661, "Zones configuration"=w2688, "IO parameters string"=w2687, "Cage diameter, mm"=w2686, "Twisted neck"=w2653, "Offset H."=w2648, "Name prefix"=w2644, "Stop at"=w2638, "\"Stop at\" enabled"=w2635, "Data filtering"=w2621) -> (w2691:T47)
                        n1555 = global read "SW_Globals.vi" "Cluster of paths"() -> (w2715:T22)
                        n1556 = local read "Current User"() -> (w2699:string)
                        n1557 = call "SW_Get_save_paths.vi"("Input cluster of paths"=w2715, "Final file name prefix"=w2644) -> ("error out"=w2643:errorcluster, "Saved track name"=w2700:string, "Output cluster of paths"=w2632:T22)  [unwired: 2 in]
                        n1558 = Format Date/Time String(seconds (now)=w2698, UTC format=FALSE) -> (date/time string=w2697:string)  [unwired: 1 in]
                        n1559 = Flatten To JSON(enable LabVIEW extensions? (T)=TRUE, anything=w2691) -> (JSON string=w2694:string, 11:w2685:errorcluster)  [unwired: 1 in]
                        n1560 = Unbundle By Name(w2632) -> ("TDMS file reference"=w2675:refnum<k34>, "Path to the settings file"=w2671:path, "Recording settings output path"=w2629:path)
                        n1561 = call <vilib>:"Open Config Data.vi"("create file if necessary (T)"=TRUE, "configuration file path"=w2671) -> ("error out"=w2667:errorcluster, "refnum"=w2669:T5)  [unwired: 7 in, 1 out]
                        n1562 = call <vilib>:"Write Key (Boolean).vi"("section"=w2625, "error in (no error)"=w2667, "value"=w2661, "key"="Bridge swap?", "refnum"=w2669) -> ("error out"=w2665:errorcluster, "refnum out"=w2666:T5)  [unwired: 4 in, 1 out]
                        n1563 = call <vilib>:"Write Key (Double).vi"("use system decimal point (T)"=w2640, "precision (6)"=i16 2, "section"=w2625, "error in (no error)"=w2665, "value"=w2662, "key"="Bridge offset", "refnum"=w2666) -> ("error out"=w2655:errorcluster, "refnum out"=w2656:T5)  [unwired: 2 in, 1 out]
                        n1564 = call <vilib>:"Write Key (Boolean).vi"("section"=w2625, "error in (no error)"=w2655, "value"=w2653, "key"="Twisted neck", "refnum"=w2656) -> ("error out"=w2652:errorcluster, "refnum out"=w2651:T5)  [unwired: 4 in, 1 out]
                        n1565 = call <vilib>:"Write Key (Double).vi"("use system decimal point (T)"=w2640, "precision (6)"=i16 2, "section"=w2625, "error in (no error)"=w2652, "value"=w2648, "key"="Offset H.", "refnum"=w2651) -> ("error out"=w2647:errorcluster, "refnum out"=w2646:T5)  [unwired: 2 in, 1 out]
                        n1566 = call <vilib>:"Write Key (String).vi"("section"=w2625, "error in (no error)"=w2647, "value"=w2644, "key"="Name prefix", "refnum"=w2646) -> ("error out"=w2641:errorcluster, "refnum out"=w2642:T5)  [unwired: 4 in, 1 out]
                        n1567 = call <vilib>:"Write Key (Double).vi"("use system decimal point (T)"=w2640, "precision (6)"=i16 2, "section"=w2625, "error in (no error)"=w2641, "value"=w2638, "key"="Stop at", "refnum"=w2642) -> ("error out"=w2637:errorcluster, "refnum out"=w2636:T5)  [unwired: 2 in, 1 out]
                        n1568 = call <vilib>:"Write Key (Boolean).vi"("section"=w2625, "error in (no error)"=w2637, "value"=w2635, "key"="\"Stop at\" enabled", "refnum"=w2636) -> ("error out"=w2627:errorcluster, "refnum out"=w2624:T5)  [unwired: 4 in, 1 out]
                        n1569 = global write "SW_Globals.vi" "Cluster of paths"(w2632) -> ()
                        n1570 = Build Array(w2700, w2699, w2697, w2694) -> (w2696:string[])
                        n1571 = call <vilib>:"Write Key (U32).vi"("section"=w2625, "error in (no error)"=w2627, "value"=w2621, "key"="Data filtering", "refnum"=w2624) -> ("error out"=w2626:errorcluster, "refnum out"=w2623:T5)  [unwired: 4 in, 1 out]
                        n1572 = call <vilib>:"Close Config Data.vi"("error in (no error)"=w2626, "refnum"=w2623) -> ("error out"=w2657:errorcluster, "file path"=w2631:path)  [unwired: 8 in]
                        n1573 = Copy(9:TRUE ("overwrite (F)"), 10:w2629, 11:w2631) -> (0:w2628:errorcluster)  [unwired: 2 in, 2 out]
                        n1574 = Flush Queue(queue=w2719) -> (error out=w2717:errorcluster)  [unwired: 1 in, 2 out]
                        n1575 = TDMS Set Properties(5:w2696, 7:string[] ["Title", "Author", "DateTime", "Description", ""] ("property names"), 8:w2685, 11:w2675) -> (0:w2681:errorcluster, 3:w2684:refnum<k34>)  [unwired: 2 in, 2 out]
                        n1576 = for {
                          tunnel: w2684 -> [w2735]
                          tunnel: string[] ["X1_raw", "Y1_raw", "X2_raw", "Y2_raw"] ("Columns Names") -> [w2734] mode=indexing
                          tunnel: "Raw_data" ("group name in (Untitled)") -> [w2733]
                          tunnel: w2679 -> [w2732]
                          tunnel: w2680 -> [w2731]
                          tunnel: w2681 -> [w2730]
                          tunnel: [w2729] -> w2678
                          tunnel: [w2728] -> w2677
                          n1577 = TDMS Set Properties(5:w2731, 7:w2732, 8:w2730, 9:w2734, 10:w2733, 11:w2735) -> (0:w2728:errorcluster, 3:w2729:refnum<k34>)  [unwired: 2 out]
                        }
                        n1578 = for {
                          tunnel: string[] ["Absolute_timestamp", "Relative_timestamp", "R", "phi", "alpha", "X", "Y", "w", "Speed_mm_per_s", "Current_zone", "TTL_inputs", "TTL_outputs", "Zones_preference", "Frame_OK"] ("appended array") -> [w2727] mode=indexing
                          tunnel: "Data" ("group name in (Untitled)") -> [w2726]
                          tunnel: w2679 -> [w2725]
                          tunnel: w2680 -> [w2724]
                          tunnel: w2677 -> [w2723]
                          tunnel: w2678 -> [w2722]
                          tunnel: [w2721] -> w2676
                          tunnel: [w2720] -> _
                          n1579 = TDMS Set Properties(5:w2724, 7:w2725, 8:w2723, 9:w2727, 10:w2726, 11:w2722) -> (0:w2721:errorcluster, 3:w2720:refnum<k34>)  [unwired: 2 out]
                        }
                        n1580 = Merge Errors(w2628, w2717, w2643, w2676, w2657) -> (w2712:errorcluster)
                        n1581 = property on="Data filtering" class="Ring (strict)"(error in=w2712, "DisabledEnum"=T12."Disabled and Grayed Out" ("Disabled")) -> (error out=w2711:errorcluster)  [unwired: 1 in, 1 out]
                        n1582 = property on="Exit (recording)" class="Bool"(error in=w2711, "DisabledEnum"=T12."Enabled" ("Disabled")) -> (error out=w2658:errorcluster)  [unwired: 1 in, 1 out]
                        n1583 = property on="Additional recording settings" class="Bool (strict)"(error in=w2658, "DisabledEnum"=w2660) -> (error out=w2659:errorcluster)  [unwired: 1 in, 1 out]
                        n1584 = property on="Bridge swap" class="Bool (strict)"(error in=w2659, "DisabledEnum"=w2660) -> (error out=w2714:errorcluster)  [unwired: 1 in, 1 out]
                        n1585 = property on="Bridge offset" class="DigNum (strict)"(error in=w2714, "DisabledEnum"=w2660) -> (error out=w2713:errorcluster)  [unwired: 1 in, 1 out]
                        n1586 = global write "SW_Globals.vi" "Start time is set"(FALSE ("Start time is set")) -> ()
                      }
                    }
                    n1587 = Unbundle By Name(w2612) -> ("Recording now"=w2614:refnum<notifier>, "Has been recorded"=w2618:refnum<notifier>)
                    n1588 = Send Notification(notification=TRUE, notifier=w2614, error in (no error)=w2611) -> ()  [unwired: 2 out]
                    n1589 = Send Notification(notification=TRUE, notifier=w2618, error in (no error)=w2611) -> (error out=w2616:errorcluster)  [unwired: 1 out]
                    n1590 = property on="Record timestamp" class="DigNum (strict)"(error in=w2616, "DisabledEnum"=T12."Enabled" ("Disabled")) -> ()  [unwired: 1 in, 2 out]
                  }
                }
                n1591 = Subtract(x=w2595, y=w2599) -> (x-y=w2585:dbl)
                "Record timestamp" <- w2585
                n1592 = property on="Stop record at" class="DigNum (strict)"() -> ("Value"=w2584:dbl)  [unwired: 2 in, 2 out]
                n1593 = Subtract(x=w2584, y=w2585) -> (x-y=w2583:dbl)
                n1594 = Round Toward +Infinity(x=w2583) -> (ceil(x): smallest int >= x=w2586:dbl)
                n1595 = feedback-in #9(w2586) -> ()
                n1596 = feedback #9(0.0) -> (w2590:dbl)
                n1597 = Not Equal?(x=w2590, y=w2586) -> (x != y?=w2589:bool)
                n1598 = property on="\"Stop at\" enabled" class="Bool (strict)"() -> ("Value"=w2587:bool)  [unwired: 2 in, 2 out]
                n1599 = And(x=w2587, y=w2589) -> (x .and. y?=w2588:bool)
                n1600 = Greater Or Equal?(x=w2585, y=w2584) -> (x >= y?=w2593:bool)
                n1601 = case shown="True" w2588 {
                  tunnel: w2586 -> [_ w2602]
                  frame False {
                  }
                  frame True {
                    n1602 = Format Date/Time String() -> ()  [unwired: 3 in, 1 out]
                    n1603 = Format Date/Time String(time format string (%c)="%H:%M:%S" ("format string"), seconds (now)=w2602, UTC format=TRUE) -> (date/time string=w2601:string)
                    n1604 = property on="Additional record settings" class="Bool (strict)"("BoolText.Text"=w2601) -> ()  [unwired: 2 in, 2 out]
                  }
                }
                n1605 = And(x=w2593, y=w2587) -> (x .and. y?=w2592:bool)
                n1606 = case shown="True" w2592 {
                  frame False {
                  }
                  frame True {
                    n1607 = property on="Record/Stop" class="Bool (strict)"("Val(Sgnl)"=FALSE ("Record/Stop")) -> ()  [unwired: 2 in, 2 out]
                  }
                }
              }
            }
            n1608 = disable-structure shown="Disabled" {
              disable-tunnel: w2212 -> [w2350 _]
              disable-tunnel: w2211 -> [w2349 _]
              disable-tunnel: w2210 -> [w2348 _]
              disable-tunnel: w2209 -> [w2347 _]
              frame Disabled {
                w2311 = FALSE ("use system decimal point (T)")
                w2302 = "\t"
                w2320 = i16 3 ("precision (6)")
                n1609 = property on="Mouse speed digi" class="DigNum (strict)"() -> ("Value"=w2301:dbl)  [unwired: 2 in, 2 out]
                n1610 = Number To Fractional String(use system decimal point (T)=TRUE, number=w2301, precision (6)=i16 3) -> (F-format string=w2298:string)  [unwired: 1 in]
                n1611 = Index Array "R"(array=w2347, index=6) -> (element=w2305:string)
                n1612 = Index Array "phi"(array=w2347, index=7) -> (element=w2322:string)
                n1613 = Fract/Exp String To Number(use system decimal point (T)=FALSE, string=w2322) -> (number=w2315:dbl)  [unwired: 2 in, 1 out]
                n1614 = Greater Than 0?(x=w2315) -> (x > 0?=w2319:bool)
                n1615 = Select(t=-180.0, s=w2319, f=180.0) -> (s? t:f=w2316:dbl)
                n1616 = Add(x=w2316, y=w2315) -> (x+y=w2314:dbl)
                n1617 = Select(t=w2314, f=w2315) -> (s? t:f=w2324:dbl)  [unwired: 1 in]
                n1618 = Fract/Exp String To Number(use system decimal point (T)=w2311, string=w2305) -> (number=w2313:dbl)  [unwired: 2 in, 1 out]
                n1619 = global read "SW_Globals.vi" "Current zone"() -> (w2308:u8)
                n1620 = Negate(x=w2350) -> (-x=w2335:dbl)
                n1621 = Negate(x=w2349) -> (-x=w2336:dbl)
                n1622 = Number To Fractional String(use system decimal point (T)=FALSE, number=w2324, precision (6)=w2320) -> (F-format string=w2309:string)  [unwired: 1 in]
                n1623 = Number To Fractional String(use system decimal point (T)=w2311, number=w2313, precision (6)=i16 3) -> (F-format string=w2310:string)  [unwired: 1 in]
                n1624 = property on="Record timestamp" class="DigNum (strict)"() -> ("Value"=w2337:dbl)  [unwired: 2 in, 2 out]
                n1625 = Select(t=w2335, f=w2350) -> (s? t:f=w2328:dbl)  [unwired: 1 in]
                n1626 = Select(t=w2336, f=w2349) -> (s? t:f=w2329:dbl)  [unwired: 1 in]
                n1627 = Number To Fractional String(use system decimal point (T)=FALSE, number=w2329, precision (6)=w2320) -> (F-format string=w2340:string)  [unwired: 1 in]
                n1628 = Number To Fractional String(use system decimal point (T)=FALSE, number=w2328, precision (6)=w2320) -> (F-format string=w2339:string)  [unwired: 1 in]
                n1629 = Number To Fractional String(use system decimal point (T)=FALSE, number=w2308, precision (6)=i16 0) -> (F-format string=w2303:string)  [unwired: 1 in]
                n1630 = Greater Than 0?(x=w2348) -> (x > 0?=w2334:bool)
                n1631 = Select(t=-180.0, s=w2334, f=180.0) -> (s? t:f=w2331:dbl)
                n1632 = Format Date/Time String(time format string (%c)="%H:%M:%S%.;%3u " ("format string"), seconds (now)=w2337, UTC format=TRUE) -> (date/time string=w2344:string)
                n1633 = Add(x=w2331, y=w2348) -> (x+y=w2330:dbl)
                n1634 = Select(t=w2330, f=w2348) -> (s? t:f=w2327:dbl)  [unwired: 1 in]
                n1635 = Number To Fractional String(use system decimal point (T)=FALSE, number=w2327, precision (6)=w2320) -> (F-format string=w2338:string)  [unwired: 1 in]
                n1636 = Concatenate Strings(w2344, w2302, w2340, w2302, w2339, w2302, w2338, w2302, w2310, w2302, w2309, w2302, w2298, w2302, w2303, "\r\n") -> (w2294:string)
                n1637 = property on="Output to the external terminal" class="Str"("Value"=w2294) -> ()  [unwired: 2 in, 2 out]
                n1638 = property on="Streaming" class="Bool (strict)"() -> ("Value"=w2295:bool)  [unwired: 2 in, 2 out]
                n1639 = case shown="True" w2295 {
                  tunnel: [w2359 w2363] -> _
                  tunnel: w2294 -> [_ w2362]
                  tunnel: [_ w2361] -> w2296
                  frame False {
                    n1640 = property on="Serial OUT name" class="VISAName"() -> ("Value"=w2359:refnum<visa-resource-name>)  [unwired: 2 in, 2 out]
                  }
                  frame True {
                    n1641 = VISA Write(write buffer=w2362) -> (VISA resource name out=w2363:refnum<visa-resource-name>, return count=w2360:u32, error out=w2361:errorcluster)  [unwired: 2 in]
                  }
                }
                n1642 = case shown="Error" w2296 {
                  tunnel: [TRUE ("write status") FALSE ("write status")] -> w2297
                  frame No Error {
                  }
                  frame Error {
                    w2356 = u32 0
                    n1643 = feedback #10(w2356) -> (w2353:u32)
                    n1644 = Increment(x=w2353) -> (x+1=w2355:u32)
                    n1645 = Greater?(x=w2355, y=u32 15) -> (0:w2357:bool)
                    n1646 = Select(t=w2356, s=w2357, f=w2355) -> (s? t:f=w2354:u32)
                    n1647 = feedback-in #10(w2354) -> ()
                  }
                }
                "write status" <- w2297
              }
              frame Enabled {
              }
            }
            n1648 = Or(x="Reset barplot", y=w2272) -> (x .or. y?=w2273:bool)
            n1649 = case shown="True" w2272 {
              frame False {
              }
              frame True {
                w2378 = waveform(dbl)[] [] ("History Data")
                n1650 = property on="Mouse speed" class="WFChart (strict)"("History Data"=w2378) -> ()  [unwired: 2 in, 2 out]
                n1651 = property on="Mouse speed 2" class="WFChart (strict)"("History Data"=w2378) -> ()  [unwired: 2 in, 2 out]
              }
            }
            n1652 = case shown="True" w2273 {
              frame False {
              }
              frame True {
                n1653 = global read "SW_Globals.vi" "Speed distribution array"() -> (w2389:u32[])
                n1654 = global read "SW_Globals.vi" "Zones allocation array"() -> (w2392:i32[])
                n1655 = global read "SW_Globals.vi" "Run Lengts distribution array"() -> (w2386:u32[])
                n1656 = global read "SW_Globals.vi" "Run Times distribution array"() -> (w2379:u32[])
                n1657 = Array Size(array=w2392) -> (size(s)=w2394:i32)
                n1658 = Array Size(array=w2389) -> (size(s)=w2387:i32)
                n1659 = Array Size(array=w2379) -> (size(s)=w2380:i32)
                n1660 = Array Size(array=w2386) -> (size(s)=w2385:i32)
                n1661 = Initialize Array(0 ("element"), w2394) -> (w2391:i32[])
                n1662 = Initialize Array(u32 0 ("element"), w2387) -> (w2390:u32[])
                n1663 = global write "SW_Globals.vi" "Zones allocation array"(w2391) -> ()
                n1664 = global write "SW_Globals.vi" "Speed distribution array"(w2390) -> ()
                n1665 = Initialize Array(u32 0 ("element"), w2380) -> (w2382:u32[])
                n1666 = Initialize Array(u32 0 ("element"), w2385) -> (w2383:u32[])
                n1667 = global write "SW_Globals.vi" "Run Times distribution array"(w2382) -> ()
                n1668 = global write "SW_Globals.vi" "Run Lengts distribution array"(w2383) -> ()
              }
            }
          }
          frame "Analysis" {
            n1669 = Unbundle By Name(w2769) -> ("Has been recorded"=w2771:refnum<notifier>)
            n1670 = disable-structure shown="Enabled" {
              frame Enabled {
                n1671 = event shown="[2] \"Back to Settings\": Value Change" {
                  selector: _ -> [_ _ _]
                  dyn-events: _ -> [_ _ _]
                  timeout: 0 -> [_ _ _]
                  event Timeout {
                    n1672 = event-data() -> ()  [unwired: 1 in, 3 out]
                  }
                  event "Play/Pause": Value Change {
                    n1673 = event-data() -> ("NewVal"=w2786:bool)  [unwired: 1 in, 5 out]
                    n1674 = case shown="True" w2786 {
                      frame False {
                        n1675 = property on="Back to Settings" class="Bool (strict)"("DisabledEnum"=T12."Enabled" ("Disabled")) -> ()  [unwired: 2 in, 2 out]
                      }
                      frame True {
                        n1676 = property on="Back to Settings" class="Bool (strict)"("DisabledEnum"=T12."Disabled and Grayed Out" ("Disabled")) -> ()  [unwired: 2 in, 2 out]
                      }
                    }
                  }
                  event "Back to Settings": Value Change {
                    n1677 = event-data() -> ("NewVal"=w2789:bool)  [unwired: 1 in, 5 out]
                    n1678 = case shown="True" w2789 {
                      frame False {
                      }
                      frame True {
                        w2801 = FALSE ("Visible")
                        w2821 = enum32{"Settings", "Recording", "Analysis"}."Settings" ("Main tab control")
                        w2817 = enum32{"Settings", "Recording", "Analysis"}."Recording" ("Main tab control")
                        w2808 = enum32{"Settings", "Recording", "Analysis"}."Analysis" ("Main tab control")
                        n1679 = property on="Diagram at recording" class="Pict" props=["Bounds"]() -> (error out=w2805:errorcluster)  [unwired: 2 in, 2 out]
                        n1680 = property on="Main tab control" class="TabCtl (strict)"(error in=w2805, "Value"=w2808) -> (error out=w2812:errorcluster, "Pages"=w2807:refnum<vi>[])  [unwired: 1 in, 1 out]
                        n1681 = To Long Integer(number=w2808) -> (32bit integer=w2809:i32)
                        n1682 = Index Array(array=w2807, index=w2809) -> (element=w2810:refnum<vi>)
                        n1683 = property class="Page"(reference=w2810, error in=w2812, "PageEnb"=T32."Page Disabled & Grayed" ("Page Enabled State")) -> (error out=w2819:errorcluster)  [unwired: 1 out]
                        n1684 = property on="Main tab control" class="TabCtl (strict)"(error in=w2819, "Value"=w2817) -> (error out=w2813:errorcluster, "Pages"=w2818:refnum<vi>[])  [unwired: 1 in, 1 out]
                        n1685 = To Long Integer(number=w2817) -> (32bit integer=w2816:i32)
                        n1686 = Index Array(array=w2818, index=w2816) -> (element=w2815:refnum<vi>)
                        n1687 = property class="Page"(reference=w2815, error in=w2813, "PageEnb"=T32."Page Disabled & Grayed" ("Page Enabled State")) -> (error out=w2826:errorcluster)  [unwired: 1 out]
                        n1688 = property on="Main tab control" class="TabCtl (strict)"(error in=w2826, "Value"=w2821) -> (error out=w2825:errorcluster, "Pages"=w2820:refnum<vi>[])  [unwired: 1 in, 1 out]
                        n1689 = To Long Integer(number=w2821) -> (32bit integer=w2822:i32)
                        n1690 = Index Array(array=w2820, index=w2822) -> (element=w2823:refnum<vi>)
                        n1691 = property class="Page"(reference=w2823, error in=w2825, "PageEnb"=T32."Page Enabled" ("Page Enabled State")) -> (error out=w2806:errorcluster)  [unwired: 1 out]
                        n1692 = global read "SW_Globals.vi" "Cluster of paths"() -> (w2804:T22)
                        n1693 = property on="Back to Settings" class="Bool (strict)"(error in=w2806, "Visible"=w2801, "Value"=w2801) -> (error out=w2791:errorcluster)  [unwired: 1 in, 1 out]
                        n1694 = Unbundle By Name(w2804) -> ("Path to the settings file"=w2803:path)
                        n1695 = property on="Pane" class="Pane"(error in=w2791) -> (error out=w2793:errorcluster, "Decos[]"=w2794:refnum<vi>[])  [unwired: 1 in, 1 out]
                        n1696 = Index Array(array=w2794, index=0) -> (element=w2799:refnum<vi>)
                        n1697 = property class="Decor"(reference=w2799, error in=w2793, "Visible"=FALSE) -> (error out=w2792:errorcluster)  [unwired: 1 out]
                        n1698 = Index Array(array=w2794, index=2) -> (element=w2796:refnum<vi>)
                        n1699 = property class="Decor"(reference=w2796, error in=w2792, "Visible"=TRUE) -> (error out=w2790:errorcluster)  [unwired: 1 out]
                        n1700 = call <vilib>:"Open Config Data.vi"("error in (no error)"=w2790, "configuration file path"=w2803) -> ("refnum"=w2802:T5)  [unwired: 7 in, 2 out]
                        n1701 = local write "Settings file refnum out"(w2802) -> ()
                      }
                    }
                  }
                }
              }
              frame Disabled {
              }
            }
            n1702 = Unbundle By Name(w2769) -> ("Data loaded"=w2778:refnum<notifier>)
            n1703 = Get Notifier Status(notifier=w2771) -> (current notification=w2768:bool)  [unwired: 1 in, 4 out]
            n1704 = Get Notifier Status(notifier=w2778) -> (current notification=w2776:bool)  [unwired: 1 in, 4 out]
            n1705 = Not(x=w2768) -> (.not. x?=w2770:bool)
            n1706 = Or(x=w2770, y=w2776) -> (x .or. y?=w2772:bool)
            n1707 = And(x=w2776, y="Play/Pause") -> (x .and. y?=w2779:bool)
            n1708 = global read "SW_Globals.vi" "Density map with no zones and with full track"() -> (w2753:picture)
            n1709 = Not(x="Play/Pause") -> (.not. x?=w2774:bool)
            n1710 = global read "SW_Globals.vi" "Density map with zones and full track"() -> (w2752:picture)
            n1711 = And(x=w2772, y=w2774) -> (x .and. y?=w2773:bool)
            n1712 = global read "SW_Globals.vi" "Density map with zones"() -> (w2754:picture)
            n1713 = global read "SW_Globals.vi" "Full track with no zones"() -> (w2757:picture)
            n1714 = global read "SW_Globals.vi" "Density map no zones"() -> (w2755:picture)
            n1715 = global read "SW_Globals.vi" "Full track with zones"() -> (w2756:picture)
            n1716 = global read "SW_Globals.vi" "Diagram no zones"() -> (w2759:picture)
            n1717 = case shown="True" w2773 {
              tunnel: w2769 -> [_ w2829]
              frame False {
              }
              frame True {
                n1718 = case "Open new file" shown="True" "Open File" {
                  tunnel: w2829 -> [_ w2833]
                  frame False {
                  }
                  frame True {
                    n1719 = global read "SW_Globals.vi" "Cluster of paths"() -> (w2834:T22)
                    n1720 = Unbundle By Name(w2834) -> ("Path to TDMS file"=w2844:path)
                    n1721 = Strip Path(path=w2844) -> (stripped path=w2843:path)  [unwired: 1 out]
                    n1722 = Strip Path(path=w2843) -> (stripped path=w2840:path)  [unwired: 1 out]
                    n1723 = call "File Dialog"("start path"=w2840, "button label"="Open track", "pattern (all files)"="*.csv; *.tdms") -> ("selected path"=w2835:path, "exists"=w2839:bool, "cancelled"=w2837:bool, "error out"=w2832:errorcluster)  [unwired: 9 in]
                    n1724 = Not(x=w2837) -> (.not. x?=w2838:bool)
                    n1725 = And(x=w2839, y=w2838) -> (x .and. y?=w2836:bool)
                    n1726 = case shown="True" w2836 {
                      tunnel: w2835 -> [_ w2849]
                      tunnel: w2834 -> [_ w2848]
                      tunnel: w2833 -> [_ w2846]
                      tunnel: w2832 -> [_ _]
                      frame False {
                      }
                      frame True {
                        n1727 = flat-sequence {
                          tunnel: w2849 -> [w2863]
                          tunnel: [w2862] -> w2847
                          tunnel: [w2851] -> w2845
                          tunnel: w2848 -> [w2869]
                          tunnel: w2847 -> [w2868]
                          tunnel: w2845 -> [w2866]
                          tunnel: w2846 -> [w2876]
                          frame #0 {
                            n1728 = call <vilib>:"Get File Extension.vi"("file"=w2863) -> ("filename without extension"=w2856:string, "lowercase file extension"=w2855:string)  [unwired: 6 in, 3 out]
                            n1729 = Concatenate Strings(w2856, ".trset" ("string")) -> (w2864:string)
                            n1730 = Strip Path(path=w2863) -> (stripped path=w2857:path)  [unwired: 1 out]
                            n1731 = Concatenate Strings(w2856, ".tdms" ("string")) -> (w2859:string)
                            n1732 = Concatenate Strings(w2856, ".csv" ("string")) -> (w2858:string)
                            n1733 = Build Path(base path=w2857, name or relative path=w2864) -> (appended path=w2862:path)
                            "Settings file path" <- w2862
                            n1734 = Build Path(base path=w2857, name or relative path=w2859) -> (appended path=w2852:path)
                            n1735 = Build Path(base path=w2857, name or relative path=w2858) -> (appended path=w2850:path)
                            n1736 = Equal?(x=w2855, y="tdms") -> (x = y?=w2853:bool)
                            n1737 = Select(t=w2852, s=w2853, f=w2850) -> (s? t:f=w2851:path)
                            "Track path" <- w2863
                          }
                          frame #1 {
                            n1738 = Bundle By Name(cluster=w2869, "Path to TDMS file"=w2866, "Recording settings output path"=w2868) -> (w2867:T22)
                            n1739 = global write "SW_Globals.vi" "Cluster of paths"(w2867) -> ()
                          }
                          frame #2 {
                            n1740 = Unbundle By Name(w2876) -> ("(Final) Data file is saved"=w2872:refnum<notifier>, "Data loaded"=w2875:refnum<notifier>, "Has been recorded"=w2870:refnum<notifier>)
                            n1741 = Send Notification(notification=TRUE, notifier=w2872) -> ()  [unwired: 1 in, 2 out]
                            n1742 = Send Notification(notification=FALSE, notifier=w2875) -> ()  [unwired: 1 in, 2 out]
                            n1743 = Send Notification(notification=TRUE, notifier=w2870) -> ()  [unwired: 1 in, 2 out]
                          }
                        }
                      }
                    }
                  }
                }
                n1744 = property on="Open File" class="Bool"("DisabledEnum"=T12."Enabled" ("Disabled")) -> (error out=w2827:errorcluster)  [unwired: 2 in, 1 out]
                n1745 = property on="Timeline" class="Slide (strict)"(error in=w2827, "DisabledEnum"=T12."Disabled and Grayed Out" ("Disabled")) -> ()  [unwired: 1 in, 2 out]
              }
            }
            n1746 = global read "SW_Globals.vi" "Diagram"() -> (w2758:picture)
            n1747 = Build Array(w2759, w2758, w2757, w2756, w2755, w2754, w2753, w2752) -> (w2765:picture[])
            n1748 = Index Array(array=w2765, index="Map index (analysis)") -> (element=w2764:picture)
            n1749 = case shown="False" w2779 {
              tunnel: w2764 -> [w2877 w2927]
              tunnel: "Zones (analysis)" -> [_ w2926]
              tunnel: [w2877 w2925] -> w2777
              tunnel: w2767 -> [_ w2906]
              frame False {
              }
              frame True {
                n1750 = disable-structure shown="Disabled" {
                  frame Disabled {
                    (unwired) "%<%H:%M:%S%3u%p%d.%m.%Y>T" ("format string")
                    n1751 = Get Date/Time In Seconds() -> (seconds since 1Jan1904=w2943:timestamp)
                    n1752 = Scan From String(default 1=w2943) -> ()  [unwired: 5 in, 3 out]
                  }
                  frame Enabled {
                  }
                }
                n1753 = Divide(x=u32 1000, y=w2906) -> (x/y=w2908:dbl)
                n1754 = Multiply(x=w2908, y="Trace in analysis, s") -> (x*y=w2901:dbl)
                n1755 = local read "Absolute timestamp (rec)"() -> (w2915:dbl[])
                n1756 = local read "Relative timestamp (rec)"() -> (w2923:dbl[])
                n1757 = local read "alpha rot. angle"() -> (w2938:dbl[])
                n1758 = local read "Index of the last recorded timepoint"() -> (w2919:i32)
                n1759 = local read "TTL outputs"() -> (w2898:u8[])
                n1760 = local read "TTL inputs"() -> (w2899:u8[])
                n1761 = local read "Zones preference array (loaded)"() -> (w2911:dbl[][])
                n1762 = property on="Timeline" class="Slide (strict)"("DisabledEnum"=T12."Enabled" ("Disabled")) -> (error out=w2916:errorcluster)  [unwired: 2 in, 1 out]
                n1763 = property on="Open File" class="Bool"(error in=w2916, "DisabledEnum"=T12."Disabled and Grayed Out" ("Disabled")) -> ()  [unwired: 1 in, 2 out]
                n1764 = local read "X coord"() -> (w2940:dbl[])
                n1765 = local read "Y coord"() -> (w2939:dbl[])
                n1766 = feedback #11(0.0125 ("String")) -> (w2932:dbl)
                n1767 = Select(t=FALSE, s=w2926, f=TRUE) -> (s? t:f=w2884:bool)
                n1768 = feedback #12(0) -> (w2897:u32)
                n1769 = Index Array(array=w2938, index=w2897) -> (element=w2879:dbl)
                n1770 = Index Array(array=w2915, index=w2897) -> (element=w2914:dbl)
                n1771 = Index Array(array=w2899, index=w2897) -> (element=w2887:u8)
                n1772 = Index Array(array=w2898, index=w2897) -> (element=w2886:u8)
                n1773 = Index Array(array=w2923, index=w2897) -> (element=w2882:dbl)
                n1774 = feedback-in #11(w2882) -> ()
                n1775 = Add(x=w2887, y=w2886) -> (x+y=w2885:u8)
                n1776 = property on="Recorded timestamp" class="DigNum (strict)"("Value"=w2882) -> ()  [unwired: 2 in, 2 out]
                n1777 = Subtract(x=w2882, y=w2932) -> (x-y=w2931:dbl)
                n1778 = Index Array(array=w2911, index (row)=w2897) -> (element=→"Zones allocation (normalized) in analysis":dbl[])  [unwired: 1 in]
                n1779 = Index Array(array=w2940, index=w2897) -> (element=w2881:dbl)
                n1780 = Index Array(array=w2939, index=w2897) -> (element=w2880:dbl)
                n1781 = Number To Boolean Array(number=w2885) -> (Boolean array=w2888:bool[])
                n1782 = To Time Stamp(1:w2914) -> (0:w2913:timestamp)
                n1783 = property on="Recorded at time" class="AbsTime (strict)"("Value"=w2913) -> ()  [unwired: 2 in, 2 out]
                n1784 = call "FL_Calc_speed_on_the_fly.vi"("Y coord, mm"=w2880, "X coord, mm"=w2881, "Time per frame, s"=w2931) -> ("Mouse speed, mm/s"=w2929:dbl)
                "Mouse speed digi 2" <- w2929
                n1785 = To Time Stamp(1:w2882) -> (0:w2933:timestamp)
                n1786 = Build Array(w2929) -> (w2934:dbl[])
                n1787 = Index Array(array=w2888, index=3) -> (element=→"TTL IO 4 (analysis)":bool)
                n1788 = Index Array(array=w2888, index=0) -> (element=→"TTL IO 1 (analysis)":bool)
                n1789 = Index Array(array=w2888, index=1) -> (element=→"TTL IO 2 (analysis)":bool)
                n1790 = Index Array(array=w2888, index=2) -> (element=→"TTL IO 3 (analysis)":bool)
                n1791 = Bundle By Name("t0"=w2933, "Y"=w2934) -> (→"Mouse speed 2":waveform(dbl))  [unwired: 1 in]
                n1792 = feedback #13(u16 3 ("Value")) -> (w2905:u16)
                n1793 = event shown="[1] \"Timeline\": Value Change" {
                  selector: _ -> [_ _ _]
                  dyn-events: _ -> [_ _ _]
                  timeout: 1 -> [_ _ _]
                  tunnel: w2882 -> [w2952 _ _]
                  tunnel: w2897 -> [w2951 _ w2964]
                  tunnel: [w2950 w2962 w2964] -> w2922
                  tunnel: w2923 -> [_ _ _]
                  tunnel: w2919 -> [_ w2955 _]
                  tunnel: [w2944 w2953 w2963] -> w2903
                  tunnel: w2905 -> [_ w2953 w2963]
                  event Timeout {
                    n1794 = event-data() -> ()  [unwired: 1 in, 3 out]
                    n1795 = property on="Timeline" class="Slide (strict)"("Value"=w2952) -> ()  [unwired: 2 in, 2 out]
                    n1796 = property on="Speed" class="Ring (strict)"() -> ("RingText.Text"=w2948:string, "Strings []"=w2949:string[], "StringsAndValues[]"=w2946:T55)  [unwired: 2 in, 2 out]
                    n1797 = Search 1D Array(1D array=w2949, element=w2948) -> (index of element=w2947:i32)  [unwired: 1 in]
                    n1798 = Index Array(array=w2946, index=w2947) -> (element=w2945:cluster{"String":string, "Value":u16})
                    n1799 = Unbundle(w2945) -> ("Value"=w2944:u16)  [unwired: 1 out]
                    n1800 = Add(x=w2944, y=w2951) -> (x+y=w2950:u32)
                  }
                  event "Timeline": Value Change {
                    n1801 = event-data() -> ("NewVal"=w2960:dbl)  [unwired: 1 in, 5 out]
                    n1802 = property on="Timeline" class="Slide (strict)"() -> ("Scale.Maximum"=w2961:dbl, "Scale.Minimum"=w2959:dbl)  [unwired: 2 in, 2 out]
                    n1803 = Subtract(x=w2960, y=w2959) -> (x-y=w2958:dbl)
                    n1804 = Subtract(x=w2961, y=w2959) -> (x-y=w2957:dbl)
                    n1805 = Divide(x=w2958, y=w2957) -> (x/y=w2956:dbl)
                    "ceil(x): smallest int >= x" <- w2956
                    n1806 = Multiply(x=w2956, y=w2955) -> (x*y=w2954:dbl)
                    n1807 = To Unsigned Long Integer(number=w2954) -> (unsigned 32bit integer=w2962:u32)
                  }
                  event "Multiplyer of chart RX 2": Value Change {
                    n1808 = event-data() -> ("NewVal"=w2965:u8)  [unwired: 1 in, 5 out]
                    n1809 = property on="Mouse speed 2" class="WFChart (strict)"() -> (error out=w2967:errorcluster, "XScale.Maximum"=w2970:dbl)  [unwired: 2 in, 1 out]
                    n1810 = Multiply(x=w2965, y=10.0) -> (x*y=w2966:dbl)
                    n1811 = Subtract(x=w2970, y=w2966) -> (x-y=w2968:dbl)
                    n1812 = property on="Mouse speed 2" class="WFChart (strict)"(error in=w2967, "XScale.Minimum"=w2968) -> ()  [unwired: 1 in, 2 out]
                  }
                }
                n1813 = feedback-in #13(w2903) -> ()
                n1814 = Greater Or Equal?(x=w2922, y=w2919) -> (x >= y?=w2912:bool)
                n1815 = Divide(x=w2903, y=u16 3) -> (x/y=w2900:dbl)
                n1816 = Select(t=u32 0, s=w2912, f=w2922) -> (s? t:f=w2921:u32)
                n1817 = feedback-in #12(w2921) -> ()
                n1818 = property on="Diagram at analysis" class="Pict"() -> ("Bounds"=w2942:T19)  [unwired: 2 in, 2 out]
                n1819 = local read "Pixels per mm"() -> (w2941:dbl)
                n1820 = Divide(x=w2901, y=w2900) -> (x/y=w2878:dbl)
                n1821 = Round To Nearest(number=w2878) -> (nearest integer value=w2883:dbl)
                n1822 = call "SW_Draw_mouse_br.vi"("Input picture (background)"=w2927, "Size of the image"=w2942, "Pixels per mm"=w2941, "Mouse coord cartesian X, mm"=w2881, "Mouse coord cartesian Y, mm"=w2880, "Mouse angle of rotation, deg"=w2879, "Show mouse lineout"=w2884, "Trace length, samples"=w2883) -> ("Output picture (with mouse overlay)"=w2925:picture)  [unwired: 6 in, 1 out]
              }
            }
            "Diagram at analysis" <- w2777
            n1823 = event shown="[1] \"Zones (analysis)\", \"Show full track (analysis)\", \"Show heatmap (analysis)\": Value Change" {
              selector: _ -> [_ _]
              dyn-events: _ -> [_ _]
              timeout: 0 -> [_ _]
              tunnel: "Zones (analysis)" -> [_ w2784]
              tunnel: "Show full track (analysis)" -> [_ w2783]
              tunnel: "Show heatmap (analysis)" -> [_ w2781]
              event Timeout {
                n1824 = event-data() -> ()  [unwired: 1 in, 3 out]
              }
              event "Zones (analysis)", "Show full track (analysis)", "Show heatmap (analysis)": Value Change {
                n1825 = event-data() -> ()  [unwired: 1 in, 6 out]
                n1826 = Build Array(w2784, w2783, w2781) -> (w2782:bool[])
                n1827 = Boolean Array To Number(Boolean array=w2782) -> (number=w2780:u32)
                n1828 = property on="Map index (analysis)" class="DigNum (strict)"("Value"=w2780) -> ()  [unwired: 2 in, 2 out]
              }
            }
          }
        }
        n1829 = Get Notifier Status(notifier=w1519, error in (no error)=w1520) -> (current notification=w1521:bool)  [unwired: 4 out]
        n1830 = Or(x="Stop Button", y=w1521) -> (x .or. y?=w1522:bool)
        n1831 = node-c288() -> ()  [unwired: 1 in, 1 out]
      }
      n1832 = node-c288(w1514) -> ()  [unwired: 1 out]
    }
    frame Enabled {
    }
  }
